vi "Position_TOTAL_R22.vi"(5 "Distance Between \nCameras  (*unit)":sgl=2.5) -> (12 "dX, dY\nLeft Cam":cluster{"X":sgl[], "Y":sgl[]}={"X"=[-5.750775, -4.1849813, -3.081379, -2.0098581, 0.0], "Y"=[7.9585915, 7.9595685, 7.960258, 7.960927, 0.0]}, 13 "Position Valid":bool=TRUE, 14 "Left Camera Real Coordinates":cluster{"X":sgl, "Y":sgl}={"X"=7.9602513, "Y"=5.592073}, 16 "dX, dY\nRight Cam":cluster{"X":sgl[], "Y":sgl[]}={"X"=[-7.3032045, -5.737411, -4.6338086, -3.5622878, -1.5524296], "Y"=[7.2714148, 7.2723923, 7.2730813, 7.273751, -0.68717635]}, 18 "Robot Coordinates":cluster{"X":sgl, "Y":sgl}={"X"=7.616663, "Y"=6.3682876}, 19 "Orietnation\n(current)":sgl=-23.843685 format="%#_13g")   [LabVIEW 2015]
uses:
  <vilib>/Analysis/coordinate.llb/2D Cartesian Coordinate Rotation (Array).vi
  <vilib>/myRIO/Common/Instrument Driver Framework/myRIO v1.0/DIO/vis/myRIO v1.0 Close DIO.vi
  <vilib>/myRIO/Common/Instrument Driver Framework/myRIO v1.0/DIO/vis/myRIO v1.0 Unreserve DIO.vi
  <vilib>/myRIO/Common/Instrument Driver Framework/myRIO v1.0/DIO/vis/myRIO v1.0 Build MUX Configuration DIO.vi
  <vilib>/myRIO/Common/Instrument Driver Framework/myRIO v1.0/Resource Manager/vis/myRIO v1.0 Unreserve Channel List.vi
  <vilib>/myRIO/Common/Instrument Driver Framework/myRIO v1.0/Resource Manager/vis/myRIO v1.0 Create Configuration List.vi
  <vilib>/myRIO/Common/Instrument Driver Framework/myRIO v1.0/Resource Manager/vis/myRIO v1.0 Unreserve Channel.vi
  <vilib>/myRIO/Common/Instrument Driver Framework/myRIO v1.0/Resource Manager/vis/myRIO v1.0 Build Mutex Name.vi
  <vilib>/Instr/_visa.llb/VISA Configure Serial Port (Instr).vi
  <vilib>/myRIO/Common/Instrument Driver Framework/myRIO v1.0/DIO/vis/myRIO v1.0 Shutdown DIO.vi
  <vilib>/Utility/error.llb/Error Cluster From Error Code.vi
  <vilib>/myRIO/Common/Instrument Driver Framework/myRIO v1.0/Resource Manager/vis/myRIO v1.0 Configure IO.vi
  <vilib>/myRIO/Common/Instrument Driver Framework/Utilities/vis/Configuration Manager.vi
  <vilib>/myRIO/Common/Instrument Driver Framework/Utilities/vis/IO Manager.vi
  <vilib>/myRIO/Common/Instrument Driver Framework/myRIO v1.0/myRIO v1.0 Close.vi
  <vilib>/Analysis/NI_AALPro.lvlib
  <vilib>/myRIO/Instrument Drivers/Onboard IO/DIO/DIO.lvlib
panel:
  out "Scale Based\nWeight":sgl format="%#_13g"
  in  "Triangle Based\nWeight":sgl=0.4 format="%#_13g"
  out "Current Cam State - R":T1(ring)=enum."Normal - 5"
  out "Current Cam State - L":T1(ring)=enum."Normal - 5"
  out "Valid Beacon Sets_":bool[](array[boolean])=[TRUE, TRUE, TRUE, TRUE, FALSE]
  in  "Distance Threshold\nRef Triangles (*unit)":sgl=30.0
  out "dA2 4":sgl=9.6935425 format="%#_13g"
  out "dA2 2":sgl=9.6935425 format="%#_13g"
  out "dA2 3":sgl=9.6935425 format="%#_13g"
  out "Beacon Scales - Left":sgl[](array[numeric])=[76.306, 116.841255, 157.35043, 195.67218, 0.0]
  out "Beacon Scales - Right":sgl[](array[numeric])=[76.306, 116.841255, 157.35043, 195.67218, 0.0]
  in  "New Orientation \nThreshold":sgl=10.0
  in  "Moving Average\nWindow Length":u8=2
  out "Current Recovery State -L":enum16{"Generic Sweep", "Recovery Search"}(ring)=enum."Recovery Search"
  out "Current Move Delta - L 2":u16
  out "Next Recovery State - Left":enum16{"Generic Sweep", "Recovery Search"}(ring)=enum."Recovery Search"
  out "Next Recovery State - Right":enum16{"Generic Sweep", "Recovery Search"}(ring)=enum."Recovery Search"
  out "Current Recovery State - Right":enum16{"Generic Sweep", "Recovery Search"}(ring)=enum."Recovery Search"
  in  "Initial Recovery State  - Right":enum16{"Generic Sweep", "Recovery Search"}(ring)=enum."Recovery Search"
  in  "Initial Recovery State - L":enum16{"Generic Sweep", "Recovery Search"}(ring)=enum."Recovery Search"
  out "Next Tracking State - Right":enum16{"Track", "Reactive Predict", ""}(ring)
  out "Current Tracking State - Right 2":enum16{"Track", "Reactive Predict", ""}(ring)
  in  "Initial Tracking State - Right":enum16{"Track", "Reactive Predict", ""}(ring)
  out "Last Track Angle - R":sgl=98.61328
  out "Next Tracking State - Left":enum16{"Track", "Reactive Predict", ""}(ring)
  in  "Initial Tracking State - Left":enum16{"Track", "Reactive Predict", ""}(ring)
  out "Current Tracking State - Left":enum16{"Track", "Reactive Predict", ""}(ring)
  in  "Timeout to \nEnable Reactive Predict":u16=5
  out "Tracking Timeout\nCount - R":i32
  in  "Tracking Timeout\nThreshold":i32=10
  out "Tracking Timeout\nCount - L":i32
  in  "Search Direction - in - Right":bool=TRUE
  out "Next Main State - Right":T2(ring)=enum."Tracking"
  in  "Recovery Search\nDirection - R":bool
  out "Recovery Mode Count in Right":i32
  out "Frames Processed\nCount - in Right":i32
  out "Recovery Search\nmove Count - Right":u16
  out "Recovery Search\nAttempt Count - Right":u16
  in  "Mounting Offset - Right":sgl=45.0
  in  "Tracking Angle - Right":sgl=98.60307
  in  "Current Servo Position\n- Right":u16
  out "New Data  Flag\nRight Servo":bool
  in  "Track Angle Valid  - Right":bool=TRUE
  out "Current Main State - Right":T2(ring)=enum."Tracking"
  in  "Initial Main State- Right":T2(ring)
  in  "Recovery Search\nDirection - L 2":bool
  in  "Max Recovery Count\n(Recovery Search) 2":u16
  in  "Max Recovery\nSearch Attempts 2":u16
  in  "Image Lock - Right 2":bool
  out "Last Track Angle - L":sgl=87.24609
  in  "Recovery Search\nDirection - L":bool=TRUE
  out "Next Main State - Left":T2(ring)=enum."Tracking"
  out "Current Move Delta - L":u16
  in  "Max Recovery Count\n(Recovery Search)":u16=10
  in  "Max Recovery\nSearch Attempts":u16=3
  out "Recovery Search\nAttempt Count - in - L":u16
  out "Recovery Search\nmove Count - in - L":u16
  in  "Image Lock - Right":bool=TRUE
  out "Recovery Mode Count - in Left":u16
  in  "Middle Beacon\nCoordinates":cluster{"X":sgl, "Y":sgl}={"X"=0.0, "Y"=2.5}
  in  "Min Num Frames\nper Search":i32=2
  in  "Wait Tick Threshold":i32=10
  out "Frames Processed\nCount - in -L":i32
  in  "Maximum Move \nServo Threshold":i16=300
  in  "Minimum Delta \nServo Threshold":i16=3
  in  "Mounting Offset - Left":sgl=-45.0
  in  "Search Step Size":u16=50
  in  "Search Direction - in - L":bool
  in  "Current Servo Position\n- Left":u16
  in  "Tracking Angle - Left":sgl=87.25689
  out "New Data  Flag\nLeft Servo":bool
  in  "Track Angle Valid - Left":bool=TRUE
  in  "Image Lock - Left":bool=TRUE
  in  "Initial Main State - Left":T2(ring)
  out "Current Main State - Left":T2(ring)=enum."Tracking"
  in  "Position Calc\nTimer":u32=100 caption="Position Calc Timer"
  in  "Fetch Input\n(mSec)":u32=20 caption="Update Camera Input\n(mSec)"
  out "Right Data\nInput Flag\n- Internal":bool=TRUE
  in  "Position Calc\nReady":bool
  out "This Servo \nAngle - Right":sgl=98.90625
  in  "Beacon Angles -R":sgl[](array[numeric])=[111.28093, 105.355774, 98.60307, 92.04714, 103.90625]
  in  "Beacon Angles - L":sgl[](array[numeric])=[101.98467, 94.59042, 87.25689, 80.30646, 91.66016]
  in  "Valid Angles -R":bool[](array[boolean])=[TRUE, TRUE, TRUE, TRUE, FALSE]
  in  "Valid Angles - L":bool[](array[boolean])=[TRUE, TRUE, TRUE, TRUE, FALSE]
  out "Left Data\nInput Flag\n- Internal":bool
  in  "Check Shared Var Timer":u32=50 caption="Main Loop\n Timer (ms)"
  out "Left_Flag 2":bool
  out "Right_Flag 2":bool
  out "Beacons Found\n- Left (Bool Array) 2":bool[](array[boolean])=[TRUE, TRUE, TRUE, TRUE, FALSE]
  out "LEFT Beacon Coord - X px (IN) 2":sgl[](array[numeric])=[76.306, 116.841255, 157.35043, 195.67218, 0.0]
  out "LEFT Beacon Position - Y px (IN) 2":sgl[](array[numeric])=[154.30304, 148.59094, 148.39949, 146.94655, 0.0]
  out "This Servo \nAngle - Left":sgl=86.66016
  in  "Compliance Slope":u8=128
  out "deltaMoveServo\n- R":i16
  out "Move Respond - R":bool
  out "Move Respond - L":bool
  out "Last Position":cluster{"X":sgl, "Y":sgl}={"X"=7.6261, "Y"=6.350474}
  out "Last Orientation":sgl=-23.876373
  in  "Distance\nBetween Beacons \n- Tolerance":sgl=0.35 format="%#_13g"
  in  "Distance\nBetween Beacons":sgl=1.0 format="%#_13g"
  out "dT":dbl=143.499
  out "Position Valid\nHistory":bool[](array[boolean])=[TRUE, FALSE, FALSE, TRUE, TRUE, FALSE, TRUE, TRUE, TRUE, TRUE, TRUE, TRUE, FALSE, TRUE, FALSE]
  out "Orientation\nHistory":sgl[](array[numeric])=[-23.876373, 0.0, 0.0, -23.938759, -24.0458, 0.0, -23.14014, -22.504314, -22.596928, -22.90728, -23.237453, -23.75214, 0.0, -23.808718, 0.0]
  out "Robot Coordinates\nHistory":cluster{sgl, sgl}[](array[cluster])=[{7.6261, 6.350474}, {0.0, 0.0}, {0.0, 0.0}, {7.63815, 6.33973}, {7.6316156, 6.322055}, {0.0, 0.0}, {7.6863523, 6.2558875}, {7.688662, 6.2228284}, {7.6736236, 6.2455945}, {7.6880507, 6.2819676}, {7.6893277, 6.3140097}, {7.668109, 6.3330927}, {0.0, 0.0}, {7.6506357, 6.3142757}, {0.0, 0.0}]
  in  "New Position \nThreshold":sgl=1.5
  out "Orientation Avgd":sgl=-23.876373
  in  "History Size":u8=15
  in  "Max Y (arena)":sgl=15.0
  in  "Max X (arena)":sgl=35.0
  in  "New Position\nWeight":sgl=0.7 format="%#_13g"
  in  "Max Std Dev (3)":sgl=0.2 format="%#_13g"
  in  "Max Std Dev (4)":sgl=0.2 format="%#_13g"
  out "Post Filtering\n- Valid Beacons":bool[](array[boolean])=[FALSE, TRUE, TRUE, TRUE, FALSE]
  out "Robot Coordinates - Avgd":cluster{"X":sgl, "Y":sgl}={"X"=7.6261, "Y"=6.350474}
  out "Real Position in Course 2":cluster{"X":dbl[], "Y":dbl[]}(graph)={"X"=[7.626100046018056], "Y"=[6.35047366782369]}
  out "Position \nLock Status":bool=TRUE
  out "Right Camera Real Coordinate":cluster{"X":sgl, "Y":sgl}={"X"=7.2730746, "Y"=7.1445026}
  out "deltaMoveServo\n- L":i16
  in  "Search Step Size\n(deg)":sgl=15.0 format="%#_13g"
  out "Beacons Found\n- Right (Bool Array)":bool[](array[boolean])=[TRUE, TRUE, TRUE, TRUE, FALSE]
  out "RIGHT Beacon Position - Y px (IN)":sgl[](array[numeric])=[153.02994, 149.48933, 150.4864, 150.33003, 0.0]
  out "RIGHT Beacon Coord - X px (IN)":sgl[](array[numeric])=[91.3685, 123.99656, 161.27843, 197.4523, 0.0]
  in  "Right Servo\nID":string="\u0001"
  in  "Servo Comm\nWait Time - (ms)":i32
  in  "Left Servo\nID":string="\u0000"
  out "dT - Comm Loop":u32=19
  in  "Servo Comm\nLoop Time (ms)":i32=20
  in  "close comms":bool
  in  "Max Read\nTx Attempts":u8=3
  in  "Max Write\nTx Attempts":u8=3
  out "Current R (10bit)":u16=696
  out "Servo Moving - R":bool
  out "Servo Moving - L":bool
  out "Current L (10bit)":u16=347
  in  "SERVO ENABLE":bool=TRUE
  out "Move Servo - L":bool
  out "Move Servo - R":bool
  in  "Servo Goal Position\n - Right":u16=695
  in  "Move Servo\nThreshold (deg)":sgl=2.0 format="%#_13g"
  in  "Servo Algorithm\nCycle Time(ms)":i32=25
  in  "Servo Goal Position\n - Left":u16=349
  in  "Current Angle\n - Left (internal)":sgl=86.66016
  in  "Current Angle\n - Right (internal)":sgl=98.90625
  in  "stop":bool
  in  "Num of Beacons (Total)":i8=5
  out "Angle to Pixel Ratios":T3={"Angle to Pixel\nRatio - Horizontal"=0.18125, "Angle to Pixel\nRatio - Vertical"=0.1875} {"Angle to Pixel\nRatio - Vertical" format="%#_13g"; "Angle to Pixel\nRatio - Horizontal" format="%#_13g"}
  in  "Cam AOV Vertical (deg)":sgl=45.0
  in  "Cam AOV Horizontal (deg)":sgl=58.0
  in  "Image Height (px)":sgl=240.0
  in  "Image Width (px)":sgl=320.0
  out "Beacon Coordinates - Left Image":T4={"Beacon Position - X px"=[76.306, 116.841255, 157.35043, 195.67218, 0.0], "Beacon Position - Y px"=[154.30304, 148.59094, 148.39949, 146.94655, 0.0]}
  out "Beacon Coordinates - Right Image":T4={"Beacon Position - X px"=[91.3685, 123.99656, 161.27843, 197.4523, 0.0], "Beacon Position - Y px"=[153.02994, 149.48933, 150.4864, 150.33003, 0.0]}
  out "Distance to LBF":sgl[](array[numeric])=[0.024284193, 0.015691843, 0.008273765, 0.028971607, 0.03291407]
  out "Local Coordinates - Calculated":cluster{sgl[], sgl[]}(graph)={[-2.0384164, -0.70265853, 0.4090246, 1.3811935, 0.0], [9.602626, 8.751521, 8.536832, 8.085801, 0.0]}
  out "Local Coordinates - Rotated":cluster{dbl[], dbl[]}(graph)={[1.5524295802029098, -5.750774735805926, -4.1849814062260675, -3.0813788557258652, -2.009858210562305, 0.0], [0.6871763361707266, 7.9585912385832795, 7.959568450875426, 7.960257859242679, 7.960927027680405, 0.0]}
  out "All Object Coordinates \n- Local - Rotated":cluster{"X":sgl[], "Y":sgl[]}={"X"=[1.5524296, -5.750775, -4.1849813, -3.081379, -2.0098581, 0.0], "Y"=[0.68717635, 7.9585915, 7.9595685, 7.960258, 7.960927, 0.0]}
  out "Local Coordinates - Normalized":cluster{sgl[], dbl[]}(graph)={[1.6977187, -2.0372734, -0.60508364, 0.4043527, 1.3844445, 0.0], [0.0, 9.605212211608887, 8.972328186035156, 8.526259422302246, 8.093157768249512, 0.0]}
  in  "Max Std Dev (5)":sgl=0.2 format="%#_13g"
  out "All Object Coordinates \n- Local":cluster{"X":sgl[], "Y":sgl[]}={"X"=[1.6977187, -2.0372734, -0.60508364, 0.4043527, 1.3844445, 0.0], "Y"=[0.0, 9.605212, 8.972328, 8.526259, 8.093158, 0.0]}
  out "LOCAL\nBeacon Coordinates\nRelative to Robot":cluster{"dX_beacon":sgl[], "dY_beacon":sgl[]}={"dX_beacon"=[-2.0384164, -0.70265853, 0.4090246, 1.3811935, 0.0], "dY_beacon"=[9.602626, 8.751521, 8.536832, 8.085801, 0.0]}
  in  "Real Beacon\n - Coordinates":cluster{"X":dbl[], "Y":dbl[]}={"X"=[0.0, 0.0, 0.0, 0.0, 0.0, 0.0], "Y"=[0.5, 1.5, 2.5, 3.5, 4.5, 0.0]}
  # "POSITION CALCULATION VARIABLES"
  # "OUTPUT VALUES"
  # "CONFIG VALUES"
  # "FILTER CONFIG VALUES"
  # "FEEDBACK INPUT VALUES"
  # "INPUT VALUES"
  # "INTERMEDIATE VALUES"
  # "IMAGE TO ANGLE VARIABLES"
  # "VISION PROCESSEING INPUTS"
  # "Use moving average for previous orientation thresholds"
  # "INPUTS"
  # "CONFIG"
  # "OUTPUT VALUES"
  # "*********************"
  # "unfiltered"
  # "NEW FILTER VALS"
  # "Inter Beacon Distance Filtering"
  # "MOVING AVERAGE\nVARIABLES"
  # "DISTANCE SOURCE WEIGHT"
  # "SERVO CONTROL VARIABLES"
  # "SERVO CONTROL VARIABLES"
  # "CONFIG"
  # "SHARED VARIABLE INPUTS"
  # "LOCAL VARIABLE INPUTS"
  # "INTERNRAL VARIABLES"
  # "SEARCH ROUTINE VARIABLES"
  # "MISC"
  # "SERVO IDs"
  # "CONTROL DELAYS"
  # "COMM LOOP DELAY"
  # "COMM PROTOCOL"
  # "SETTINGS"
  # "Make function of distance^^"
  # "**** only left side starts search\nat previously known good angle"
  # "LEFT SERVO"
  # "RIGHT SERVO"
  # "Main State Machine"
  # "Recovery State Machine"
  # "Current Track Angle Inputs"
  # "Servo Status Inputs"
  # "Main State Machine Inputs"
  # "Recovery State Machine Inputs"
  # "Current Track Angle Inputs"
  # "Servo Status Inputs"
  # "Recovery State Machine Feedback"
  # "Tracking State Machine Inputs"
  # "Tracking State Machine Inputs"
  # "NOTE: Must be 1 bigger than amount of beacons"
  # "NOTE: Must be 1 bigger than amount of beacons"
types:
  T1 = enum16{"Sub - 2", "Sub - 3", "Sub - 4", "Normal - 5"}
  T2 = enum16{"Start Up Search", "Tracking", "Recovery Mode", ""}
  T3 = cluster{"Angle to Pixel\nRatio - Horizontal":sgl, "Angle to Pixel\nRatio - Vertical":sgl}
  T4 = cluster{"Beacon Position - X px":sgl[], "Beacon Position - Y px":sgl[]}
  T5 = cluster{"Tracking Coordinates":cluster{"X":dbl, "Y":dbl}, "Current Valid":bool, "Current State - Out":enum16{"Sub - 2", "Sub - 3", "Sub - 4", "Normal - 5"}}
  T6 = cluster{"Array of Double":dbl[], "Array of Double":dbl[]}
  T7 = typedef "DIO.lvlib/DIO Reference.ctl" = cluster{"myRIO Reference":T8, "DIO Channels List":T12}
  T8 = typedef "myRIO Generic Hardware Reference.ctl" = cluster{"myRIO Model":T9, "myRIO Hardware Reference":T10}
  T9 = typedef "Hardware Version Enum.ctl" = enum16{"Unknown", "myRIO-1900", "myRIO-1950", "roboRIO"}
  T10 = typedef "myRIO v1.0 Reference.ctl" = cluster{"Generic FPGA Reference":T11, "Allow multiple opens":bool}
  T11 = typedef "Generic FPGA Reference.ctl" = refnum<k20>
  T12 = typedef "DIO Channels List.ctl" = T13[]
  T13 = typedef "DIO Channels Enum.ctl" = enum16{"Not Connected", "C/DIO0", "C/DIO1", "C/DIO2", "C/DIO3", "C/DIO4", "C/DIO5", "C/DIO6", "C/DIO7", "A/DIO0", "A/DIO1", "A/DIO2", "A/DIO3", "A/DIO4", "A/DIO5", "A/DIO6", "A/DIO7", "A/DIO8", "A/DIO9", "A/DIO10", "A/DIO11", "A/DIO12", "A/DIO13", "A/DIO14", "A/DIO15", "B/DIO0", "B/DIO1", "B/DIO2", "B/DIO3", "B/DIO4", "B/DIO5", "B/DIO6", "B/DIO7", "B/DIO8", "B/DIO9", "B/DIO10", "B/DIO11", "B/DIO12", "B/DIO13", "B/DIO14", "B/DIO15", "LED0", "LED1", "LED2", "LED3", "Button0", "DIO/DIO0", "DIO/DIO1", "DIO/DIO2", "DIO/DIO3", "DIO/DIO4", "DIO/DIO5", "DIO/DIO6", "DIO/DIO7", "DIO/DIO8", "DIO/DIO9", "SPI/CS0", "SPI/CS1", "SPI/CS2", "SPI/CS3", "LED RADIO (Green)", "LED RADIO (Red)", "LED COMM (Green)", "LED COMM (Red)", "LED MODE (Green)", "LED MODE (Red)"}
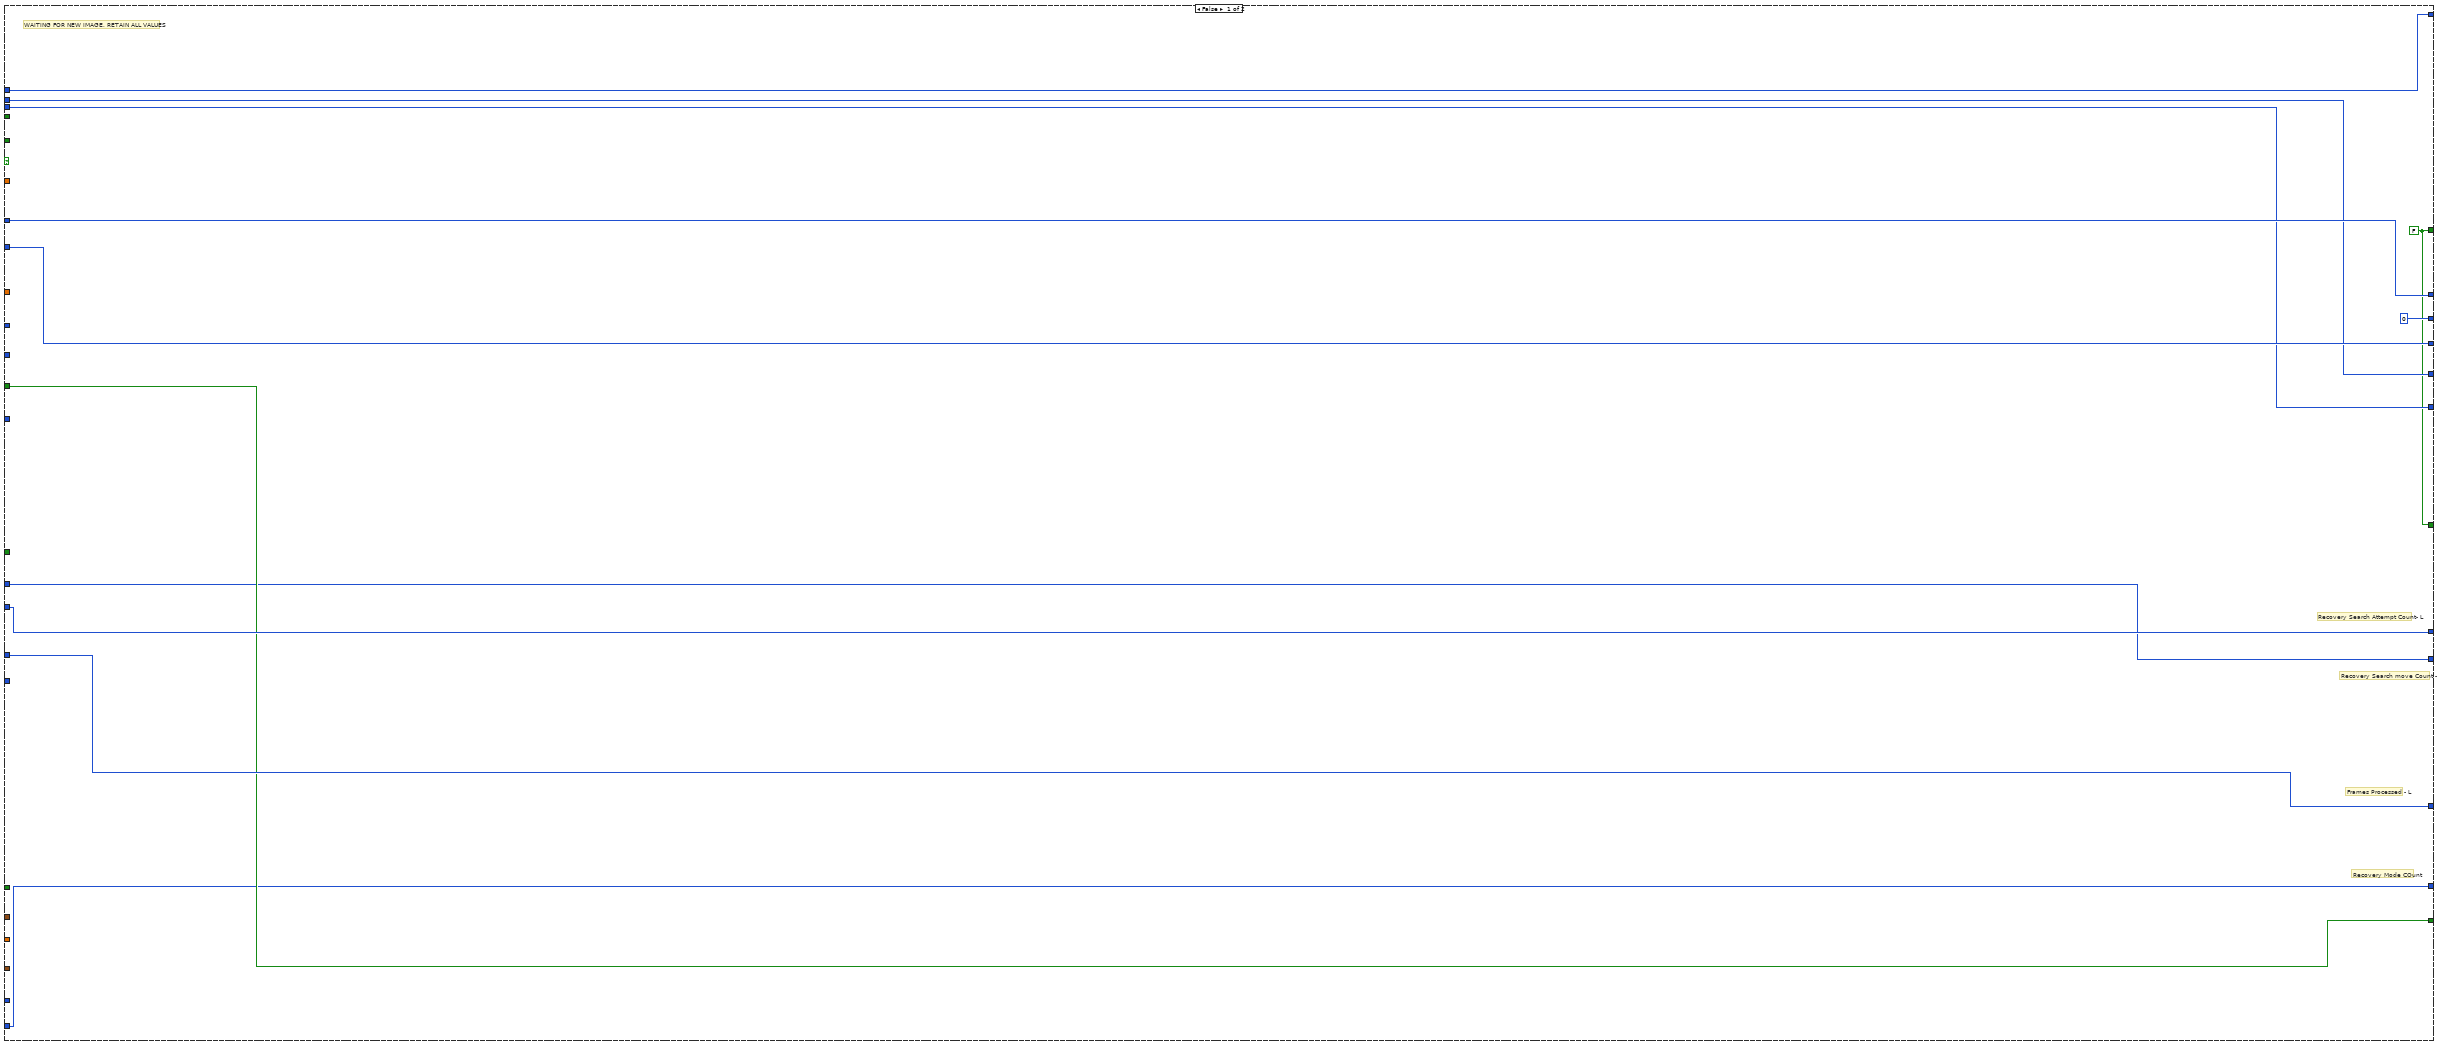
[diagram p2: hidden frame]
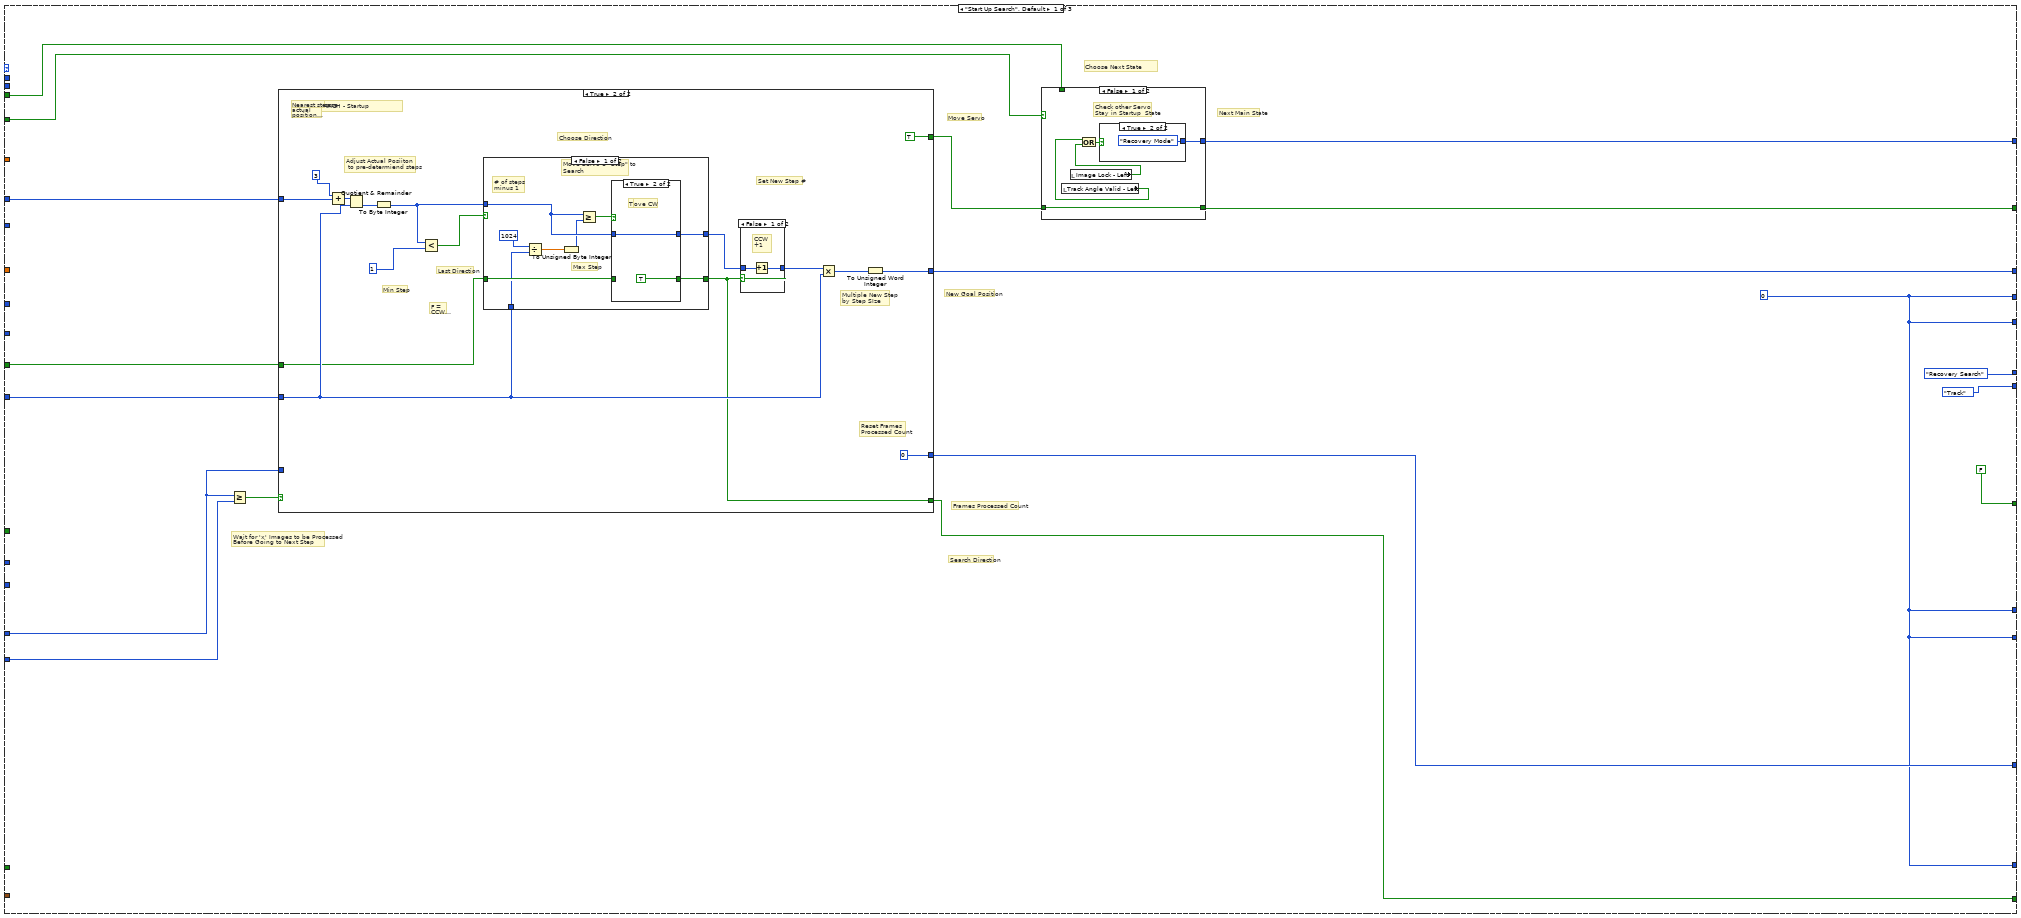
[diagram p3: hidden frame]
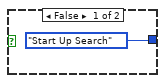
[diagram p4: hidden frame]
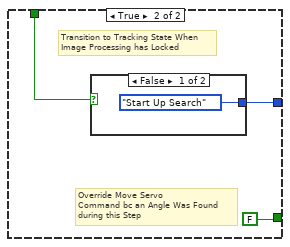
[diagram p5: hidden frame]
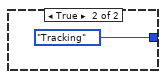
[diagram p6: hidden frame]
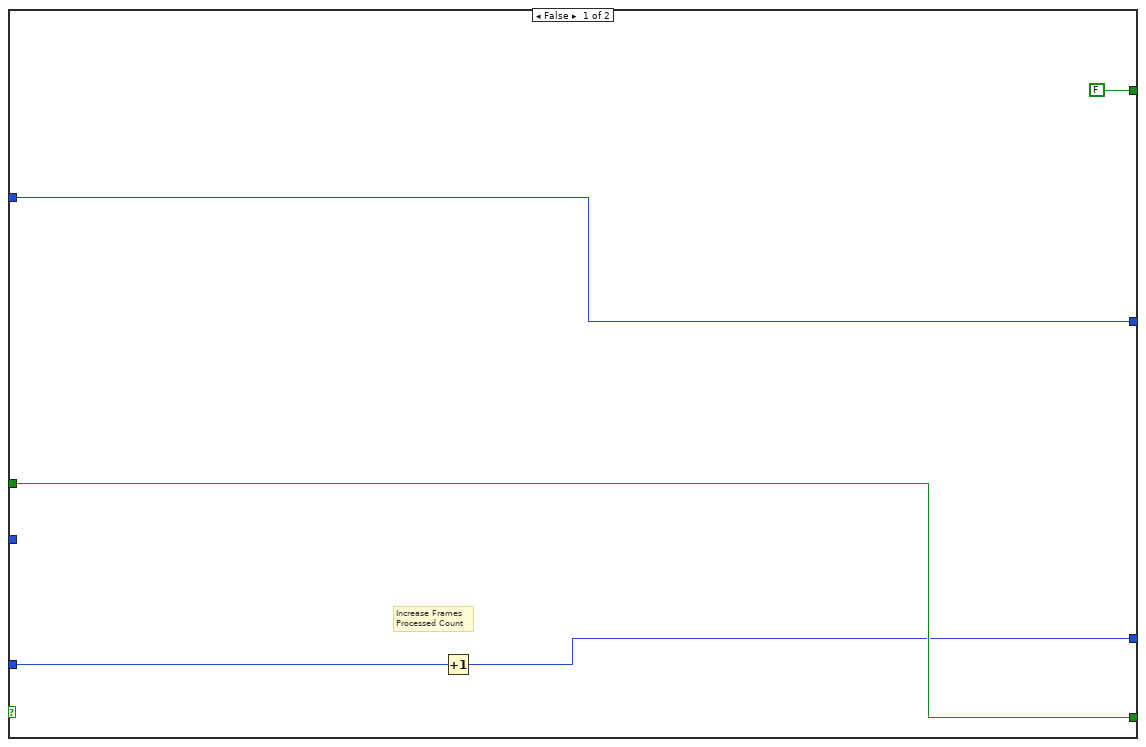
[diagram p7: hidden frame]
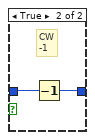
[diagram p8: hidden frame]
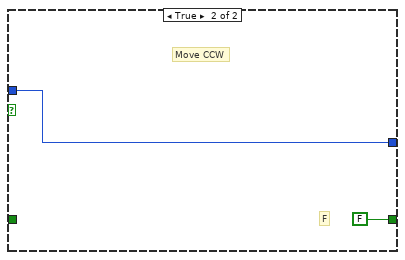
[diagram p10: hidden frame]
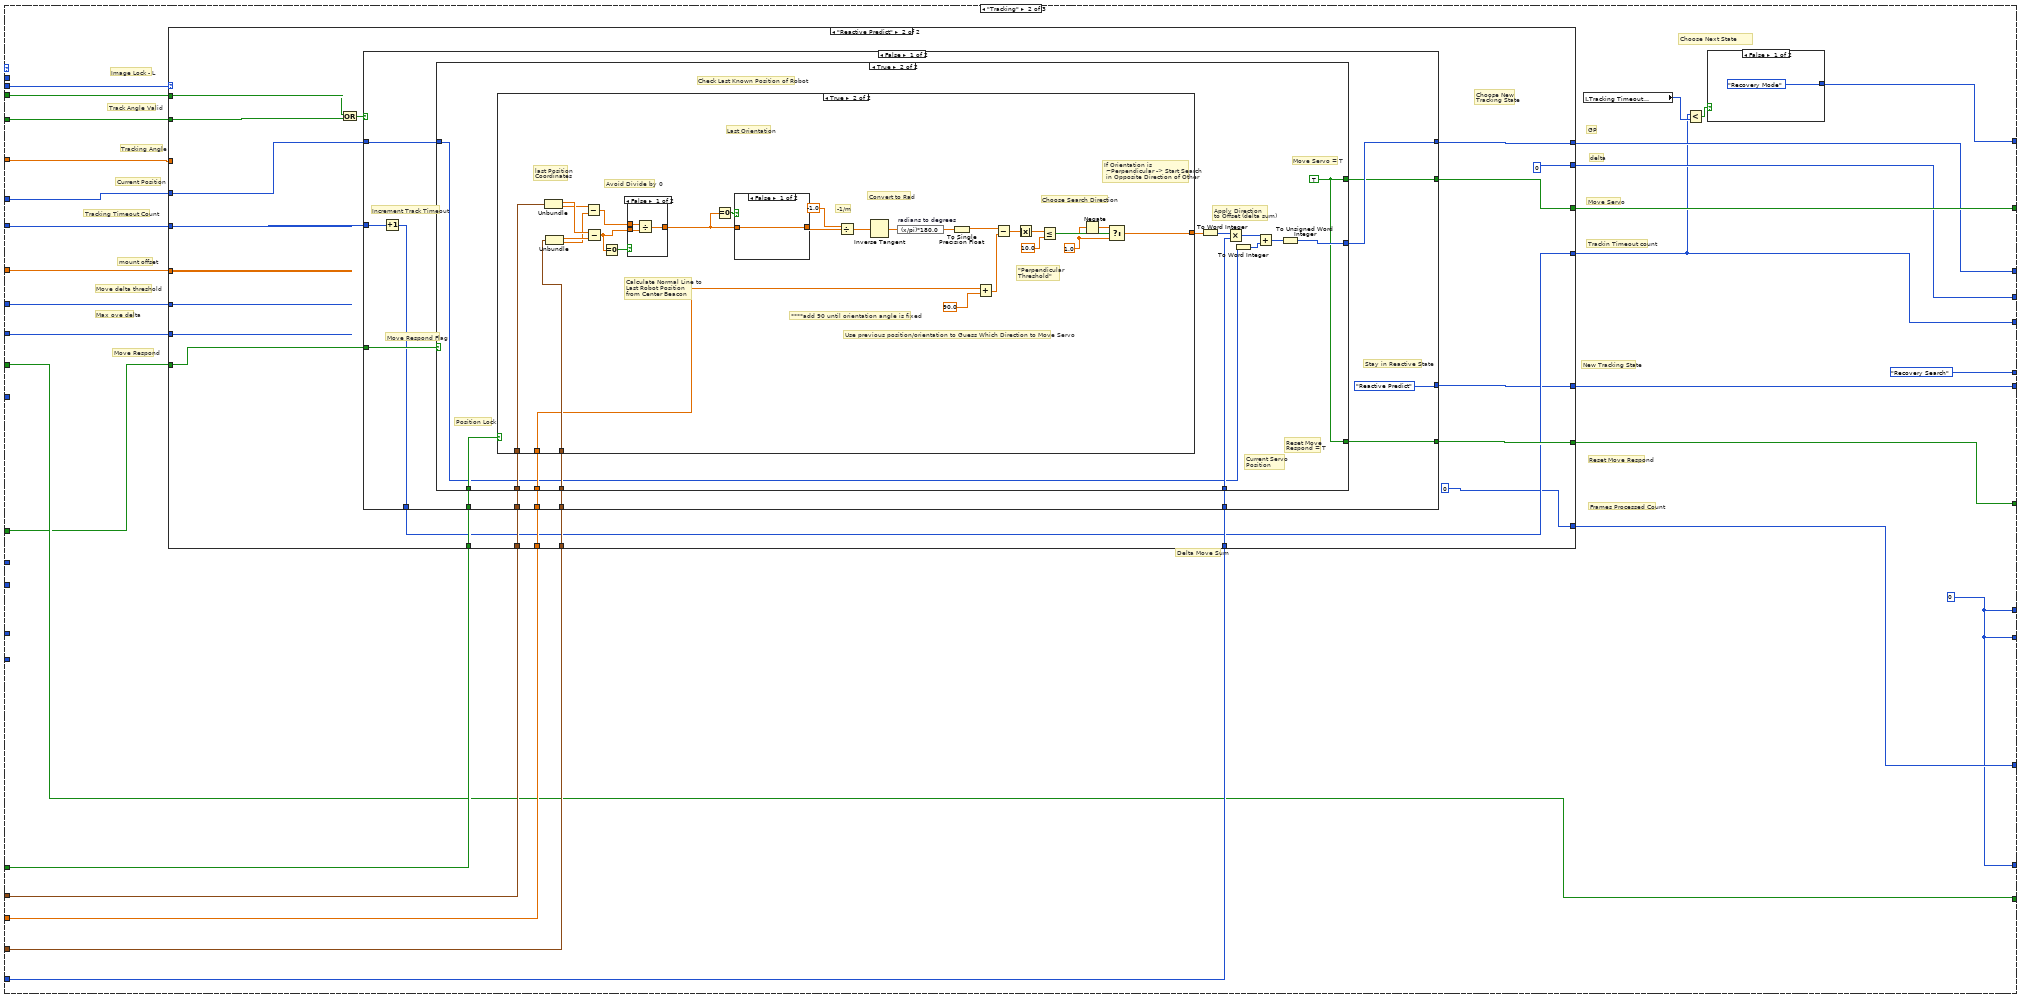
[diagram p11: hidden frame]
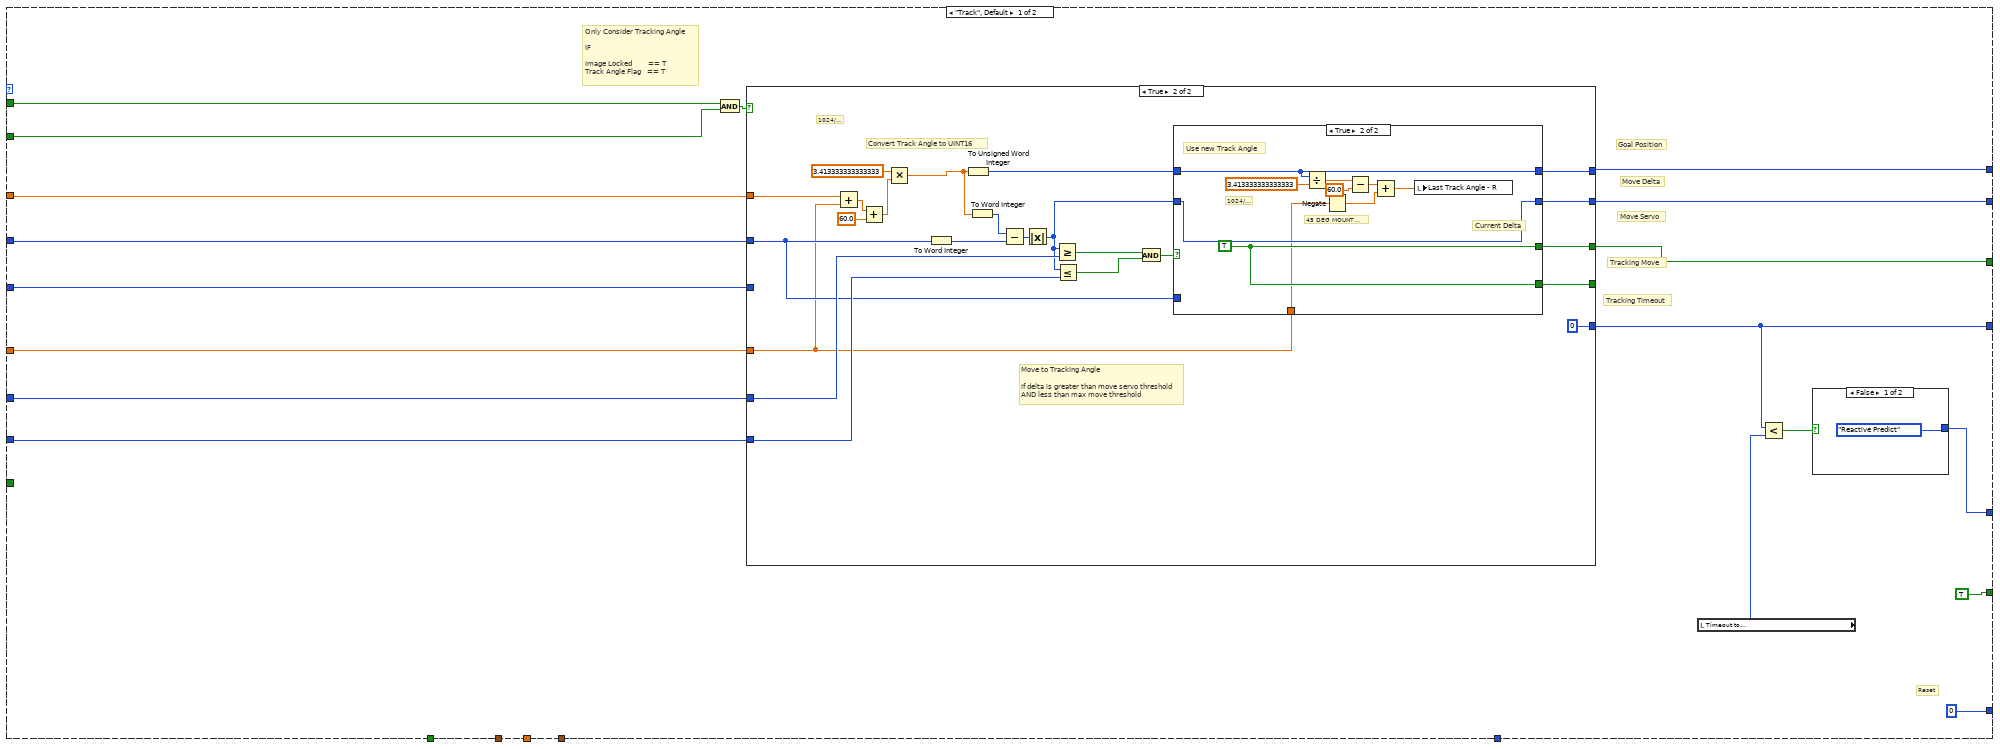
[diagram p12: hidden frame]
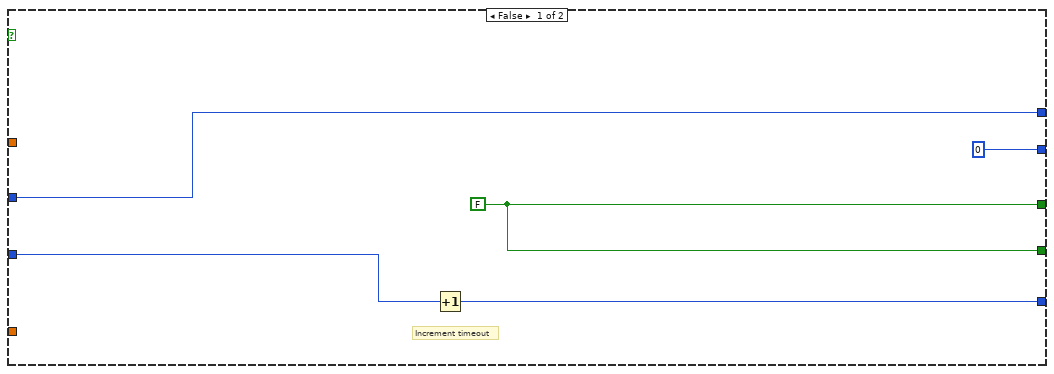
[diagram p13: hidden frame]
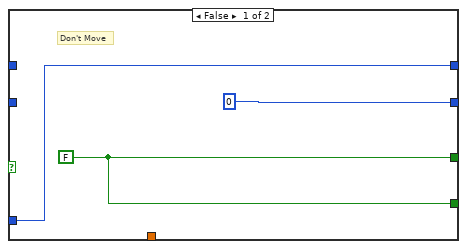
[diagram p14: hidden frame]
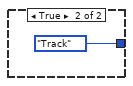
[diagram p15: hidden frame]
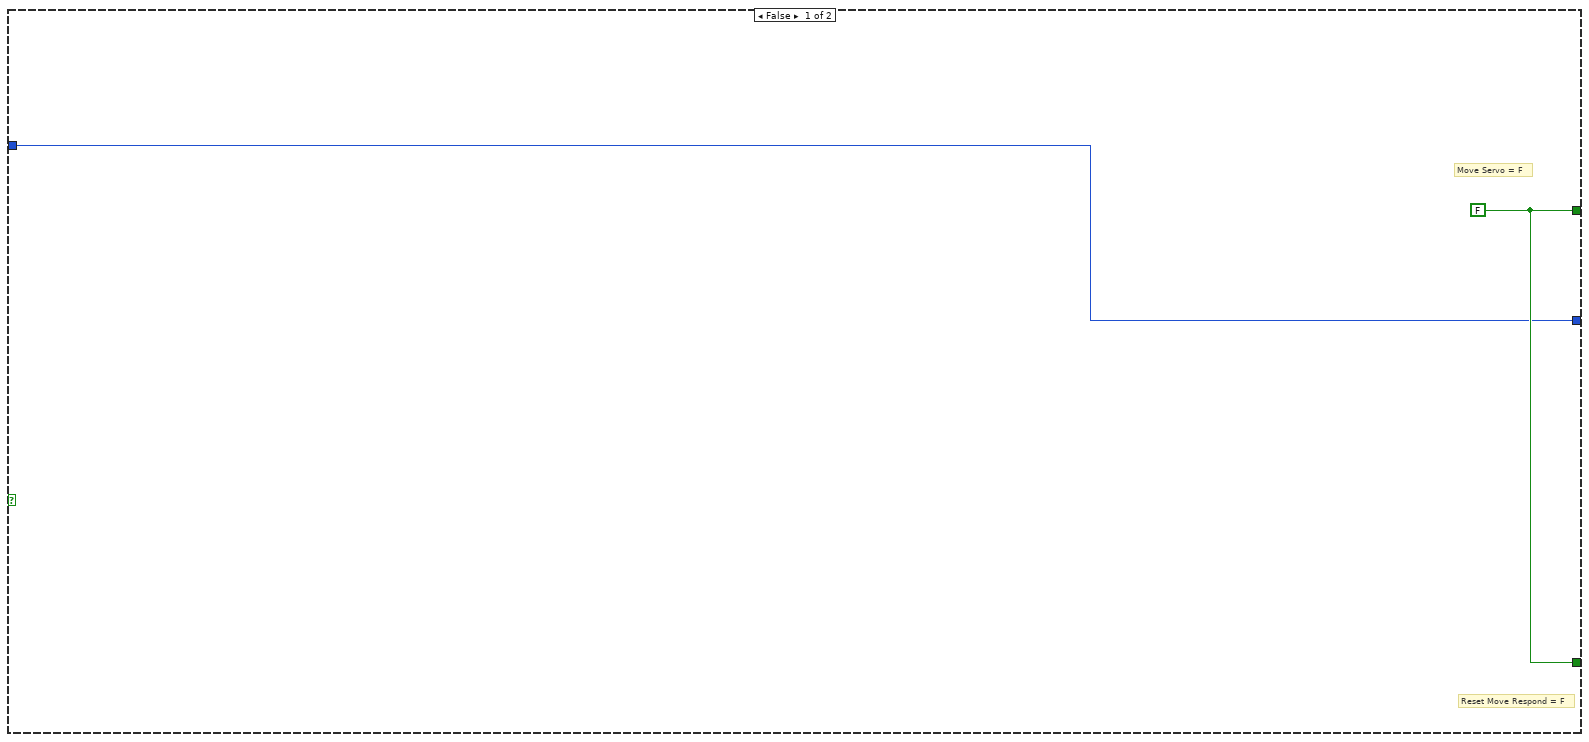
[diagram p16: hidden frame]
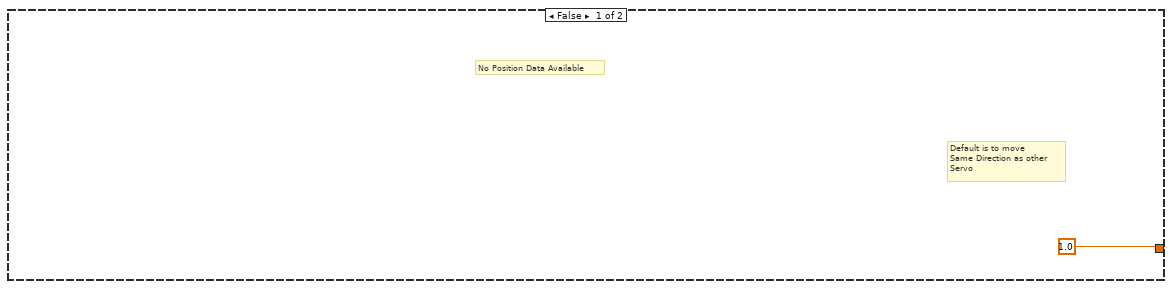
[diagram p17: hidden frame]
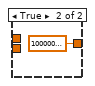
[diagram p18: hidden frame]
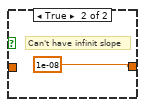
[diagram p19: hidden frame]
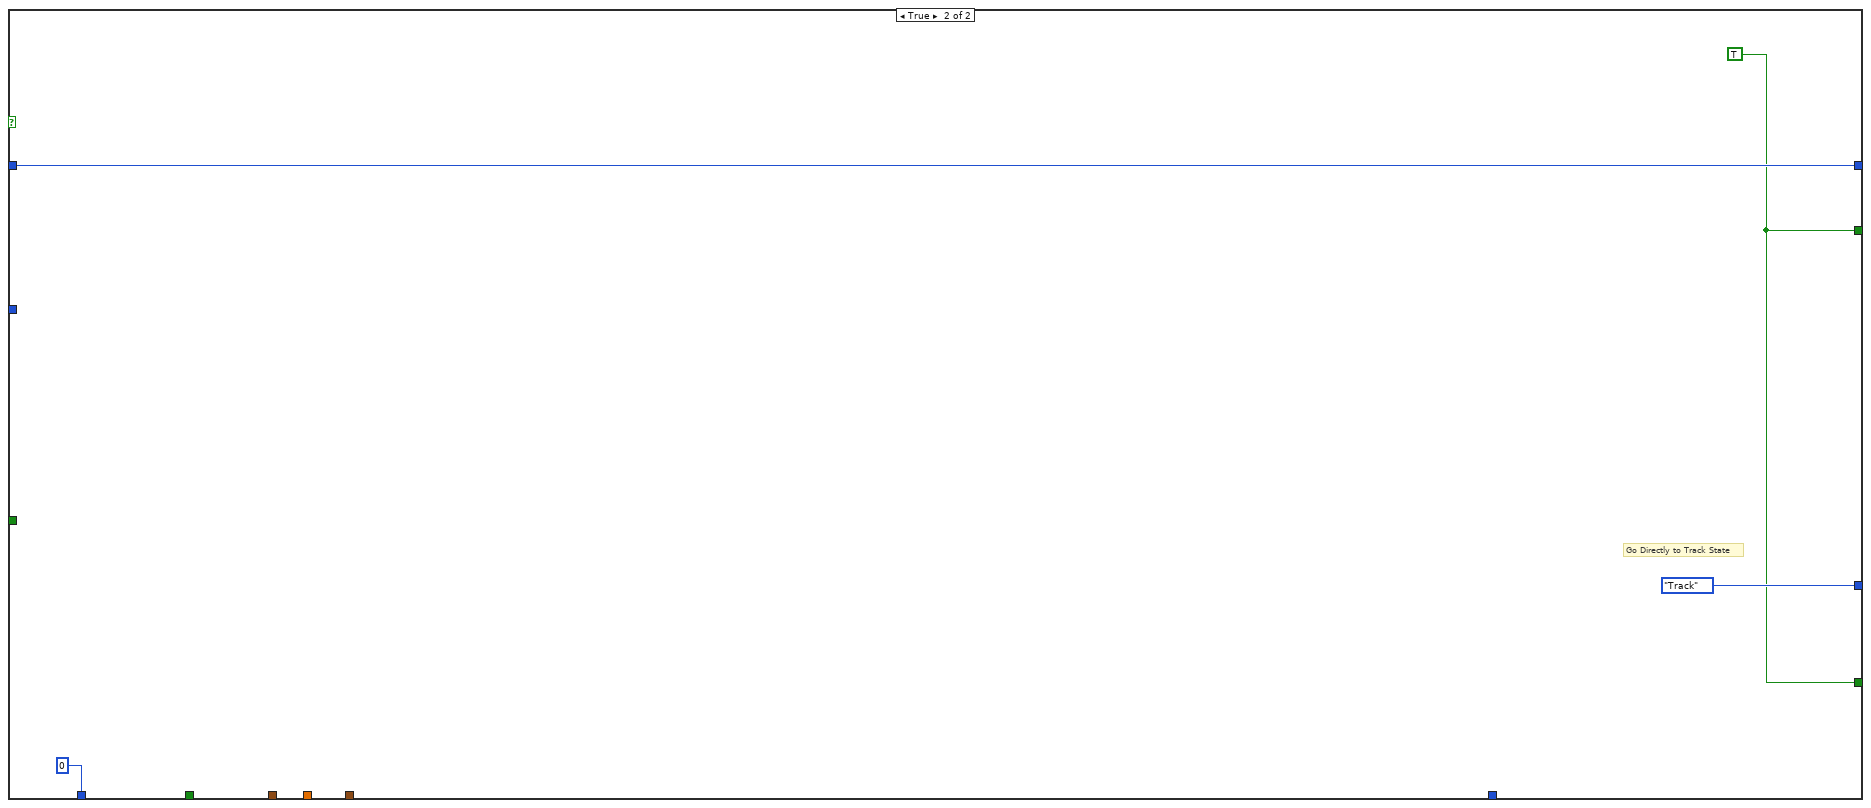
[diagram p20: hidden frame]
diagram:
  (unwired) enum16{"Generic Sweep", "Recovery Search"}."Recovery Search"
  w12 = 0 ("Frames Processed\nCount - in")
  w13 = 0 ("Frames Processed\nCount - in")
  w2 = FALSE
  w34 = sgl 0.0
  # "SERVO CONTROL FLAGS"
  # "***"
  # "Next Tracking State"
  # "Tracking Timeout Count"
  # "Search Direction - L"
  # "Next Recovery State"
  # "Move Respond"
  # "Recovery Mode Count - L"
  # "Delta Move Sum - L"
  # "Wait Tick Count - L"
  # "Frames Processed - L"
  # "Recovery Search move Count - L"
  # "Recovery Search Attempt Count- L"
  # "Next Main State"
  # "Search Direction - L"
  # "Next Recovery State"
  # "INPUTS - Local vars"
  # "Recovery Mode Count - L"
  # "Delta Move Sum - L"
  # "Frames Processed\nLeft"
  # "Move Respond - R"
  # "Initial Search Direction\n- Right"
  # "Move Respond"
  # "Recovery Mode Count - L"
  # "Delta Move Sum - L"
  # "Wait Tick Count - L"
  # "Frames Processed - L"
  # "Recovery Search move Count - L"
  # "Recovery Search Attempt Count- L"
  # "Next Main State"
  # "Settings -- Update in a slow loop"
  # "Recovery Mode Count - L"
  # "Delta Move Sum - L"
  # "Frames Processed\nLeft"
  # "Move Respond - L"
  # "Replace these with\nconstants"
  # "Initial Search Direction\n- Left"
  # "Read Inputs when Available"
  # "# of Physical Beacons"
  # "Right Data Internal Falg"
  # "Left Data Internal Falg"
  # "Initialize Shift Arrays"
  # "Robot Position (cluster)\nShift Array"
  # "Robot Position (cluster)\nShift Array"
  # "Position Valid Shift Array"
  # "Orientation Shift Array"
  # "Position Valid Shift Array"
  # "Orientation Shift Array"
  # "Servo Communication (to Servo- UART))"
  # "Internal Local Variables"
  # "Servo Control Logic"
  # "Local Variables"
  # "Images to Robot Position Calculation Process"
  # "SERVO MOTOR CONTROL"
  # "SERVO MOTOR CONTROL"
  n1 = Divide(x="Cam AOV Horizontal (deg)", y="Image Width (px)") -> (x/y=w25:sgl)
  n2 = Divide(x="Cam AOV Vertical (deg)", y="Image Height (px)") -> (x/y=w26:sgl)
  n3 = Bundle(w25, w26) -> (w20:cluster{sgl, sgl})  [unwired: 1 in]
  "Angle to Pixel Ratios" <- w20
  n4 = disable-structure shown="Disabled" {
    frame Disabled {
      # "Always Read Incoming Flags & Store"
      n5 = while {
        tunnel: "Check Shared Var Timer" -> [w46]
        stop <- FALSE stop-if-true
        n6 = shared-variable "myRIO-1900\\Lib1.lvlib\\RIGHT_FLAG"() -> (→"Right_Flag 2":bool)  [unwired: 1 in, 1 out]
        n7 = shared-variable "myRIO-1900\\Lib1.lvlib\\Left_Flag"() -> (→"Left_Flag 2":bool)  [unwired: 1 in, 1 out]
        n8 = call "Wait8"("Count(mSec)"=w46) -> ()  [unwired: 1 out]
      }
    }
    frame Enabled {
    }
  }
  n9 = while {
    shift-right: [w55] -> _
    shift-left: w2 -> [w60]
    shift-right: [w54] -> _
    shift-left: w2 -> [w58]
    tunnel: w20 -> [w56]
    tunnel: "Num of Beacons (Total)" -> [w57]
    stop <- FALSE stop-if-true
    # "Wait for Both Internal Flags"
    n10 = call "Wait6"("Count(mSec)"="Fetch Input\n(mSec)") -> ()  [unwired: 1 out]
    n11 = shared-variable "RT myRIO Target - Overlord\\Localization_Variables_r0.lvlib\\RIGHT_FLAG"() -> (w51:bool)  [unwired: 1 in, 1 out]
    n12 = shared-variable "RT myRIO Target - Overlord\\Localization_Variables_r0.lvlib\\Left_Flag"() -> (w52:bool)  [unwired: 1 in, 1 out]
    n13 = case shown="True" w51 {
      tunnel: w57 -> [_ w79]
      tunnel: w56 -> [_ w77]
      tunnel: [w61 w67] -> w49
      tunnel: w58 -> [w61 _]
      frame False {
        # "Don't Update Servo Position\nbc we're waiting on new Data to\ncome in and the servo position\nwas set at the previous set of data"
      }
      frame True {
        w67 = TRUE
        # "Store Values"
        # "Raise Internal Flag"
        # "If New Data Available"
        # "From Shift Reg"
        # "Perforrm Indivudual Angle Calculation"
        # "Pull Down Individual Flag"
        n14 = shared-variable "RT myRIO Target - Overlord\\Localization_Variables_r0.lvlib\\RIGHT_BEACON_X_array"() -> (w73:dbl[])  [unwired: 1 in, 1 out]
        "RIGHT Beacon Coord - X px (IN)" <- w73
        n15 = shared-variable "RT myRIO Target - Overlord\\Localization_Variables_r0.lvlib\\Image Lock - R"() -> (w68:bool)  [unwired: 1 in, 1 out]
        n16 = shared-variable "RT myRIO Target - Overlord\\Localization_Variables_r0.lvlib\\RIGHT_BEACON_Scales"() -> (→"Beacon Scales - Right":sgl[])  [unwired: 1 in, 1 out]
        n17 = shared-variable "RT myRIO Target - Overlord\\Localization_Variables_r0.lvlib\\Info - Right"() -> (w65:T5)  [unwired: 1 in, 1 out]
        n18 = shared-variable "RT myRIO Target - Overlord\\Localization_Variables_r0.lvlib\\RIGHT_BEACON_Y_array"() -> (w72:dbl[])  [unwired: 1 in, 1 out]
        "RIGHT Beacon Position - Y px (IN)" <- w72
        n19 = shared-variable "RT myRIO Target - Overlord\\Localization_Variables_r0.lvlib\\RIGHT_BEACON_BOOL_array"() -> (w71:bool[])  [unwired: 1 in, 1 out]
        "Beacons Found\n- Right (Bool Array)" <- w71
        n20 = Unbundle By Name(w65) -> ("Tracking Coordinates"=w64:cluster{"X":dbl, "Y":dbl}, "Current Valid"=w63:bool, "Current State - Out"=→"Current Cam State - R":T1)
        n21 = local write "Image Lock - Right"(w68) -> ()
        n22 = Bundle("Array of Double"=w73, "Array of Double"=w72) -> (w70:T6)  [unwired: 1 in]
        "Beacon Coordinates - Right Image" <- w70
        n23 = shared-variable "RT myRIO Target - Overlord\\Localization_Variables_r0.lvlib\\Right Servo Angle_Image"() -> (w69:dbl)  [unwired: 1 in, 1 out]
        "This Servo \nAngle - Right" <- w69
        n24 = shared-variable "RT myRIO Target - Overlord\\Localization_Variables_r0.lvlib\\RIGHT_FLAG"(FALSE) -> ()  [unwired: 1 in, 1 out]
        n25 = feedback #1() -> (w81:sgl[])  [unwired: 1 in]
        n26 = feedback #2() -> (w80:bool[])  [unwired: 1 in]
        n27 = call "Angle Calc_Individual Process R4.vi"("Angle to Pixel Ratios"=w77, "Previous Angles"=w81, "Num of Beacons"=w79, "Beacon Coordinates - Image"=w70, "Current Servo Angle"=w69, "Beacons Found (Bool Array)"=w71, "Previous Valid Angles"=w80, "Tracking Coordinates"=w64) -> ("Servo Goal Angle"=w76:sgl, "Valid Beacons (Bool Array)\nPosition Calc"=w75:bool[], "Angle Of Beacons \nRelative to Robot"=w74:sgl[])  [unwired: 4 in, 1 out]
        n28 = feedback-in #1(w74) -> ()
        n29 = feedback-in #2(w75) -> ()
        n30 = local write "Beacon Angles -R"(w74) -> ()
        n31 = local write "Tracking Angle - Right"(w76) -> ()
        n32 = local write "Valid Angles -R"(w75) -> ()
        n33 = local write "Track Angle Valid  - Right"(w63) -> ()
        n34 = local write "New Data  Flag\nRight Servo"(w67) -> ()
      }
    }
    "Right Data\nInput Flag\n- Internal" <- w49
    n35 = case shown="True" w52 {
      tunnel: [w82 w88] -> w48
      tunnel: w60 -> [w82 _]
      tunnel: w56 -> [_ w92]
      tunnel: w57 -> [_ w91]
      frame False {
        # "Don't Update Servo Position\nbc we're waiting on new Data to\ncome in and the servo position\nwas set at the previous set of data"
      }
      frame True {
        w88 = TRUE
        # "Store Values"
        # "Raise Internal Flag"
        # "If New Data Available"
        # "Perforrm Indivudual Angle Calculation"
        # "Pull Down Individual Flag"
        n36 = shared-variable ".\\Localization_Variables_r0.lvlib\\LEFT_BEACON_X_array"() -> (w98:dbl[])  [unwired: 1 in, 1 out]
        "LEFT Beacon Coord - X px (IN) 2" <- w98
        n37 = shared-variable "RT myRIO Target - Overlord\\Localization_Variables_r0.lvlib\\LEFT_BEACON_Scales"() -> (→"Beacon Scales - Left":sgl[])  [unwired: 1 in, 1 out]
        n38 = shared-variable "RT myRIO Target - Overlord\\Localization_Variables_r0.lvlib\\LEFT_BEACON_Y_array"() -> (w99:dbl[])  [unwired: 1 in, 1 out]
        "LEFT Beacon Position - Y px (IN) 2" <- w99
        n39 = shared-variable "RT myRIO Target - Overlord\\Localization_Variables_r0.lvlib\\LEFT_BEACON_BOOL_array"() -> (w100:bool[])  [unwired: 1 in, 1 out]
        "Beacons Found\n- Left (Bool Array) 2" <- w100
        n40 = shared-variable "RT myRIO Target - Overlord\\Localization_Variables_r0.lvlib\\Image Lock - L"() -> (w89:bool)  [unwired: 1 in, 1 out]
        n41 = shared-variable "RT myRIO Target - Overlord\\Localization_Variables_r0.lvlib\\Info - Left"() -> (w86:T5)  [unwired: 1 in, 1 out]
        n42 = Unbundle By Name(w86) -> ("Tracking Coordinates"=w85:cluster{"X":dbl, "Y":dbl}, "Current Valid"=w84:bool, "Current State - Out"=→"Current Cam State - L":T1)
        n43 = local write "Image Lock - Left"(w89) -> ()
        n44 = Bundle("Array of Double"=w98, "Array of Double"=w99) -> (w96:T6)  [unwired: 1 in]
        "Beacon Coordinates - Left Image" <- w96
        n45 = shared-variable "RT myRIO Target - Overlord\\Localization_Variables_r0.lvlib\\Left Servo Angle_Image"() -> (w90:dbl)  [unwired: 1 in, 1 out]
        "This Servo \nAngle - Left" <- w90
        n46 = shared-variable "RT myRIO Target - Overlord\\Localization_Variables_r0.lvlib\\Left_Flag"(FALSE) -> ()  [unwired: 1 in, 1 out]
        n47 = feedback #3() -> (w102:sgl[])  [unwired: 1 in]
        n48 = feedback #4() -> (w101:bool[])  [unwired: 1 in]
        n49 = call "Angle Calc_Individual Process R4.vi"("Angle to Pixel Ratios"=w92, "Previous Angles"=w102, "Num of Beacons"=w91, "Beacon Coordinates - Image"=w96, "Current Servo Angle"=w90, "Beacons Found (Bool Array)"=w100, "Previous Valid Angles"=w101, "Tracking Coordinates"=w85) -> ("Servo Goal Angle"=w95:sgl, "Valid Beacons (Bool Array)\nPosition Calc"=w94:bool[], "Angle Of Beacons \nRelative to Robot"=w93:sgl[])  [unwired: 4 in, 1 out]
        n50 = feedback-in #3(w93) -> ()
        n51 = feedback-in #4(w94) -> ()
        n52 = local write "Beacon Angles - L"(w93) -> ()
        n53 = local write "Valid Angles - L"(w94) -> ()
        n54 = local write "Tracking Angle - Left"(w95) -> ()
        n55 = local write "Track Angle Valid - Left"(w84) -> ()
        n56 = local write "New Data  Flag\nLeft Servo"(w88) -> ()
      }
    }
    "Left Data\nInput Flag\n- Internal" <- w48
    n57 = And(x=w48, y=w49) -> (x .and. y?=w59:bool)
    n58 = case shown="True" w59 {
      selector: w59 -> [_ w105]
      tunnel: w48 -> [w104 _]
      tunnel: [w104 w106] -> w55
      tunnel: [w103 w106] -> w54
      tunnel: w49 -> [w103 _]
      frame False {
      }
      frame True {
        w106 = FALSE
        # "Reset Internal Data Flags"
        # "Position Data\nReady Enabled"
        n59 = local write "Position Calc\nReady"(w105) -> ()
      }
    }
  }
  n60 = Bundle(w34, w34) -> (w37:cluster{sgl, sgl})  [unwired: 1 in]
  n61 = Initialize Array(w34, "History Size") -> (w32:sgl[])
  n62 = Initialize Array(w37, "History Size") -> (w33:cluster{sgl, sgl}[])
  n63 = Initialize Array(FALSE, "History Size") -> (w31:bool[])
  n64 = call "Tick Count4"() -> ("Tick Count(uSec)"=w30:u32)
  n65 = while {
    shift-right: [w117] -> _
    shift-left: w32 -> [w114]
    shift-right: [w116] -> _
    shift-left: w31 -> [w115]
    shift-right: [w118] -> _
    shift-left: w33 -> [w109]
    shift-right: [w110] -> _
    shift-left: w30 -> [w111]
    stop <- "stop" stop-if-true
    n66 = call "Wait5"("Count(mSec)"="Position Calc\nTimer") -> ()  [unwired: 1 out]
    n67 = case shown="True" "Position Calc\nReady" {
      selector: "Position Calc\nReady" -> [_ w184]
      tunnel: w109 -> [_ w206]
      tunnel: w109 -> [w127 w200]
      tunnel: w114 -> [w129 w199]
      tunnel: w115 -> [w128 w198]
      tunnel: [w129 w205] -> w117
      tunnel: [w128 w203] -> w116
      tunnel: [w127 w204] -> w118
      tunnel: w115 -> [_ w197]
      tunnel: w114 -> [_ w196]
      tunnel: [w126 w191] -> w112
      tunnel: w111 -> [_ w191]
      tunnel: [FALSE TRUE] -> w113
      tunnel: w109 -> [_ w186]
      frame False {
        n68 = call "Tick Count5"() -> ("Tick Count(uSec)"=w126:u32)
      }
      frame True {
        # "dY"
        # "dX"
        # "Valid"
        # "Find Local Coordinates"
        # "Valid COunt"
        # "Make sure 2+ Data Sets are Still available"
        # "Check 1st element\nwith rest of elements"
        # "Make Sure all Pointed \nIn Same Direction"
        # "For Each Valid Beacon\nCalculate Distance from Each Camera to Each Beacon"
        # "Find Common Beacons\nAmong Cameras"
        # "Currently will only\ncalculate position if 2+ \nbeacons are available \nfrom both cameras"
        # "System is in Normal (long range) State"
        # "Average Both Data Sets"
        # "Estimate Distance for each Available Beacon Angle\nPER Camera, indivduallly"
        # "At least 2+ Avaialbe"
        # "CALCULATE AVERAGE ORIENTATION"
        # "Update Outputs\nif Current Calc is Invalid\n(shouldn't matter)"
        # "Estimate Orienation Based on Previous Position"
        # "****# of previous in history that must be true\nin order for position to be considered \"locked\""
        # "New Position is Valid if both \nOrientation and Positions\nis within range of previous"
        # "Robot Position\n Shift Array"
        # "Position Valid Shift Array"
        # "Orientation Shift Array"
        # "Orientation Value"
        # "Shift & Insert Current Position Valid"
        # "Position Valid\n(orientation)"
        # "Position Valid\n(position)"
        # "Update Shift Registers"
        # "Shift & Insert Current Calculated Orientation"
        # "Shift & Insert Current Robot Position"
        # "UPDATE FINAL OUTPUT\n VALUES"
        n69 = local read "Num of Beacons (Total)"() -> (w167:i8)
        n70 = Not(x=w184) -> (.not. x?=w185:bool)
        n71 = local write "Position Calc\nReady"(w185) -> ()
        n72 = disable-structure shown="Disabled" {
          frame Disabled {
            w207 = T1."Normal - 5" ("Initial State")
            # "***********do for both"
            # "sTATE"
            n73 = local read "Current Cam State - L"() -> (w211:T1)
            n74 = local read "Current Cam State - R"() -> (w210:T1)
            n75 = Equal?(x=w211, y=w207) -> (x = y?=w209:bool)
            n76 = Equal?(x=w210, y=w207) -> (x = y?=w208:bool)
            n77 = And(x=w209, y=w208) -> ()  [unwired: 1 out]
          }
          frame Enabled {
          }
        }
        n78 = local read "Beacon Scales - Left"() -> (w173:sgl[])
        n79 = local read "Beacon Scales - Right"() -> (w170:sgl[])
        n80 = for {
          N: w167 -> [_]
          tunnel: "Valid Angles - L" -> [w340] mode=indexing
          tunnel: "Beacon Angles - L" -> [w349] mode=indexing
          tunnel: w173 -> [w350] mode=indexing
          tunnel: "Valid Angles -R" -> [w339] mode=indexing
          tunnel: "Beacon Angles -R" -> [w348] mode=indexing
          tunnel: w170 -> [w347] mode=indexing
          tunnel: "Distance Between \nCameras  (*unit)" -> [w346]
          tunnel: [w338] -> w164 mode=indexing
          tunnel: [w337] -> w163 mode=indexing
          tunnel: [w336] -> w165 mode=indexing
          # "dY"
          # "dX"
          # "Valid"
          # "If Both Cameras are using Same Beacon Data,\nAverage the 2 independently esitmated positions"
          # "dY"
          # "dX"
          # "dY"
          # "dX"
          n81 = case shown="True" w340 {
            tunnel: w349 -> [_ w427]
            tunnel: [w414 w418] -> w344
            tunnel: [w414 w419] -> w343
            tunnel: w350 -> [_ w415]
            frame False {
              w414 = sgl 0.0
              # "Current Data Set Was Not Valid\nFill with 0\nWill not be used later"
            }
            frame True {
              # "Estimate Distance"
              # "Negate dX if A2>90"
              # "Find LOCAL Coordinate of Each Beacon"
              # "Current - Valid Data Set"
              n82 = call "Scaling and Mapping"("Signals"=w415) -> ("Scaled Signals"=w416:dynamicdata)  [unwired: 9 in, 1 out]
              n83 = To Single Precision Float(number=w416) -> (single precision float=w417:sgl)
              n84 = Less?(x=w427, y=sgl 90.0) -> (x < y?=w429:bool)
              n85 = case shown="False" w429 {
                tunnel: w427 -> [w436 w438]
                tunnel: [w434 w439] -> w426
                tunnel: [FALSE TRUE] -> w421
                frame False {
                  # "Negative Y"
                  # "A2 is > 90"
                  n86 = Subtract(x=w436, y=sgl 90.0) -> (x-y=w434:sgl)
                }
                frame True {
                  # "Positive Y"
                  # "A2 is < 90"
                  n87 = Subtract(x=sgl 90.0, y=w438) -> (x-y=w439:sgl)
                }
              }
              "dA2 2" <- w426
              n88 = expression code="(x/180.0)*pi" "degrees to radians"(w426) -> (w424:sgl)
              n89 = expression code="(x/180.0)*pi" "degrees to radians"(w426) -> (w425:sgl)
              n90 = Cosine(x=w424) -> (cos(x)=w422:sgl)
              n91 = Sine(x=w425) -> (sin(x)=w423:sgl)
              n92 = Multiply(x=w417, y=w422) -> (x*y=w419:sgl)
              n93 = Multiply(x=w417, y=w423) -> (x*y=w420:sgl)
              n94 = case shown="True" w421 {
                tunnel: w420 -> [w431 w432]
                tunnel: [w430 w432] -> w418
                frame False {
                  n95 = Negate(x=w431) -> (-x=w430:sgl)
                }
                frame True {
                }
              }
            }
          }
          n96 = case shown="True" w339 {
            tunnel: w348 -> [_ w400]
            tunnel: [w385 w387] -> w342
            tunnel: [w385 w386] -> w341
            tunnel: w347 -> [_ w392]
            tunnel: w346 -> [_ w389]
            frame False {
              w385 = sgl 0.0
              # "Current Data Set Was Not Valid\nFill with 0\nWill not be used later"
            }
            frame True {
              # "Add delta for\nRIGHT camera ONLY"
              # "Estimate Distance"
              # "Negate dX if A2>90"
              # "Find LOCAL Coordinate of Each Beacon"
              # "Current - Valid Data Set"
              n97 = call "Scaling and Mapping2"("Signals"=w392) -> ("Scaled Signals"=w391:dynamicdata)  [unwired: 9 in, 1 out]
              n98 = To Single Precision Float(number=w391) -> (single precision float=w390:sgl)
              n99 = Less?(x=w400, y=sgl 90.0) -> (x < y?=w402:bool)
              n100 = case shown="False" w402 {
                tunnel: w400 -> [w409 w411]
                tunnel: [w407 w412] -> w399
                tunnel: [FALSE TRUE] -> w394
                frame False {
                  # "Negative Y"
                  # "A2 is > 90"
                  n101 = Subtract(x=w409, y=sgl 90.0) -> (x-y=w407:sgl)
                }
                frame True {
                  # "Positive Y"
                  # "A2 is < 90"
                  n102 = Subtract(x=sgl 90.0, y=w411) -> (x-y=w412:sgl)
                }
              }
              "dA2 3" <- w399
              n103 = expression code="(x/180.0)*pi" "degrees to radians"(w399) -> (w397:sgl)
              n104 = expression code="(x/180.0)*pi" "degrees to radians"(w399) -> (w398:sgl)
              n105 = Cosine(x=w397) -> (cos(x)=w395:sgl)
              n106 = Sine(x=w398) -> (sin(x)=w396:sgl)
              n107 = Multiply(x=w390, y=w395) -> (x*y=w386:sgl)
              n108 = Multiply(x=w390, y=w396) -> (x*y=w393:sgl)
              n109 = case shown="True" w394 {
                tunnel: w393 -> [w404 w405]
                tunnel: [w403 w405] -> w388
                frame False {
                  n110 = Negate(x=w404) -> (-x=w403:sgl)
                }
                frame True {
                }
              }
              n111 = Add(x=w389, y=w388) -> (x+y=w387:sgl)
            }
          }
          n112 = And(x=w340, y=w339) -> (x .and. y?=w345:bool)
          n113 = case shown="False" w345 {
            tunnel: w344 -> [w358 w384]
            tunnel: w343 -> [w355 w383]
            tunnel: w342 -> [w357 w382]
            tunnel: w341 -> [w356 w381]
            tunnel: [w353 w377] -> w338
            tunnel: [w352 w376] -> w337
            tunnel: w340 -> [w354 _]
            tunnel: w339 -> [w359 _]
            tunnel: [w351 TRUE] -> w336
            frame False {
              n114 = Exclusive Or(1:w359, 2:w354) -> (0:w360:bool)
              n115 = case shown="True" w360 {
                tunnel: w358 -> [_ w368]
                tunnel: w357 -> [_ w365]
                tunnel: w356 -> [_ w364]
                tunnel: w355 -> [_ w366]
                tunnel: w354 -> [_ w370]
                tunnel: [w361 w369] -> w353
                tunnel: [w361 w367] -> w352
                tunnel: [FALSE TRUE] -> w351
                frame False {
                  w361 = sgl 0.0
                  # "None are valid,"
                }
                frame True {
                  # "Only 1 beacon is valid,\nUse the valid beacon"
                  n116 = case shown="False" w370 {
                    tunnel: [w372 w374] -> w369
                    tunnel: w368 -> [_ w374]
                    tunnel: [w371 w373] -> w367
                    tunnel: w366 -> [_ w373]
                    tunnel: w365 -> [w372 _]
                    tunnel: w364 -> [w371 _]
                    frame False {
                      # "Left is invalid,\nRight MUST be valid"
                    }
                    frame True {
                      # "Left is Valid"
                    }
                  }
                }
              }
            }
            frame True {
              w378 = sgl 2.0 ("y")
              # "Both are Valid"
              n117 = Add(x=w384, y=w382) -> (x+y=w379:sgl)
              n118 = Add(x=w383, y=w381) -> (x+y=w380:sgl)
              n119 = Divide(x=w380, y=w378) -> (x/y=w376:sgl)
              n120 = Divide(x=w379, y=w378) -> (x/y=w377:sgl)
            }
          }
        }
        n121 = And(x="Valid Angles - L", y="Valid Angles -R") -> (x .and. y?=w155:bool[])
        n122 = Boolean To (0,1)(Boolean=w155) -> (0, 1=w152:i16[])
        n123 = Add Array Elements(numeric array=w152) -> (sum=w153:i16)
        n124 = Greater?(x=w153, y=1) -> (0:w151:bool)
        n125 = for {
          N: w167 -> [_]
          tunnel: w151 -> [w272]
          tunnel: "Beacon Angles - L" -> [w271] mode=indexing
          tunnel: "Beacon Angles -R" -> [w270] mode=indexing
          tunnel: "Distance Between \nCameras  (*unit)" -> [w269]
          tunnel: "Distance Threshold\nRef Triangles (*unit)" -> [w268]
          tunnel: [w267] -> w138 mode=indexing
          tunnel: [w266] -> _ mode=indexing
          tunnel: [w265] -> w137 mode=indexing
          tunnel: [w264] -> _ mode=indexing
          tunnel: [w263] -> w139 mode=indexing
          tunnel: [w262] -> w145 mode=indexing
          n126 = case shown="True" w272 {
            tunnel: w271 -> [w277 w287]
            tunnel: w270 -> [w276 w286]
            tunnel: w269 -> [_ w278]
            tunnel: w268 -> [_ w279]
            tunnel: [w277 w285] -> w267
            tunnel: [w276 w284] -> w266
            tunnel: [FALSE w283] -> w265
            tunnel: [w274 w282] -> w264
            tunnel: [w274 w281] -> w263
            tunnel: [0 w280] -> w262
            frame False {
              w274 = sgl 1.0
            }
            frame True {
              # "Build Reference Triangle"
              n127 = call "Position Calc_Build Reference Triangle_R1.vi"("A2_in"=w287, "A3_in"=w286, "S1 (Length Between\n Cameras - inches)"=w278, "Distance\nThreshold"=w279) -> ("S2"=w282:sgl, "S3"=w281:sgl, "Direction"=w280:i8, "A2"=w285:sgl, "A3"=w284:sgl, "Accept"=w283:bool)  [unwired: 6 in]
            }
          }
        }
        n128 = for {
          N: w167 -> [_]
          tunnel: w137 -> [w257] mode=indexing
          tunnel: w145 -> [w261] mode=indexing
          tunnel: [w261] -> w147 mode=indexing if=w257
          shift-right: [w260] -> w141
          shift-left: 0 -> [w258]
          # "Only add to array\nif valid distance"
          n129 = Increment(x=w258) -> (x+1=w259:i32)
          n130 = Select(t=w259, s=w257, f=w258) -> (s? t:f=w260:i32)
        }
        n131 = Index Array(array=w147, index=0) -> (element=w148:i32)
        n132 = Equal?(x=w147, y=w148) -> (x = y?=w149:bool[])
        n133 = And Array Elements(Boolean array=w149) -> (logical AND=w143:bool)
        n134 = Greater?(x=w141, y=1) -> (0:w142:bool)
        n135 = And(x=w143, y=w142) -> (x .and. y?=w136:bool)
        n136 = case shown="True" w136 {
          tunnel: w167 -> [w214 w223]
          tunnel: w139 -> [_ w222]
          tunnel: w138 -> [_ w221]
          tunnel: w137 -> [_ w220]
          tunnel: [w213 w219] -> w166
          tunnel: [w212 w218] -> w162
          tunnel: [w212 w217] -> w161
          frame False {
            # "Build Array for False"
            n137 = for {
              N: w214 -> [_]
              tunnel: [sgl 0.0] -> w212 mode=indexing
              tunnel: [FALSE] -> w213 mode=indexing
            }
          }
          frame True {
            n138 = for {
              N: w223 -> [_]
              tunnel: w221 -> [w229] mode=indexing
              tunnel: w222 -> [w228] mode=indexing
              tunnel: [w227] -> w218 mode=indexing
              tunnel: [w226] -> w217 mode=indexing
              tunnel: [w225] -> w219 mode=indexing
              tunnel: w220 -> [w224] mode=indexing
              n139 = case shown="True" w224 {
                selector: w224 -> [w231 w235]
                tunnel: w229 -> [_ w243]
                tunnel: [w230 w233] -> w227
                tunnel: [w230 w234] -> w226
                tunnel: w228 -> [_ w232]
                tunnel: [w231 w235] -> w225
                frame False {
                  w230 = sgl 0.0
                  # "Current Data Set Was Not Valid\nFill with 0\nWill not be used later"
                }
                frame True {
                  # "dY"
                  # "dX"
                  # "Negate dX if A2>90"
                  # "Find LOCAL Coordinate of Each Beacon"
                  # "Current - Valid Data Set"
                  n140 = Less?(x=w243, y=sgl 90.0) -> (x < y?=w245:bool)
                  n141 = case shown="False" w245 {
                    tunnel: w243 -> [w252 w254]
                    tunnel: [w250 w255] -> w242
                    tunnel: [FALSE TRUE] -> w237
                    frame False {
                      # "Negative Y"
                      # "A2 is > 90"
                      n142 = Subtract(x=w252, y=sgl 90.0) -> (x-y=w250:sgl)
                    }
                    frame True {
                      # "Positive Y"
                      # "A2 is < 90"
                      n143 = Subtract(x=sgl 90.0, y=w254) -> (x-y=w255:sgl)
                    }
                  }
                  "dA2 4" <- w242
                  n144 = expression code="(x/180.0)*pi" "degrees to radians"(w242) -> (w240:sgl)
                  n145 = expression code="(x/180.0)*pi" "degrees to radians"(w242) -> (w241:sgl)
                  n146 = Cosine(x=w240) -> (cos(x)=w238:sgl)
                  n147 = Sine(x=w241) -> (sin(x)=w239:sgl)
                  n148 = Multiply(x=w232, y=w238) -> (x*y=w234:sgl)
                  n149 = Multiply(x=w232, y=w239) -> (x*y=w236:sgl)
                  n150 = case shown="True" w237 {
                    tunnel: w236 -> [w247 w248]
                    tunnel: [w246 w248] -> w233
                    frame False {
                      n151 = Negate(x=w247) -> (-x=w246:sgl)
                    }
                    frame True {
                    }
                  }
                }
              }
            }
          }
        }
        n152 = Subtract(x=sgl 1.0, y="Triangle Based\nWeight") -> (x-y=w158:sgl)
        "Scale Based\nWeight" <- w158
        n153 = for {
          N: w167 -> [_]
          tunnel: w166 -> [w292] mode=indexing
          tunnel: w165 -> [w291] mode=indexing
          tunnel: w164 -> [w296] mode=indexing
          tunnel: w163 -> [w295] mode=indexing
          tunnel: w162 -> [w298] mode=indexing
          tunnel: w161 -> [w297] mode=indexing
          tunnel: "Triangle Based\nWeight" -> [w294]
          tunnel: w158 -> [w293]
          tunnel: [w290] -> w135 mode=indexing
          tunnel: [w289] -> w157 mode=indexing
          tunnel: [w288] -> w156 mode=indexing
          # "If Beacon info \nis available from\nboth"
          n154 = And(x=w292, y=w291) -> (x .and. y?=w299:bool)
          n155 = case shown="True" w299 {
            selector: w299 -> [_ w325]
            tunnel: w298 -> [w306 w333]
            tunnel: w297 -> [w304 w334]
            tunnel: w296 -> [w302 w332]
            tunnel: w295 -> [w301 w331]
            tunnel: w294 -> [_ w335]
            tunnel: w293 -> [_ w330]
            tunnel: [w305 w323] -> w288
            tunnel: [w307 w324] -> w289
            tunnel: w292 -> [w308 _]
            tunnel: w291 -> [w303 _]
            tunnel: [w300 w325] -> w290
            frame False {
              n156 = case shown="False" w308 {
                selector: w308 -> [_ w320]
                tunnel: [w313 w322] -> w307
                tunnel: w306 -> [_ w322]
                tunnel: [w311 w321] -> w305
                tunnel: w304 -> [_ w321]
                tunnel: w303 -> [w314 _]
                tunnel: w302 -> [w312 _]
                tunnel: w301 -> [w310 _]
                tunnel: [w309 w320] -> w300
                frame False {
                  n157 = case shown="False" w314 {
                    selector: w314 -> [w315 w317]
                    tunnel: [w316 w319] -> w313
                    tunnel: w312 -> [_ w319]
                    tunnel: [w316 w318] -> w311
                    tunnel: w310 -> [_ w318]
                    tunnel: [w315 w317] -> w309
                    frame False {
                      w316 = sgl 0.0
                      # "None avail"
                    }
                    frame True {
                    }
                  }
                }
                frame True {
                }
              }
            }
            frame True {
              n158 = Multiply(x=w333, y=w335) -> (x*y=w329:sgl)
              n159 = Multiply(x=w334, y=w335) -> (x*y=w327:sgl)
              n160 = Multiply(x=w332, y=w330) -> (x*y=w328:sgl)
              n161 = Multiply(x=w331, y=w330) -> (x*y=w326:sgl)
              n162 = Add(x=w329, y=w328) -> (x+y=w324:sgl)
              n163 = Add(x=w327, y=w326) -> (x+y=w323:sgl)
            }
          }
        }
        "Valid Beacon Sets_" <- w135
        n164 = Boolean To (0,1)(Boolean=w135) -> (0, 1=w178:i16[])
        n165 = Add Array Elements(numeric array=w178) -> (sum=w177:i16)
        n166 = Greater?(x=w177, y=i16 1) -> (0:w175:bool)
        n167 = case shown="True" w175 {
          tunnel: w206 -> [_ w531]
          tunnel: [0.0 ("f") w530] -> w202
          tunnel: [w443 w529] -> w201
          tunnel: w197 -> [_ w447]
          tunnel: w196 -> [_ w528]
          tunnel: [FALSE w527] -> w189
          tunnel: [FALSE w526] -> w188
          tunnel: w186 -> [_ w525]
          tunnel: [sgl 0.0 w523] -> w179
          tunnel: "Distance Between \nCameras  (*unit)" -> [_ w459]
          tunnel: w157 -> [_ w458]
          tunnel: w156 -> [_ w457]
          tunnel: w135 -> [_ w456]
          tunnel: w167 -> [_ w455]
          frame False {
            w442 = 0.0 ("f")
            n168 = Bundle("f"=w442, "f"=w442) -> (w443:cluster{"f":dbl, "f":dbl})  [unwired: 1 in]
          }
          frame True {
            w495 = sgl 2.0
            w512 = 0
            # "Valid Position Ccount"
            # "Only Apply This Filtering \nif 3 or More Beacons Still Valid"
            # "Orientation Value"
            # "Orientation Valid"
            # "Y (current)"
            # "X (current)"
            # "Number of Valid\nPrevious Orientations"
            # "More than 1 Previous\nValid Positions"
            # "More than\n2previous position\navailable"
            # "Choose Beacon Set\nwith Lowest Std Dev"
            # "Y value cannot be negative"
            # "Find New # Of Valid Beacons"
            # "Adjust/Normalize\nLocal Beacon Positions\nusing Line of Best fit"
            # "# Valid\nData Sets"
            # "cam, y"
            # "cam, x"
            # "Calculate dX and dY\nfor right cam"
            # "Average dX and dY from each (valid) beacon to find position of each camera\n\nthen average all  positions for each camera find center between"
            # "Convert Slope\nto Radians"
            # "*rotate CCW in rad"
            # "Rotate Coordinate\n System by Slope"
            n169 = Boolean To (0,1)(Boolean=w447) -> (0, 1=w479:i16[])
            n170 = Initialize Array(u8 0, "Moving Average\nWindow Length") -> (w452:u8[])
            n171 = Add Array Elements(numeric array=w479) -> (sum=w473:i16)
            n172 = Greater?(x=w473, y=0) -> (0:w449:bool)
            n173 = while {
              shift-right: [w533] -> w450
              shift-left: w452 -> [w535]
              tunnel: w447 -> [w540] mode=indexing
              shift-right: [w539] -> w448
              shift-left: u8 0 -> [w541]
              tunnel: "Moving Average\nWindow Length" -> [w532]
              i -> [w534]
              stop <- w536 stop-if-true
              # "Grab Last 2 Valid Position Indexes"
              n174 = case shown="True" w540 {
                tunnel: w541 -> [w543 w545]
                tunnel: [w543 w548] -> w539
                tunnel: w535 -> [w542 w547]
                tunnel: w534 -> [_ w546]
                tunnel: [w542 w544] -> w533
                frame False {
                }
                frame True {
                  # "Update Index\nto use"
                  # "Increment\nValid Count"
                  n175 = Replace Array Subset(array=w547, new element=w546, index=w545) -> (w544:u8[])
                  n176 = Increment(x=w545) -> (x+1=w548:u8)
                }
              }
              n177 = Greater Or Equal?(x=w539, y=w532) -> (x >= y?=w538:bool)
              n178 = Greater Or Equal?(x=w534, y=w532) -> (x >= y?=w537:bool)
              n179 = Or(x=w538, y=w537) -> (x .or. y?=w536:bool)
            }
            n180 = Bundle(w458, w457) -> (→"LOCAL\nBeacon Coordinates\nRelative to Robot" →"Local Coordinates - Calculated":cluster{sgl[], sgl[]})  [unwired: 1 in]
            n181 = call "Coordinate_Outlier_Filtering_R1.vi"("Num of Beacons"=w455, "Max Std Dev(all 5)"="Max Std Dev (5)", "X in"=w458, "Valid Data\nSets in"=w456, "Y in"=w457, "Max Std Dev( 4 )"="Max Std Dev (4)", "Max Std Dev (3)"="Max Std Dev (3)") -> ("Y out"=w469:sgl[], "X out"=w470:sgl[], "Valid Beacons\nout"=w467:bool[], "Slope out"=w476:dbl)  [unwired: 3 in, 2 out]
            n182 = Inverse Tangent(1:w476) -> (0:w491:dbl)
            n183 = expression code="(x/pi)*180.0" "radians to degrees"(w491) -> (w475:dbl)
            n184 = Boolean To (0,1)(Boolean=w467) -> (0, 1=w466:i16[])
            n185 = To Single Precision Float(number=w475) -> (single precision float=w523:sgl)
            n186 = case shown="True" w449 {
              tunnel: [w558 w569] -> w526
              tunnel: w528 -> [_ w572]
              tunnel: w523 -> [w559 w566]
              tunnel: [w557 w570] -> w530
              tunnel: w525 -> [_ _]
              tunnel: w450 -> [_ w564]
              tunnel: w448 -> [_ w563]
              frame False {
                # "Since no history available,\ncheck that current is with 0-360"
                # "Use Current Orientation bc \nPrevious are not available"
                # "New Position\nValid"
                n187 = In Range and Coerce(upper limit=sgl 360.0, x=w559, lower limit=sgl -360.0 ("upper limit")) -> (In Range?=w558:bool)  [unwired: 1 out]
                n188 = Select(t=w559, s=w558, f=sgl 0.0) -> (s? t:f=w557:sgl)
              }
              frame True {
                # "Moving Average Out"
                n189 = for {
                  N: w563 -> [_]
                  shift-right: [w598] -> w574
                  shift-left: 0.0 -> [w597]
                  tunnel: w564 -> [w596] mode=indexing
                  tunnel: w572 -> [w594]
                  # "Fetch Last Valid Values\nand Sum"
                  n190 = Index Array(array=w594, index=w596) -> (element=w595:sgl)
                  n191 = Add(x=w595, y=w597) -> (x+y=w598:dbl)
                }
                n192 = Increment(x=w563) -> (x+1=w565:u8)
                n193 = Add(x=w566, y=w574) -> (x+y=w567:dbl)
                n194 = To Double Precision Float(number=w565) -> (double precision float=w573:dbl)
                n195 = Divide(x=w567, y=w573) -> (x/y=w571:dbl)
                n196 = Greater Than 0?(x=w565) -> (x > 0?=w568:bool)
                n197 = case shown="True" w568 {
                  tunnel: w571 -> [w578 w584]
                  tunnel: w564 -> [_ w591]
                  tunnel: w572 -> [_ w590]
                  tunnel: [w577 w583] -> w570
                  tunnel: [w576 w586] -> w569
                  frame False {
                    # "No Pevious is Available to Compare\ncheck that current is real angle"
                    n198 = In Range and Coerce(upper limit=sgl 360.0, x=w578, lower limit=sgl -360.0 ("upper limit")) -> (In Range?=w576:bool)  [unwired: 1 out]
                    n199 = Select(t=w578, s=w576, f=sgl 0.0) -> (s? t:f=w577:dbl)
                  }
                  frame True {
                    # "Calculate New, Weighted\nOrientation"
                    # "Check That New Value\nis within Range of Old\n(avg)"
                    # "(X1 - X2)^2"
                    # "Previous"
                    # "Pevious is Available to Compare"
                    n200 = Index Array(array=w591, index=u8 0) -> (element=w592:u8)
                    n201 = Index Array(array=w590, index=w592) -> (element=w589:sgl)
                    n202 = Subtract(x=w589, y=w584) -> (x-y=w588:dbl)
                    n203 = Absolute Value(x=w588) -> (abs(x)=w587:dbl)
                    n204 = Less Or Equal?(x=w587, y="New Orientation \nThreshold") -> (x <= y?=w586:bool)
                    n205 = Select(t=w584, s=w586, f=sgl 0.0) -> (s? t:f=w583:dbl)
                  }
                }
              }
            }
            n206 = Add Array Elements(numeric array=w466) -> (sum=w465:i16)
            n207 = Greater?(x=w465, y=i16 2) -> (0:w463:bool)
            n208 = case shown="True" w463 {
              tunnel: w455 -> [_ w556]
              tunnel: w467 -> [w549 w555]
              tunnel: w470 -> [_ w554]
              tunnel: w469 -> [_ w553]
              tunnel: [w549 w552] -> w468
              tunnel: "Distance\nBetween Beacons" -> [_ w551]
              tunnel: "Distance\nBetween Beacons \n- Tolerance" -> [_ w550]
              frame False {
                # "Don't apply filtering,\nnot enough data points"
              }
              frame True {
                # "This will filter beacons if they are calculate to be \ntoo close to each other. The beacon(s) that is\n discarded is chosen based distance between each/every\nbeacon,. Capable of filtering as long as 1/2 of sample\nset has uniform distances (between beacons)."
                # "Validate Distance Between\nEach Beacon"
                n209 = call "Beacon_Filtering_Inter_Beacon_Distance_R1.vi"("Num of Beacons"=w556, "Inter Beacon\nReal Distance"=w551, "X in"=w554, "Inter Beacon\ndelta Threshold"=w550, "Y in"=w553, "Valid Data\nSets in"=w555) -> ("Beacons Valid - Out"=w552:bool[])  [unwired: 9 in]
              }
            }
            "Post Filtering\n- Valid Beacons" <- w468
            n210 = Increment(x=w455) -> (x+1=w513:i8)
            n211 = for {
              N: w513 -> [_]
              tunnel: [w711] -> w514 mode=indexing
              tunnel: w470 -> [w707]
              tunnel: w469 -> [w710]
              tunnel: [w709] -> w515 mode=indexing
              tunnel: w459 -> [w706]
              i -> [w708]
              # "Build Array's of Coordinates\nFor All Objects"
              n212 = Greater Than 0?(x=w708) -> (x > 0?=w712:bool)
              n213 = case shown="True" w712 {
                tunnel: [w714 w720] -> w711
                tunnel: w707 -> [w717 _]
                tunnel: w710 -> [w716 _]
                tunnel: [w713 0.0] -> w709
                tunnel: w708 -> [w718 _]
                tunnel: w706 -> [_ w720]
                frame True {
                  # "Rest of Array is\nBeacon Coordinates"
                  n214 = Decrement(x=w718) -> (x-1=w715:i32)
                  n215 = Index Array(array=w717, index=w715) -> (element=w714:sgl)
                  n216 = Index Array(array=w716, index=w715) -> (element=w713:sgl)
                }
                frame False {
                  # "First object is the\nother Camera\n\nthis coordinate\nis simply:\nx = 0\ny = distance btween cams"
                }
              }
            }
            n217 = Bundle(w514, w515) -> (→"All Object Coordinates \n- Local" →"Local Coordinates - Normalized":cluster{sgl[], dbl[]})  [unwired: 1 in]
            n218 = expression code="(x/180.0)*pi" "degrees to radians"(w530) -> (w474:dbl)
            n219 = call-poly <vilib>:"2D Cartesian Coordinate Rotation.vi"("theta"=w474, "Y"=w515, "X"=w514) -> ("Y Out"=w492:dbl[], "X Out"=w493:dbl[])  [unwired: 6 in, 1 out]
            n220 = Bundle("X Out"=w493, "Y Out"=w492) -> (→"All Object Coordinates \n- Local - Rotated" →"Local Coordinates - Rotated":cluster{"X Out":dbl[], "Y Out":dbl[]})  [unwired: 1 in]
            n221 = Index Array(array=w492, index=w512) -> (element=w488:dbl)
            n222 = Index Array(array=w493, index=w512) -> (element=w511:dbl)
            n223 = for {
              N: w455 -> [_]
              tunnel: w492 -> [w702]
              tunnel: w493 -> [w703]
              tunnel: w511 -> [w701]
              tunnel: w488 -> [w700]
              tunnel: [w699] -> w485 mode=indexing
              tunnel: [w698] -> w484 mode=indexing
              tunnel: [w697] -> w460 mode=indexing
              tunnel: [w696] -> w486 mode=indexing
              i -> [w705]
              n224 = Increment(x=w705) -> (x+1=w704:i32)
              n225 = Index Array(array=w702, index=w704) -> (element=w696:dbl)
              n226 = Index Array(array=w703, index=w704) -> (element=w697:dbl)
              n227 = Subtract(x=w696, y=w700) -> (x-y=w698:dbl)
              n228 = Subtract(x=w697, y=w701) -> (x-y=w699:dbl)
            }
            n229 = Bundle(w485, w484) -> (→"dX, dY\nRight Cam":cluster{dbl[], dbl[]})  [unwired: 1 in]
            n230 = Bundle(w460, w486) -> (→"dX, dY\nLeft Cam":cluster{dbl[], dbl[]})  [unwired: 1 in]
            n231 = Unbundle("Real Beacon\n - Coordinates") -> ("X"=w509:dbl[], "Y"=w489:dbl[])
            n232 = Boolean To (0,1)(Boolean=w468) -> (0, 1=w487:i16[])
            n233 = for {
              N: w455 -> [_]
              tunnel: w468 -> [w682] mode=indexing
              tunnel: w509 -> [w679] mode=indexing
              tunnel: w489 -> [w678] mode=indexing
              tunnel: w460 -> [w681] mode=indexing
              tunnel: w486 -> [w677] mode=indexing
              tunnel: w485 -> [w680] mode=indexing
              tunnel: w484 -> [w676] mode=indexing
              tunnel: [w675] -> w508 mode=indexing
              tunnel: [w674] -> w507 mode=indexing
              tunnel: [w673] -> w506 mode=indexing
              tunnel: [w672] -> w505 mode=indexing
              n234 = case shown="True" w682 {
                tunnel: w681 -> [_ w695]
                tunnel: w680 -> [_ w694]
                tunnel: w679 -> [_ w685]
                tunnel: w678 -> [_ w684]
                tunnel: w677 -> [_ w693]
                tunnel: w676 -> [_ w686]
                tunnel: [w683 w691] -> w675
                tunnel: [w683 w690] -> w674
                tunnel: [w683 w689] -> w673
                tunnel: [w683 w688] -> w672
                frame False {
                  w683 = sgl 0.0
                  # "Add Nothing"
                }
                frame True {
                  # "realX = beaconX + dY\nrealY = beaconY + (-dx)"
                  # "Right Cam"
                  # "Left Cam"
                  # "dX = -dX\nSwap dX, dY"
                  # "Translate to Real Coordinates\nOnly Apply for Valid Beacons"
                  n235 = Negate(x=w695) -> (-x=w692:dbl)
                  n236 = Negate(x=w694) -> (-x=w687:dbl)
                  n237 = Add(x=w685, y=w693) -> (x+y=w691:dbl)
                  n238 = Add(x=w684, y=w692) -> (x+y=w690:dbl)
                  n239 = Add(x=w685, y=w686) -> (x+y=w689:dbl)
                  n240 = Add(x=w684, y=w687) -> (x+y=w688:dbl)
                }
              }
            }
            n241 = Add Array Elements(numeric array=w487) -> (sum=w490:i16)
            n242 = Add Array Elements(numeric array=w508) -> (sum=w504:dbl)
            n243 = Add Array Elements(numeric array=w507) -> (sum=w503:dbl)
            n244 = Add Array Elements(numeric array=w506) -> (sum=w502:dbl)
            n245 = Add Array Elements(numeric array=w505) -> (sum=w501:dbl)
            n246 = Divide(x=w504, y=w490) -> (x/y=w500:dbl)
            n247 = Divide(x=w503, y=w490) -> (x/y=w498:dbl)
            n248 = Divide(x=w502, y=w490) -> (x/y=w499:dbl)
            n249 = Divide(x=w501, y=w490) -> (x/y=w497:dbl)
            n250 = Bundle(w500, w498) -> (→"Left Camera Real Coordinates":cluster{dbl, dbl})  [unwired: 1 in]
            n251 = Bundle(w499, w497) -> (→"Right Camera Real Coordinate":cluster{dbl, dbl})  [unwired: 1 in]
            n252 = Add(x=w500, y=w499) -> (x+y=w496:dbl)
            n253 = Add(x=w498, y=w497) -> (x+y=w494:dbl)
            n254 = Divide(x=w496, y=w495) -> (x/y=w478:dbl)
            n255 = Divide(x=w494, y=w495) -> (x/y=w477:dbl)
            n256 = Bundle(w478, w477) -> (→"Robot Coordinates":cluster{dbl, dbl})  [unwired: 1 in]
            n257 = Less Than 0?(x=w477) -> ()  [unwired: 1 out]
            n258 = case shown="True" w449 {
              tunnel: w473 -> [_ _]
              tunnel: w478 -> [w603 w620]
              tunnel: [w604 w631] -> w527
              tunnel: w531 -> [_ w625]
              tunnel: w477 -> [w602 w619]
              tunnel: [w601 w635] -> w529
              tunnel: "Max X (arena)" -> [w600 w630]
              tunnel: "Max Y (arena)" -> [w599 w629]
              tunnel: w450 -> [_ w627]
              tunnel: w448 -> [_ w626]
              frame False {
                # "New Position\nValid"
                # "Since no history available,\ncheck that current is within\nthe bounds of the arena size"
                # "Use Current Position bc \nPrevious are not available"
                n259 = In Range and Coerce(upper limit=w600, x=w603, lower limit=sgl 0.0 ("upper limit")) -> (In Range?=w606:bool)  [unwired: 1 out]
                n260 = In Range and Coerce(upper limit=w599, x=w602, lower limit=sgl 0.0 ("upper limit")) -> (In Range?=w605:bool)  [unwired: 1 out]
                n261 = Bundle(w603, w602) -> (w601:cluster{dbl, dbl})  [unwired: 1 in]
                n262 = And(x=w606, y=w605) -> (x .and. y?=w604:bool)
              }
              frame True {
                w628 = 0.0
                # "If needed, make seperate FOR Loop for \nY only... Using more previous values than X"
                # "New Y"
                # "New X"
                # "Only consider if velocity is\ngreater than certain speed"
                # "Weighted Robot \nCoordinates"
                # "Position\nValid\n(current)"
                n263 = for {
                  N: w626 -> [_]
                  shift-right: [w644] -> w624
                  shift-left: w628 -> [w643]
                  shift-right: [w642] -> w623
                  shift-left: w628 -> [w641]
                  tunnel: w627 -> [w639] mode=indexing
                  tunnel: w625 -> [w637]
                  # "Fetch Last Valid Values\nand Sum"
                  n264 = Index Array(array=w637, index=w639) -> (element=w638:cluster{sgl, sgl})
                  n265 = Unbundle(w638) -> (w640:sgl, w636:sgl)
                  n266 = Add(x=w636, y=w641) -> (x+y=w642:dbl)
                  n267 = Add(x=w640, y=w643) -> (x+y=w644:dbl)
                }
                n268 = To Single Precision Float(number=w626) -> (single precision float=w613:sgl)
                n269 = Subtract(x=sgl 1.0, y="New Position\nWeight") -> (x-y=w622:sgl)
                n270 = Multiply(x=w622, y=w624) -> (x*y=w614:dbl)
                n271 = Multiply(x=w622, y=w623) -> (x*y=w615:dbl)
                n272 = Divide(x=w614, y=w613) -> (x/y=w611:dbl)
                n273 = Divide(x=w615, y=w613) -> (x/y=w612:dbl)
                n274 = Multiply(x="New Position\nWeight", y=w620) -> (x*y=w617:dbl)
                n275 = Multiply(x="New Position\nWeight", y=w619) -> (x*y=w616:dbl)
                n276 = Add(x=w617, y=w611) -> (x+y=w610:dbl)
                n277 = Add(x=w616, y=w612) -> (x+y=w609:dbl)
                n278 = Greater Than 0?(x=w626) -> (x > 0?=w634:bool)
                n279 = case shown="True" w634 {
                  tunnel: w610 -> [w649 w656]
                  tunnel: w609 -> [w648 w655]
                  tunnel: w627 -> [_ w668]
                  tunnel: w625 -> [_ w667]
                  tunnel: [w646 w656] -> w633
                  tunnel: [w645 w655] -> w632
                  tunnel: [w650 w657] -> w631
                  tunnel: w630 -> [w652 _]
                  tunnel: w629 -> [w651 _]
                  frame False {
                    w647 = sgl 0.0 ("upper limit")
                    # "Check that within bounds of arena"
                    # "No Pevious is Available to Compare"
                    n280 = In Range and Coerce(upper limit=w652, x=w649, lower limit=w647) -> (In Range?=w654:bool)  [unwired: 1 out]
                    n281 = In Range and Coerce(upper limit=w651, x=w648, lower limit=w647) -> (In Range?=w653:bool)  [unwired: 1 out]
                    n282 = And(x=w654, y=w653) -> (x .and. y?=w650:bool)
                    n283 = Select(t=w649, s=w650, f=w647) -> (s? t:f=w646:dbl)
                    n284 = Select(t=w648, s=w650, f=w647) -> (s? t:f=w645:dbl)
                  }
                  frame True {
                    # "New"
                    # "(Y1 - Y2)^2"
                    # "(X1 - X2)^2"
                    # "Previous"
                    # "Pevious is Available to Compare"
                    n285 = Index Array(array=w668, index=u8 0) -> (element=w670:u8)
                    n286 = Index Array(array=w667, index=w670) -> (element=w669:cluster{sgl, sgl})
                    n287 = Unbundle(w669) -> (w659:sgl, w658:sgl)
                    n288 = Subtract(x=w659, y=w656) -> (x-y=w664:dbl)
                    n289 = Subtract(x=w655, y=w658) -> (x-y=w663:dbl)
                    n290 = Square(x=w664) -> (x^2=w662:dbl)
                    n291 = Square(x=w663) -> (x^2=w661:dbl)
                    n292 = Add(x=w662, y=w661) -> (x+y=w665:dbl)
                    n293 = Square Root(x=w665) -> (sqrt(x)=w660:dbl)
                    n294 = Less Or Equal?(x=w660, y="New Position \nThreshold") -> (x <= y?=w657:bool)
                  }
                }
                n295 = Bundle("upper limit"=w633, "upper limit"=w632) -> (w635:cluster{"upper limit":dbl, "upper limit":dbl})  [unwired: 1 in]
              }
            }
          }
        }
        "Orietnation\n(current)" <- w179
        n296 = And(x=w189, y=w188) -> (x .and. y?=w130:bool)
        "Position Valid" <- w130
        n297 = Exclusive Or(1:w188, 2:w189) -> (0:w187:bool)
        n298 = case shown="True" w130 {
          tunnel: [w727 w730] -> w131
          tunnel: [w728 w729] -> w134
          tunnel: w202 -> [_ w730]
          tunnel: w201 -> [_ w729]
          tunnel: w187 -> [_ _]
          frame False {
            w727 = sgl 0.0 ("f")
            n299 = Bundle("f"=w727, "f"=w727) -> (w728:cluster{"f":sgl, "f":sgl})  [unwired: 1 in]
          }
          frame True {
            # "For Servos"
            "Last Orientation" <- w730
            "Last Position" <- w729
          }
        }
        "Robot Coordinates - Avgd" <- w134
        "Orientation Avgd" <- w131
        n300 = local read "History Size"() -> (w181:u8)
        n301 = Decrement(x=w181) -> (x-1=w182:u8)
        n302 = for {
          N: w181 -> [_]
          shift-right: [w768] -> w204
          shift-left: w200 -> [w767]
          tunnel: w134 -> [w766]
          tunnel: w182 -> [w765]
          i -> [w764]
          n303 = Subtract(x=w765, y=w764) -> (x-y=w763:i32)
          n304 = Equal To 0?(x=w763) -> (x = 0?=w762:bool)
          n305 = case shown="False" w762 {
            tunnel: w763 -> [w770 w775]
            tunnel: w767 -> [w773 w776]
            tunnel: [w771 w777] -> w768
            tunnel: w766 -> [_ w774]
            frame False {
              n306 = Decrement(x=w770) -> (x-1=w769:i32)
              n307 = Index Array(array=w773, index=w769) -> (element=w772:cluster{sgl, sgl})
              n308 = Replace Array Subset(array=w773, new element=w772, index=w770) -> (w771:cluster{sgl, sgl}[])
            }
            frame True {
              n309 = Replace Array Subset(array=w776, new element=w774, index=w775) -> (w777:cluster{sgl, sgl}[])
            }
          }
        }
        n310 = Unbundle(w134) -> ("upper limit"=w133:dbl, "upper limit"=w132:dbl)
        n311 = shared-variable "RT myRIO Target - Overlord\\Localization_Variables_r0.lvlib\\loc_x"(w133) -> ()  [unwired: 1 in, 1 out]
        n312 = shared-variable "RT myRIO Target - Overlord\\Localization_Variables_r0.lvlib\\loc_y"(w132) -> ()  [unwired: 1 in, 1 out]
        n313 = shared-variable "RT myRIO Target - Overlord\\Localization_Variables_r0.lvlib\\loc_theta"(w131) -> ()  [unwired: 1 in, 1 out]
        n314 = shared-variable "RT myRIO Target - Overlord\\Localization_Variables_r0.lvlib\\loc_flag"(w130) -> ()  [unwired: 1 in, 1 out]
        n315 = Decrement(x=w181) -> (x-1=w183:u8)
        n316 = for {
          N: w181 -> [_]
          shift-right: [w752] -> w205
          shift-left: w199 -> [w751]
          tunnel: w131 -> [w750]
          tunnel: w183 -> [w749]
          i -> [w748]
          n317 = Subtract(x=w749, y=w748) -> (x-y=w746:i32)
          n318 = Equal To 0?(x=w746) -> (x = 0?=w747:bool)
          n319 = case shown="False" w747 {
            tunnel: w746 -> [w754 w759]
            tunnel: w751 -> [w757 w760]
            tunnel: [w755 w761] -> w752
            tunnel: w750 -> [_ w758]
            frame False {
              # "Shift"
              n320 = Decrement(x=w754) -> (x-1=w753:i32)
              n321 = Index Array(array=w757, index=w753) -> (element=w756:sgl)
              n322 = Replace Array Subset(array=w757, new element=w756, index=w754) -> (w755:sgl[])
            }
            frame True {
              # "insert new"
              n323 = Replace Array Subset(array=w760, new element=w758, index=w759) -> (w761:sgl[])
            }
          }
        }
        n324 = Decrement(x=w181) -> (x-1=w180:u8)
        n325 = for {
          N: w181 -> [_]
          shift-right: [w737] -> w203
          shift-left: w198 -> [w736]
          tunnel: w130 -> [w735]
          tunnel: w180 -> [w734]
          i -> [w733]
          n326 = Subtract(x=w734, y=w733) -> (x-y=w731:i32)
          n327 = Equal To 0?(x=w731) -> (x = 0?=w732:bool)
          n328 = case shown="False" w732 {
            tunnel: w736 -> [w742 w744]
            tunnel: [w740 w745] -> w737
            tunnel: w735 -> [_ w743]
            tunnel: w731 -> [w738 _]
            frame False {
              n329 = Decrement(x=w738) -> (x-1=w739:i32)
              n330 = Index Array(array=w742, index=w739) -> (element=w741:bool)
              n331 = Replace Array Subset(array=w742, new element=w741, index=w738) -> (w740:bool[])
            }
            frame True {
              n332 = Replace Array Subset(array=w744, new element=w743) -> (w745:bool[])  [unwired: 1 in]
            }
          }
        }
        n333 = Boolean To (0,1)(Boolean=w203) -> (0, 1=w195:i16[])
        n334 = Add Array Elements(numeric array=w195) -> (sum=w193:i16)
        n335 = Greater Or Equal?(x=w193, y=i16 2) -> (x >= y?=→"Position \nLock Status":bool)
        n336 = case shown="True" w130 {
          tunnel: w134 -> [_ w726]
          frame False {
          }
          frame True {
            # "update debug graph\nif current is valid"
            n337 = Unbundle(w726) -> ("upper limit"=w725:dbl, "upper limit"=w724:dbl)
            n338 = Build Array(w724) -> (w722:dbl[])
            n339 = Build Array(w725) -> (w723:dbl[])
            n340 = Bundle(w723, w722) -> (→"Real Position in Course 2":cluster{dbl[], dbl[]})  [unwired: 1 in]
          }
        }
      }
    }
    n341 = case shown="True" w113 {
      tunnel: w112 -> [_ w120]
      frame False {
      }
      frame True {
        n342 = call "Tick Count3"() -> ("Tick Count(uSec)"=w121:u32)
        n343 = Subtract(x=w121, y=w120) -> (x-y=w124:u32)
        n344 = Divide(x=w124, y=u32 1000 ("x")) -> (x/y=→"dT":dbl)
      }
    }
    n345 = call "Tick Count6"() -> ("Tick Count(uSec)"=w110:u32)
    "Robot Coordinates\nHistory" <- w109
    "Orientation\nHistory" <- w114
    "Position Valid\nHistory" <- w115
  }
  n346 = disable-structure shown="Enabled" {
    disable-tunnel: [w780 _] -> _
    disable-tunnel: ["Search Step Size\n(deg)" _] -> _
    frame Enabled {
      n347 = Multiply(x=3.413333333333333, y="Search Step Size\n(deg)") -> (x*y=w778:dbl)
      n348 = To Unsigned Word Integer(number=w778) -> (unsigned 16bit integer=w780:u16)
    }
    frame Disabled {
    }
  }
  n349 = Multiply(x="Move Servo\nThreshold (deg)", y=3.413333333333333) -> (x*y=w18:dbl)
  n350 = To Unsigned Word Integer(number=w18) -> ()  [unwired: 1 out]
  n351 = call "Tick Count8"() -> ()  [unwired: 1 out]
  n352 = flat-sequence {
    tunnel: [w784] -> w42
    tunnel: [w783] -> w41
    tunnel: [w788] -> w40
    tunnel: ["Left Servo\nID"] -> w29
    tunnel: ["Right Servo\nID"] -> w28
    tunnel: ["Compliance Slope"] -> w27
    tunnel: [w828] -> w39
    tunnel: [w827] -> w38
    tunnel: w42 -> [w826]
    tunnel: w41 -> [w825]
    tunnel: w40 -> [w824]
    tunnel: w29 -> [w822]
    tunnel: w28 -> [w821]
    tunnel: w27 -> [w820]
    tunnel: w39 -> [w1101]
    tunnel: w38 -> [w1100]
    frame #0 {
      # "BAUD RATE"
      # "Initialize UART and DIO"
      n353 = call-poly "VISA Configure Serial Port"("VISA resource name"=refnum<visa-resource-name> "ASRL1::INSTR", "Enable Termination\nChar (T)"=FALSE ("Enable Termination\nChar (T)"), "baud rate (9600)"=u32 115200) -> ("VISA resource name out"=w784:refnum<visa-resource-name>)  [unwired: 11 in, 1 out]
      n354 = call <vilib>:"Smart Open.vi"("Channel Names"=tag[] ["A/DIO2"]) -> ("DIO Ref Out"=w783:T7)  [unwired: 9 in, 1 out]
      n355 = flat-sequence {
        tunnel: w784 -> [w796]
        tunnel: w783 -> [w795]
        tunnel: "Left Servo\nID" -> [w797]
        tunnel: [w794] -> w785
        tunnel: "Compliance Slope" -> [w793]
        tunnel: "Right Servo\nID" -> [w810]
        tunnel: w785 -> [w809]
        tunnel: "Compliance Slope" -> [w808]
        tunnel: w784 -> [w807]
        tunnel: w783 -> [w806]
        frame #0 {
          w794 = 3
          n356 = while {
            tunnel: w794 -> [w803]
            tunnel: w796 -> [w801]
            tunnel: w795 -> [w800]
            tunnel: w797 -> [w799]
            tunnel: w793 -> [w798]
            i -> [w804]
            stop <- w802 stop-if-true
            n357 = call "Set_Compliance_Slope_R2.vi"("Compliance Slope"=w798, "DIO Ref Out"=w800, "VISA resource name"=w801, "Servo ID"=w799) -> ()  [unwired: 6 in, 2 out]
            n358 = Increment(x=w804) -> (x+1=w805:i32)
            n359 = Greater Or Equal?(x=w805, y=w803) -> (x >= y?=w802:bool)
          }
        }
        frame #1 {
          n360 = while {
            tunnel: w809 -> [w816]
            tunnel: w810 -> [w814]
            tunnel: w807 -> [w813]
            tunnel: w806 -> [w812]
            tunnel: w808 -> [w811]
            i -> [w817]
            stop <- w815 stop-if-true
            n361 = call "Set_Compliance_Slope_R2.vi"("Compliance Slope"=w811, "DIO Ref Out"=w812, "VISA resource name"=w813, "Servo ID"=w814) -> ()  [unwired: 6 in, 2 out]
            n362 = Increment(x=w817) -> (x+1=w818:i32)
            n363 = Greater Or Equal?(x=w818, y=w816) -> (x >= y?=w815:bool)
          }
        }
      }
      n364 = call "Tick Count"() -> ("Tick Count(uSec)"=w788:u32)
    }
    frame #1 {
      # "Service Count"
      n365 = while {
        shift-right: [w831] -> _
        shift-left: w824 -> [w848]
        tunnel: "Max Write\nTx Attempts" -> [w843]
        tunnel: "Max Read\nTx Attempts" -> [w842]
        shift-right: [w838] -> w828
        shift-left: w826 -> [w841]
        shift-right: [w837] -> w827
        shift-left: w825 -> [w840]
        tunnel: w822 -> [w836]
        tunnel: w821 -> [w835]
        tunnel: w820 -> [w834]
        shift-right: [w832] -> _
        shift-left: u16 0 -> [w833]
        stop <- "close comms" stop-if-true
        # "Loop Timer"
        n366 = local read "SERVO ENABLE"() -> (w830:bool)
        n367 = call "Tick Count2"() -> ("Tick Count(uSec)"=w831:u32)
        n368 = Subtract(x=w831, y=w848) -> (x-y=w847:u32)
        n369 = call "Wait4"("Count(mSec)"="Servo Comm\nLoop Time (ms)") -> ()  [unwired: 1 out]
        n370 = Divide(x=w847, y=u32 1000) -> (x/y=→"dT - Comm Loop":dbl)
        n371 = case shown="True" w830 {
          tunnel: w843 -> [_ w857]
          tunnel: w842 -> [_ w888]
          tunnel: w841 -> [w851 w852]
          tunnel: w840 -> [w850 w881]
          tunnel: [w851 w854] -> w838
          tunnel: [w850 w853] -> w837
          tunnel: w836 -> [_ w860]
          tunnel: w835 -> [_ w859]
          tunnel: w834 -> [_ w858]
          tunnel: w833 -> [_ w856]
          tunnel: [u16 100 w855] -> w832
          frame False {
            # "Restart at same value\nUsed to Periodically update \nCompliance Slope"
          }
          frame True {
            n372 = flat-sequence {
              tunnel: [w894] -> w892
              tunnel: [w895] -> w891
              tunnel: [w893] -> w890
              tunnel: w888 -> [w896]
              tunnel: [w898] -> w879
              tunnel: [w897] -> w877
              tunnel: w852 -> [w898]
              tunnel: w881 -> [w897]
              tunnel: w860 -> [w893]
              tunnel: w892 -> [w916]
              tunnel: w891 -> [w917]
              tunnel: w890 -> [w915]
              tunnel: [w915] -> w889
              tunnel: [w914] -> w882
              tunnel: [w913] -> w880
              tunnel: w879 -> [w913]
              tunnel: [w912] -> w878
              tunnel: w877 -> [w912]
              tunnel: w889 -> [w938]
              tunnel: w857 -> [w937]
              tunnel: w882 -> [w932]
              tunnel: w880 -> [w934]
              tunnel: w878 -> [w933]
              tunnel: [w934] -> w875
              tunnel: [w933] -> w873
              tunnel: [w971] -> w876
              tunnel: w875 -> [w971]
              tunnel: [w970] -> w874
              tunnel: w873 -> [w970]
              tunnel: ["Servo Comm\nWait Time - (ms)"] -> w865
              tunnel: w888 -> [w978]
              tunnel: [w977] -> w887
              tunnel: [w976] -> w886
              tunnel: [w972] -> w884
              tunnel: w876 -> [w975]
              tunnel: w874 -> [w974]
              tunnel: [w975] -> w872
              tunnel: [w974] -> w869
              tunnel: [w973] -> w866
              tunnel: w865 -> [w973]
              tunnel: w859 -> [w972]
              tunnel: w887 -> [w998]
              tunnel: w886 -> [w997]
              tunnel: [w996] -> w885
              tunnel: w884 -> [w996]
              tunnel: [w995] -> w883
              tunnel: w872 -> [w994]
              tunnel: [w994] -> w871
              tunnel: [w993] -> w870
              tunnel: w869 -> [w993]
              tunnel: w866 -> [w992]
              tunnel: [w992] -> w864
              tunnel: w885 -> [w1020]
              tunnel: w883 -> [w1018]
              tunnel: w857 -> [w1019]
              tunnel: w871 -> [w1017]
              tunnel: w870 -> [w1016]
              tunnel: [w1017] -> w868
              tunnel: [w1016] -> w867
              tunnel: w864 -> [w1013]
              tunnel: [w1013] -> w863
              tunnel: w868 -> [w1053]
              tunnel: w867 -> [w1052]
              tunnel: w863 -> [w1051]
              tunnel: [w1053] -> w862
              tunnel: [w1052] -> w861
              tunnel: w862 -> [w1057]
              tunnel: w861 -> [w1056]
              tunnel: w860 -> [w1062]
              tunnel: w859 -> [w1061]
              tunnel: w858 -> [w1060]
              tunnel: w856 -> [w1055]
              tunnel: w857 -> [w1059]
              tunnel: [w1058] -> w855
              tunnel: [w1057] -> w854
              tunnel: [w1056] -> w853
              frame #0 {
                n373 = while {
                  tunnel: [w911] -> w894
                  tunnel: w893 -> [w910]
                  tunnel: [w903] -> w895
                  tunnel: w896 -> [w901]
                  tunnel: w898 -> [w900]
                  tunnel: w897 -> [w899]
                  i -> [w902]
                  stop <- w904 stop-if-true
                  # "Attemp to Read Until\nMax Read Tx Attemps Limit"
                  n374 = call "ReadServo_R3.vi"("DIO Ref In"=w899, "VISA resource name out"=w900, "Servo ID"=w910) -> ("Error"=w907:u8, "Valid Checksum"=w908:bool, "Current Position"=w911:u64)  [unwired: 6 in]
                  n375 = Increment(x=w902) -> (x+1=w905:i32)
                  n376 = Equal To 0?(x=w907) -> (x = 0?=w909:bool)
                  n377 = Greater Or Equal?(x=w905, y=w901) -> (x >= y?=w906:bool)
                  n378 = And(x=w908, y=w909) -> (x .and. y?=w903:bool)
                  n379 = Or(x=w903, y=w906) -> (x .or. y?=w904:bool)
                }
              }
              frame #1 {
                # "Read Position First"
                n380 = local read "Servo Goal Position\n - Left"() -> (w914:u16)
                n381 = case shown="True" w917 {
                  tunnel: w916 -> [_ w922]
                  tunnel: w914 -> [_ w920]
                  frame False {
                  }
                  frame True {
                    # "Convert Received Position to Angle Relative to Robot"
                    # "45 DEG MOUNT OFFSET"
                    # "1024/300"
                    n382 = local write "Current L (10bit)"(w922) -> ()
                    n383 = To Word Integer(number=w922) -> (16bit integer=w926:i16)
                    n384 = To Word Integer(number=w920) -> (16bit integer=w925:i16)
                    n385 = Subtract(x=w925, y=w926) -> (x-y=w924:i16)
                    n386 = Divide(x=w922, y=3.413333333333333) -> (x/y=w930:dbl)
                    n387 = Absolute Value(x=w924) -> (abs(x)=w923:i16)
                    n388 = Subtract(x=w930, y=sgl 60.0) -> (x-y=w928:dbl)
                    n389 = Greater?(x=w923, y=u16 5) -> (0:w919:bool)
                    n390 = Add(x=w928, y=sgl 45.0) -> (x+y=w918:dbl)
                    n391 = local write "Move Servo - L"(w919) -> ()
                    n392 = local write "Servo Moving - L"(w919) -> ()
                    n393 = local write "Current Angle\n - Left (internal)"(w918) -> ()
                    n394 = shared-variable "RT myRIO Target - Overlord\\Localization_Variables_r0.lvlib\\Left Servo Angle_Current"(w918) -> ()  [unwired: 1 in, 1 out]
                  }
                }
              }
              frame #2 {
                n395 = local read "Move Servo - L"() -> (w935:bool)
                n396 = case shown="True" w935 {
                  tunnel: w938 -> [_ w953]
                  tunnel: w932 -> [_ w940]
                  tunnel: [TRUE w951] -> w936
                  tunnel: w937 -> [_ w943]
                  tunnel: w934 -> [_ w942]
                  tunnel: w933 -> [_ w941]
                  frame False {
                    # "Only Send if Current Position is far enough"
                  }
                  frame True {
                    w949 = 1
                    # "High Byte"
                    # "Low Byte"
                    n397 = Type Cast(type="", x=w940) -> (*(type *) &x=w950:string)
                    n398 = local write "Servo Moving - L"(TRUE) -> ()
                    n399 = String Subset(string=w950, offset (0)=1, length (rest)=w949) -> (substring=w945:string)
                    n400 = String Subset(string=w950, offset (0)=0, length (rest)=w949) -> (substring=w944:string)
                    n401 = while {
                      tunnel: w953 -> [w967]
                      tunnel: [w959] -> w951
                      tunnel: w945 -> [w963]
                      tunnel: w944 -> [w962]
                      tunnel: w943 -> [w956]
                      tunnel: w942 -> [w955]
                      tunnel: w941 -> [w954]
                      i -> [w957]
                      stop <- w958 stop-if-true
                      # "Attemp to Write Until\nMax Write Tx Attemps Limit"
                      n402 = call "MoveServo_R3.vi"("DIO Ref Out"=w954, "VISA resource name out"=w955, "GP - Low Byte"=w963, "GP - High Byte"=w962, "Servo ID"=w967) -> ("Valid Checksum"=w964:bool, "Error"=w966:u64)  [unwired: 5 in]
                      n403 = Equal To 0?(x=w966) -> (x = 0?=w965:bool)
                      n404 = And(x=w964, y=w965) -> (x .and. y?=w959:bool)
                      n405 = Increment(x=w957) -> (x+1=w961:i32)
                      n406 = Greater Or Equal?(x=w961, y=w956) -> (x >= y?=w960:bool)
                      n407 = Or(x=w959, y=w960) -> (x .or. y?=w958:bool)
                    }
                  }
                }
                n408 = case shown="True" w936 {
                  frame False {
                  }
                  frame True {
                    # "Update Servo flag"
                    n409 = local write "Move Servo - L"(FALSE) -> ()
                  }
                }
              }
              frame #3 {
                n410 = call "Wait2"("Count(mSec)"="Servo Comm\nWait Time - (ms)") -> ()  [unwired: 1 out]
              }
              frame #4 {
                n411 = while {
                  tunnel: [w991] -> w977
                  tunnel: w972 -> [w990]
                  tunnel: [w983] -> w976
                  tunnel: w978 -> [w981]
                  tunnel: w975 -> [w980]
                  tunnel: w974 -> [w979]
                  i -> [w982]
                  stop <- w984 stop-if-true
                  # "Attemp to Read Until\nMax Read Tx Attemps Limit"
                  n412 = call "ReadServo_R3.vi"("DIO Ref In"=w979, "VISA resource name out"=w980, "Servo ID"=w990) -> ("Error"=w987:u8, "Valid Checksum"=w988:bool, "Current Position"=w991:u64)  [unwired: 6 in]
                  n413 = Increment(x=w982) -> (x+1=w985:i32)
                  n414 = Equal To 0?(x=w987) -> (x = 0?=w989:bool)
                  n415 = Greater Or Equal?(x=w985, y=w981) -> (x >= y?=w986:bool)
                  n416 = And(x=w988, y=w989) -> (x .and. y?=w983:bool)
                  n417 = Or(x=w983, y=w986) -> (x .or. y?=w984:bool)
                }
              }
              frame #5 {
                n418 = local read "Servo Goal Position\n - Right"() -> (w995:u16)
                n419 = case shown="True" w997 {
                  tunnel: w998 -> [_ w1002]
                  tunnel: w995 -> [_ w1001]
                  frame False {
                    # "Don't update current position"
                  }
                  frame True {
                    # "Convert Received Position to Angle Relative to Robot"
                    # "45 DEG MOUNT OFFSET"
                    # "1024/300"
                    n420 = local write "Current R (10bit)"(w1002) -> ()
                    n421 = Divide(x=w1002, y=3.413333333333333) -> (x/y=w1011:dbl)
                    n422 = Subtract(x=w1011, y=sgl 60.0) -> (x-y=w1009:dbl)
                    n423 = Subtract(x=w1009, y=sgl 45.0) -> (x-y=w999:dbl)
                    n424 = To Word Integer(number=w1001) -> (16bit integer=w1006:i16)
                    n425 = To Word Integer(number=w1002) -> (16bit integer=w1007:i16)
                    n426 = shared-variable "RT myRIO Target - Overlord\\Localization_Variables_r0.lvlib\\Right Servo Angle_Current"(w999) -> ()  [unwired: 1 in, 1 out]
                    n427 = local write "Current Angle\n - Right (internal)"(w999) -> ()
                    n428 = Subtract(x=w1006, y=w1007) -> (x-y=w1005:i16)
                    n429 = Absolute Value(x=w1005) -> (abs(x)=w1004:i16)
                    n430 = Greater?(x=w1004, y=u16 5) -> (0:w1000:bool)
                    n431 = local write "Move Servo - R"(w1000) -> ()
                    n432 = local write "Servo Moving - R"(w1000) -> ()
                  }
                }
              }
              frame #6 {
                n433 = local read "Move Servo - R"() -> (w1014:bool)
                n434 = case shown="True" w1014 {
                  tunnel: w1018 -> [_ w1023]
                  tunnel: w1020 -> [_ w1030]
                  tunnel: [TRUE w1031] -> w1015
                  tunnel: w1019 -> [_ w1026]
                  tunnel: w1017 -> [_ w1025]
                  tunnel: w1016 -> [_ w1024]
                  frame False {
                  }
                  frame True {
                    w1033 = 1
                    # "High Byte"
                    # "Low Byte"
                    n435 = Type Cast(type="", x=w1023) -> (*(type *) &x=w1032:string)
                    n436 = local write "Servo Moving - R"(TRUE) -> ()
                    n437 = String Subset(string=w1032, offset (0)=1, length (rest)=w1033) -> (substring=w1029:string)
                    n438 = String Subset(string=w1032, offset (0)=0, length (rest)=w1033) -> (substring=w1028:string)
                    n439 = while {
                      tunnel: [w1042] -> w1031
                      tunnel: w1030 -> [w1047]
                      tunnel: w1029 -> [w1046]
                      tunnel: w1028 -> [w1045]
                      tunnel: w1026 -> [w1040]
                      tunnel: w1025 -> [w1038]
                      tunnel: w1024 -> [w1037]
                      i -> [w1041]
                      stop <- w1039 stop-if-true
                      # "Attemp to Write Until\nMax Write Tx Attemps Limit"
                      n440 = call "MoveServo_R3.vi"("DIO Ref Out"=w1037, "VISA resource name out"=w1038, "GP - Low Byte"=w1046, "GP - High Byte"=w1045, "Servo ID"=w1047) -> ("Valid Checksum"=w1049:bool, "Error"=w1048:u64)  [unwired: 5 in]
                      n441 = Increment(x=w1041) -> (x+1=w1043:i32)
                      n442 = Greater Or Equal?(x=w1043, y=w1040) -> (x >= y?=w1044:bool)
                      n443 = Equal To 0?(x=w1048) -> (x = 0?=w1050:bool)
                      n444 = And(x=w1049, y=w1050) -> (x .and. y?=w1042:bool)
                      n445 = Or(x=w1042, y=w1044) -> (x .or. y?=w1039:bool)
                    }
                  }
                }
                n446 = case shown="True" w1015 {
                  frame False {
                  }
                  frame True {
                    # "Update Servo flag"
                    n447 = local write "Move Servo - R"(FALSE) -> ()
                  }
                }
              }
              frame #7 {
                n448 = call "Wait3"("Count(mSec)"=w1051) -> ()  [unwired: 1 out]
              }
              frame #8 {
                # "Increment Service Count"
                # "Update Compliance Slope\nEvery x loops"
                n449 = Equal?(x=w1055, y=u16 1000) -> (x = y?=w1064:bool)
                n450 = case shown="True" w1064 {
                  tunnel: w1060 -> [_ w1074]
                  tunnel: w1057 -> [_ w1073]
                  tunnel: w1056 -> [_ w1072]
                  tunnel: w1057 -> [_ w1071]
                  tunnel: w1056 -> [_ w1070]
                  tunnel: w1062 -> [_ w1069]
                  tunnel: w1061 -> [_ w1068]
                  tunnel: w1055 -> [w1065 _]
                  tunnel: [w1065 u16 0] -> w1063
                  tunnel: w1059 -> [_ w1066]
                  frame False {
                  }
                  frame True {
                    # "Reset Service\nCount"
                    n451 = flat-sequence {
                      tunnel: w1073 -> [w1079]
                      tunnel: w1072 -> [w1078]
                      tunnel: w1069 -> [w1080]
                      tunnel: [w1076] -> w1075
                      tunnel: w1074 -> [w1077]
                      tunnel: w1066 -> [w1076]
                      tunnel: w1068 -> [w1092]
                      tunnel: w1075 -> [w1091]
                      tunnel: w1074 -> [w1090]
                      tunnel: w1071 -> [w1089]
                      tunnel: w1070 -> [w1088]
                      frame #0 {
                        n452 = while {
                          tunnel: w1076 -> [w1087]
                          tunnel: w1079 -> [w1085]
                          tunnel: w1078 -> [w1084]
                          tunnel: w1080 -> [w1083]
                          tunnel: w1077 -> [w1082]
                          i -> [w1081]
                          stop <- w1086 stop-if-true
                          n453 = call "Set_Compliance_Slope_R2.vi"("Compliance Slope"=w1082, "DIO Ref Out"=w1084, "VISA resource name"=w1085, "Servo ID"=w1083) -> ()  [unwired: 6 in, 2 out]
                          n454 = Greater Or Equal?(x=w1081, y=w1087) -> (x >= y?=w1086:bool)
                        }
                      }
                      frame #1 {
                        n455 = while {
                          tunnel: w1091 -> [w1099]
                          tunnel: w1092 -> [w1097]
                          tunnel: w1089 -> [w1096]
                          tunnel: w1088 -> [w1095]
                          tunnel: w1090 -> [w1094]
                          i -> [w1093]
                          stop <- w1098 stop-if-true
                          n456 = call "Set_Compliance_Slope_R2.vi"("Compliance Slope"=w1094, "DIO Ref Out"=w1095, "VISA resource name"=w1096, "Servo ID"=w1097) -> ()  [unwired: 6 in, 2 out]
                          n457 = Greater Or Equal?(x=w1093, y=w1099) -> (x >= y?=w1098:bool)
                        }
                      }
                    }
                  }
                }
                n458 = Increment(x=w1063) -> (x+1=w1058:u16)
              }
            }
          }
        }
      }
    }
    frame #2 {
      n459 = VISA Close(VISA resource name=w1101) -> ()  [unwired: 1 in, 1 out]
      n460 = call <vilib>:"Close.vi"("DIO Ref In"=w1100) -> ()  [unwired: 10 in, 1 out]
    }
  }
  n461 = while {
    stop <- FALSE stop-if-true
    n462 = call "Wait9"("Count(mSec)"=u32 1000) -> ()  [unwired: 1 out]
  }
  n463 = while {
    shift-right: [w1162] -> _
    shift-left: "Initial Main State - Left" -> [w1187]
    shift-right: [w1154] -> _
    shift-left: "Search Direction - in - L" -> [w1181]
    shift-right: [w1153] -> _
    shift-left: FALSE -> [w1180]
    shift-right: [w1156] -> _
    shift-left: w13 -> [w1155]
    shift-right: [w1157] -> _
    shift-left: w13 -> [w1174]
    shift-right: [w1158] -> _
    shift-left: w13 -> [w1179]
    shift-right: [w1159] -> _
    shift-left: w13 -> [w1173]
    shift-right: [w1160] -> _
    shift-left: w13 -> [w1172]
    shift-right: [w1105] -> _
    shift-left: "Search Direction - in - Right" -> [w1129]
    shift-right: [w1150] -> _
    shift-left: FALSE -> [w1127]
    shift-right: [w1151] -> _
    shift-left: w12 -> [w1118]
    shift-right: [w1106] -> _
    shift-left: w12 -> [w1117]
    shift-right: [w1107] -> _
    shift-left: w12 -> [w1124]
    shift-right: [w1108] -> _
    shift-left: w12 -> [w1126]
    shift-right: [w1109] -> _
    shift-left: w12 -> [w1125]
    shift-right: [w1116] -> _
    shift-left: "Initial Main State- Right" -> [w1141]
    shift-right: [w1146] -> _
    shift-left: 0 -> [w1148]
    shift-right: [w1113] -> _
    shift-left: 0 -> [w1133]
    shift-right: [w1145] -> _
    shift-left: "Initial Tracking State - Left" -> [w1147]
    shift-right: [w1111] -> _
    shift-left: "Initial Tracking State - Right" -> [w1139]
    shift-right: [w1112] -> _
    shift-left: "Initial Recovery State  - Right" -> [w1140]
    shift-right: [w1143] -> _
    shift-left: "Initial Recovery State - L" -> [w1144]
    stop <- FALSE stop-if-true
    w1166 = T2."Tracking" ("Next Main State")
    # "Wait for New"
    # "ADD TRACKING TIMEOUT COUNT**********************"
    # "Service Track Angle Flag"
    # "Add Logic to Have Search Directions\nopposite if Both Searching"
    # "REMOVE LAST GOAL POSITION WITH cURRENT"
    # "Go to Current State"
    # "Add Logic to Have Search Directions\nopposite if Both Searching"
    # "Manuallly Reset\nRespond Var"
    # "Manuallly Reset\nRespond Var"
    # "Update Comm Process Variables"
    # "Both Tracking"
    # "Current delta - L"
    # "delta move sum - R"
    # "delta move sum - L"
    # "Current delta - R"
    # "Service Move Respond Variables"
    n464 = local read "Min Num Frames\nper Search"() -> (w1152:i32)
    n465 = local read "Minimum Delta \nServo Threshold"() -> (w1171:i16)
    n466 = local read "Maximum Move \nServo Threshold"() -> (w1170:i16)
    n467 = local read "Middle Beacon\nCoordinates"() -> (w1119:cluster{"X":sgl, "Y":sgl})
    n468 = local read "Position \nLock Status"() -> (w1178:bool)
    n469 = local read "Position \nLock Status"() -> (w1122:bool)
    n470 = local read "Search Step Size"() -> (w1169:u16)
    n471 = local read "Last Orientation"() -> (w1176:sgl)
    n472 = local read "Last Orientation"() -> (w1120:sgl)
    n473 = local read "Last Position"() -> (w1177:cluster{"X":sgl, "Y":sgl})
    n474 = local read "Last Position"() -> (w1121:cluster{"X":sgl, "Y":sgl})
    n475 = local read "Min Num Frames\nper Search"() -> (w1123:i32)
    n476 = call "Wait"("Count(mSec)"="Servo Algorithm\nCycle Time(ms)") -> ()  [unwired: 1 out]
    n477 = local read "Minimum Delta \nServo Threshold"() -> (w1131:i16)
    n478 = local read "Maximum Move \nServo Threshold"() -> (w1130:i16)
    n479 = local read "Search Step Size"() -> (w1128:u16)
    n480 = local read "New Data  Flag\nRight Servo"() -> (w1136:bool)
    n481 = local read "New Data  Flag\nLeft Servo"() -> (w1142:bool)
    n482 = local read "Image Lock - Right"() -> (w1138:bool)
    n483 = local read "Image Lock - Left"() -> (w1186:bool)
    n484 = local read "Tracking Angle - Right"() -> (w1135:sgl)
    n485 = local read "Tracking Angle - Left"() -> (w1184:sgl)
    n486 = local read "Current R (10bit)"() -> (w1134:u16)
    n487 = local read "Current L (10bit)"() -> (w1183:u16)
    n488 = case shown="True" w1136 {
      tunnel: [w1214 w1252] -> w1104
      tunnel: [w1208 w1251] -> w1115
      tunnel: w1141 -> [w1209 w1250]
      tunnel: w1138 -> [_ w1249]
      tunnel: "Track Angle Valid  - Right" -> [_ w1248]
      tunnel: w1135 -> [_ w1247]
      tunnel: w1134 -> [w1214 w1246]
      tunnel: "Mounting Offset - Right" -> [_ w1245]
      tunnel: w1129 -> [w1205 w1244]
      tunnel: w1127 -> [_ w1243]
      tunnel: w1124 -> [w1206 w1242]
      tunnel: w1122 -> [_ w1241]
      tunnel: w1121 -> [_ w1240]
      tunnel: w1120 -> [_ w1239]
      tunnel: w1119 -> [_ w1238]
      tunnel: w1117 -> [w1204 w1237]
      tunnel: w1126 -> [w1203 w1236]
      tunnel: w1125 -> [w1207 w1235]
      tunnel: w1131 -> [_ w1234]
      tunnel: w1130 -> [_ w1233]
      tunnel: w1128 -> [_ w1232]
      tunnel: [0 w1231] -> w1114
      tunnel: [w1209 w1230] -> w1116
      tunnel: [w1208 w1229] -> w1110
      tunnel: [w1207 w1228] -> w1109
      tunnel: [w1203 w1227] -> w1108
      tunnel: [w1206 w1226] -> w1107
      tunnel: [w1204 w1225] -> w1106
      tunnel: w1118 -> [_ w1224]
      tunnel: [w1205 w1223] -> w1105
      tunnel: w1123 -> [_ w1222]
      tunnel: w1133 -> [w1212 w1221]
      tunnel: w1139 -> [w1211 w1220]
      tunnel: [w1212 w1219] -> w1113
      tunnel: [w1211 w1218] -> w1111
      tunnel: w1140 -> [w1210 w1217]
      tunnel: [w1210 w1216] -> w1112
      frame False {
        w1208 = FALSE
        # "Recovery Mode COunt"
        # "Frames Processed - L"
        # "Recovery Search move Count - L"
        # "Recovery Search Attempt Count- L"
        # "WAITING FOR NEW IMAGE, RETAIN ALL VALUES"
      }
      frame True {
        w1254 = u16 1023
        w1257 = u16 0
        # "New Tracking State"
        # "Tracking Timeout Count"
        # "Next Main State"
        # "Next Recovery State"
        # "Reset Respond"
        # "Search Direction"
        # "Recovery Count"
        # "Recovery Search move Count"
        # "Recovery Search Attempt Count"
        # "Frames Processed"
        # "Apply Floor/Ceiling to Goal Position"
        # "Current move Delta"
        # "Service Track Angle Flag"
        # "Move Servo"
        # "Goal Position"
        # "Go to Current State"
        n489 = case shown="\"Recovery Mode\"" w1250 {
          tunnel: w1246 -> [w1276 w1353 w1531]
          tunnel: w1247 -> [_ w1355 _]
          tunnel: w1232 -> [w1275 _ w1526]
          tunnel: w1244 -> [w1274 w1335 w1520]
          tunnel: [w1273 w1351 w1530] -> w1258
          tunnel: [w1271 w1352 w1529] -> w1251
          tunnel: w1248 -> [w1269 w1346 w1507]
          tunnel: [w1268 w1348 w1516] -> w1230
          tunnel: w1249 -> [w1267 w1347 w1506]
          tunnel: w1245 -> [_ w1356 w1527]
          tunnel: w1234 -> [_ w1354 _]
          tunnel: [w1261 w1350 w1511] -> w1231
          tunnel: w1233 -> [_ w1349 _]
          tunnel: w1242 -> [w1266 _ w1521]
          tunnel: [enum16{"Generic Sweep", "Recovery Search"}."Recovery Search" enum16{"Generic Sweep", "Recovery Search"}."Recovery Search" w1528] -> w1216
          tunnel: w1237 -> [_ _ w1525]
          tunnel: w1217 -> [_ _ w1508]
          tunnel: w1243 -> [_ w1332 w1537]
          tunnel: w1224 -> [_ w1337 w1532]
          tunnel: w1239 -> [_ w1339 w1534]
          tunnel: w1240 -> [_ w1340 w1535]
          tunnel: w1241 -> [_ w1341 w1536]
          tunnel: w1238 -> [_ w1338 w1533]
          tunnel: [FALSE w1334 w1509] -> w1229
          tunnel: w1222 -> [w1265 _ w1519]
          tunnel: [w1261 w1329 w1518] -> w1225
          tunnel: [w1261 w1329 w1524] -> w1228
          tunnel: [w1261 w1329 w1523] -> w1227
          tunnel: [w1264 w1330 w1522] -> w1226
          tunnel: w1236 -> [_ _ w1514]
          tunnel: w1235 -> [_ _ w1513]
          tunnel: [w1262 w1335 w1512] -> w1223
          tunnel: w1221 -> [_ w1345 _]
          tunnel: [w1261 w1336 w1511] -> w1219
          tunnel: w1220 -> [_ w1342 _]
          tunnel: [enum16{"Track", "Reactive Predict", ""}."Track" ("Initial Tracking State - Right") w1333 enum16{"Track", "Reactive Predict", ""}."Track" ("Initial Tracking State - Right")] -> w1218
          frame "Start Up Search", Default {
            w1261 = u16 0
            # "Search Direction"
            # "Wait for 'x' Images to be Processed\nBefore Going to Next Step"
            # "Next Main State"
            # "New Goal Position"
            # "Move Servo"
            # "Choose Next State"
            # "Frames Processed Count"
            n490 = Greater Or Equal?(x=w1266, y=w1265) -> (x >= y?=w1272:bool)
            n491 = case shown="True" w1272 {
              tunnel: w1276 -> [w1291 w1303]
              tunnel: w1275 -> [_ w1301]
              tunnel: w1274 -> [w1290 w1300]
              tunnel: [w1291 w1297] -> w1273
              tunnel: [w1289 0] -> w1264
              tunnel: [FALSE TRUE] -> w1270
              tunnel: w1266 -> [w1292 _]
              tunnel: [w1290 w1294] -> w1262
              frame False {
                # "Increase Frames\nProcessed Count"
                n492 = Increment(x=w1292) -> (x+1=w1289:i32)
              }
              frame True {
                # "Reset Frames\nProcessed Count"
                # "SWEEP SEARCH - Startup"
                # "Multiple New Step\nby Step SIze"
                # "F = CCW\nT = CW"
                # "Last Direction"
                # "Min Step"
                # "add 10 in case\nactual position\nis lower than GP"
                # "Set New Step #"
                # "Choose Direction"
                # "Nearest step"
                # "Adjust Actual Posiiton\n to pre-determiend steps"
                # "Move Servo 1 \"Step\" to\nSearch"
                n493 = Add(x=3, y=w1303) -> (x+y=w1309:i32)
                n494 = Quotient & Remainder(x=w1309, y=w1301) -> (floor(x/y)=w1307:i32)  [unwired: 1 out]
                n495 = To Byte Integer(number=w1307) -> (8bit integer=w1298:i8)
                n496 = Less?(x=w1298, y=1) -> (x < y?=w1304:bool)
                n497 = case shown="False" w1304 {
                  tunnel: w1298 -> [w1320 w1328]
                  tunnel: [w1322 FALSE] -> w1294
                  tunnel: [w1321 w1328] -> w1306
                  tunnel: w1300 -> [w1319 _]
                  tunnel: w1301 -> [w1317 _]
                  frame False {
                    # "Max Step"
                    # "# of steps\nminus 1"
                    n498 = Divide(x=1024, y=w1317) -> (x/y=w1314:dbl)
                    n499 = To Unsigned Byte Integer(number=w1314) -> (unsigned 8bit integer=w1315:u8)
                    n500 = Greater Or Equal?(x=w1320, y=w1315) -> (x >= y?=w1316:bool)
                    n501 = case shown="True" w1316 {
                      tunnel: [w1323 TRUE] -> w1322
                      tunnel: [w1324 w1325] -> w1321
                      tunnel: w1320 -> [w1324 w1325]
                      tunnel: w1319 -> [w1323 _]
                      frame False {
                        # "No Need to\nChange Direction"
                      }
                      frame True {
                        # "T"
                        # "Move CW"
                      }
                    }
                  }
                  frame True {
                    # "F"
                    # "Move CCW"
                  }
                }
                n502 = case shown="False" w1294 {
                  tunnel: w1306 -> [w1311 w1312]
                  tunnel: [w1310 w1313] -> w1302
                  frame False {
                    # "CCW\n+1"
                    n503 = Increment(x=w1311) -> (x+1=w1310:i8)
                  }
                  frame True {
                    # "CW\n-1"
                    n504 = Decrement(x=w1312) -> (x-1=w1313:i8)
                  }
                }
                n505 = Multiply(x=w1302, y=w1301) -> (x*y=w1299:u16)
                n506 = To Unsigned Word Integer(number=w1299) -> (unsigned 16bit integer=w1297:u16)
              }
            }
            n507 = case shown="False" w1269 {
              tunnel: [w1280 FALSE] -> w1271
              tunnel: w1270 -> [w1280 _]
              tunnel: [w1281 w1286] -> w1268
              tunnel: w1267 -> [_ w1284]
              frame False {
                # "Check other Servo\nStay in Startup  State"
                n508 = local read "Track Angle Valid - Left"() -> (w1277:bool)
                n509 = local read "Image Lock - Left"() -> (w1278:bool)
                n510 = Or(x=w1277, y=w1278) -> (x .or. y?=w1279:bool)
                n511 = case shown="True" w1279 {
                  tunnel: [T2."Start Up Search" ("Next Main State") T2."Recovery Mode" ("Next Main State")] -> w1281
                  frame False {
                  }
                  frame True {
                  }
                }
              }
              frame True {
                # "Override Move Servo\nCommand bc an Angle Was Found\nduring this Step"
                # "Transition to Tracking State When\nImage Processing has Locked"
                n512 = case shown="False" w1284 {
                  tunnel: [T2."Start Up Search" ("Next Main State") T2."Tracking" ("Next Main State")] -> w1286
                  frame False {
                  }
                  frame True {
                  }
                }
              }
            }
          }
          frame "Tracking" {
            w1329 = 0
            # "Frames Processed Count"
            # "Image Lock - L"
            # "Track Angle Valid"
            # "Tracking Angle"
            # "Tracking Timeout Count"
            # "Max ove delta"
            # "Move delta threshold"
            # "mount offset"
            # "Current Position"
            # "Move Respond"
            # "Trackin Timeout count"
            # "Move Servo"
            # "delta"
            # "GP"
            # "Reset Move Respond"
            # "New Tracking State"
            # "Delta Move Sum"
            # "Choose Next State"
            n513 = case shown="\"Reactive Predict\"" w1342 {
              tunnel: w1356 -> [w1374 _]
              tunnel: w1355 -> [w1373 _]
              tunnel: w1354 -> [w1372 _]
              tunnel: w1353 -> [w1371 w1429]
              tunnel: [w1370 w1427] -> w1352
              tunnel: [w1369 w1435] -> w1351
              tunnel: [w1368 0] -> w1350
              tunnel: w1349 -> [w1367 _]
              tunnel: w1347 -> [w1366 w1419]
              tunnel: w1346 -> [w1365 w1422]
              tunnel: w1345 -> [w1364 w1424]
              tunnel: w1341 -> [_ w1434]
              tunnel: w1340 -> [_ w1433]
              tunnel: w1339 -> [_ w1432]
              tunnel: w1338 -> [_ w1431]
              tunnel: w1332 -> [_ w1430]
              tunnel: w1337 -> [_ w1428]
              tunnel: [TRUE w1425] -> w1334
              tunnel: [w1361 w1423] -> w1336
              tunnel: [w1359 w1421] -> w1333
              tunnel: [0 0] -> w1330
              frame "Track", Default {
                # "Reset"
                # "Tracking Timeout"
                # "Move Delta"
                # "Goal Position"
                # "Tracking Move"
                # "Move Servo"
                # "Only Consider Tracking Angle\n\nIF\n\nImage Locked        == T\nTrack Angle Flag   == T"
                n514 = And(x=w1366, y=w1365) -> (x .and. y?=w1358:bool)
                n515 = case shown="True" w1358 {
                  tunnel: w1374 -> [_ w1380]
                  tunnel: w1373 -> [_ w1398]
                  tunnel: w1372 -> [_ w1395]
                  tunnel: w1371 -> [w1377 w1385]
                  tunnel: [w1377 w1394] -> w1369
                  tunnel: [w1379 w1393] -> w1370
                  tunnel: [w1379 w1392] -> _
                  tunnel: [u16 0 w1391] -> w1368
                  tunnel: w1367 -> [_ w1387]
                  tunnel: w1364 -> [w1376 _]
                  tunnel: [w1375 0] -> w1361
                  frame False {
                    w1379 = FALSE
                    # "Increment timeout"
                    n516 = Increment(x=w1376) -> (x+1=w1375:i32)
                  }
                  frame True {
                    # "Convert Track Angle to UINT16"
                    # "1024/300"
                    # "Move to Tracking Angle \n\nif delta is greater than move servo threshold\nAND less than max move threshold"
                    n517 = Add(x=w1398, y=w1380) -> (x+y=w1401:sgl)
                    n518 = Add(x=w1401, y=sgl 60.0) -> (x+y=w1400:sgl)
                    n519 = Multiply(x=3.413333333333333, y=w1400) -> (x*y=w1381:dbl)
                    n520 = To Word Integer(number=w1385) -> (16bit integer=w1383:i16)
                    n521 = To Unsigned Word Integer(number=w1381) -> (unsigned 16bit integer=w1397:u16)
                    n522 = To Word Integer(number=w1381) -> (16bit integer=w1396:i16)
                    n523 = Subtract(x=w1396, y=w1383) -> (x-y=w1386:i16)
                    n524 = Absolute Value(x=w1386) -> (abs(x)=w1382:i16)
                    n525 = Greater Or Equal?(x=w1382, y=w1395) -> (x >= y?=w1389:bool)
                    n526 = Less Or Equal?(x=w1382, y=w1387) -> (x <= y?=w1388:bool)
                    n527 = And(x=w1389, y=w1388) -> (x .and. y?=w1390:bool)
                    n528 = case shown="True" w1390 {
                      tunnel: w1397 -> [_ w1409]
                      tunnel: [w1404 w1409] -> w1394
                      tunnel: [w1405 w1415] -> w1393
                      tunnel: [w1405 w1415] -> w1392
                      tunnel: w1385 -> [w1404 _]
                      tunnel: w1382 -> [_ w1414]
                      tunnel: [u16 0 w1414] -> w1391
                      tunnel: w1380 -> [_ w1408]
                      frame False {
                        w1405 = FALSE
                        # "Don't Move"
                      }
                      frame True {
                        w1415 = TRUE
                        # "45 DEG MOUNT OFFSET"
                        # "1024/300"
                        # "Current Delta"
                        # "Use new Track Angle"
                        n529 = Divide(x=w1409, y=3.413333333333333) -> (x/y=w1411:dbl)
                        n530 = Negate(x=w1408) -> (-x=w1407:sgl)
                        n531 = Subtract(x=w1411, y=sgl 60.0) -> (x-y=w1413:dbl)
                        n532 = Add(x=w1413, y=w1407) -> (x+y=w1406:dbl)
                        n533 = local write "Last Track Angle - R"(w1406) -> ()
                      }
                    }
                  }
                }
                n534 = local read "Timeout to \nEnable Reactive Predict"() -> (w1362:u16)
                n535 = Less?(x=w1361, y=w1362) -> (x < y?=w1360:bool)
                n536 = case shown="False" w1360 {
                  tunnel: [enum16{"Track", "Reactive Predict", ""}."Reactive Predict" ("Initial Tracking State - Right") enum16{"Track", "Reactive Predict", ""}."Track" ("Initial Tracking State - Right")] -> w1359
                  frame False {
                  }
                  frame True {
                  }
                }
              }
              frame "Reactive Predict" {
                # "Choose New\nTracking State"
                n537 = Or(x=w1419, y=w1422) -> (x .or. y?=w1418:bool)
                n538 = case shown="False" w1418 {
                  tunnel: [w1448 w1500] -> w1435
                  tunnel: w1434 -> [w1447 _]
                  tunnel: w1433 -> [w1446 _]
                  tunnel: w1432 -> [w1445 _]
                  tunnel: w1431 -> [w1444 _]
                  tunnel: w1430 -> [w1443 _]
                  tunnel: w1428 -> [w1442 _]
                  tunnel: [w1441 w1499] -> w1427
                  tunnel: [w1440 w1499] -> w1425
                  tunnel: w1424 -> [w1439 _]
                  tunnel: [w1438 0] -> w1423
                  tunnel: [enum16{"Track", "Reactive Predict", ""}."Reactive Predict" ("Initial Tracking State - Right") enum16{"Track", "Reactive Predict", ""}."Track" ("Initial Tracking State - Right")] -> w1421
                  tunnel: w1429 -> [w1436 w1500]
                  frame False {
                    # "Stay in Reactive State"
                    # "Increment Track Timeout"
                    # "Move Respond Flag"
                    n539 = Increment(x=w1439) -> (x+1=w1438:i32)
                    n540 = case shown="True" w1443 {
                      tunnel: w1447 -> [_ w1463]
                      tunnel: w1446 -> [_ w1462]
                      tunnel: w1445 -> [_ w1461]
                      tunnel: w1444 -> [_ w1460]
                      tunnel: w1442 -> [_ w1457]
                      tunnel: [w1449 w1453] -> w1448
                      tunnel: [w1450 w1452] -> w1441
                      tunnel: [w1450 w1452] -> w1440
                      tunnel: w1436 -> [w1449 w1451]
                      frame False {
                        w1450 = FALSE
                        # "Reset Move Respond = F"
                        # "Move Servo = F"
                      }
                      frame True {
                        w1452 = TRUE
                        # "Position Lock"
                        # "Current Servo\nPosition"
                        # "Reset Move\nRespond = T"
                        # "Move Servo = T"
                        # "Apply Direction \nto Offset (delta sum)"
                        # "Check Last Known Position of Robot"
                        n541 = case shown="True" w1463 {
                          tunnel: w1462 -> [_ w1491]
                          tunnel: w1461 -> [_ w1466]
                          tunnel: w1460 -> [_ w1467]
                          tunnel: [sgl 1.0 ("y") w1465] -> w1459
                          frame False {
                            # "No Position Data Available"
                            # "Default is to move\nSame Direction as other\nServo"
                          }
                          frame True {
                            w1472 = sgl 1.0 ("y")
                            # "Use previous position/orientation to Guess Which Direction to Move Servo"
                            # "Choose Search Direction"
                            # "\"Perpendicular \nThreshold\""
                            # "If Orientation is\n ~Perpendicular -> Start Search\n in Opposite Direction of Other"
                            # "****add 90 until orientation angle is fixed"
                            # "Last Orientation"
                            # "Convert to Rad"
                            # "Avoid Divide by 0"
                            # "-1/m"
                            # "Calculate Normal Line to \nLast Robot Position\nfrom Center Beacon"
                            # "last Position \nCoordinates"
                            n542 = Unbundle(w1491) -> ("X"=w1471:sgl, "Y"=w1470:sgl)
                            n543 = Unbundle(w1467) -> ("X"=w1469:sgl, "Y"=w1468:sgl)
                            n544 = Subtract(x=w1470, y=w1468) -> (x-y=w1487:sgl)
                            n545 = Subtract(x=w1471, y=w1469) -> (x-y=w1485:sgl)
                            n546 = Equal To 0?(x=w1485) -> (x = 0?=w1486:bool)
                            n547 = case shown="False" w1486 {
                              tunnel: w1487 -> [w1494 _]
                              tunnel: w1485 -> [w1493 _]
                              tunnel: [w1492 1000000000000000.0] -> w1484
                              frame False {
                                n548 = Divide(x=w1494, y=w1493) -> (x/y=w1492:sgl)
                              }
                              frame True {
                              }
                            }
                            n549 = Equal To 0?(x=w1484) -> (x = 0?=w1489:bool)
                            n550 = case shown="False" w1489 {
                              tunnel: [w1496 1e-08] -> w1488
                              tunnel: w1484 -> [w1496 _]
                              frame False {
                              }
                              frame True {
                                # "Can't have infinit slope"
                              }
                            }
                            n551 = Divide(x=-1.0, y=w1488) -> (x/y=w1483:dbl)
                            n552 = Inverse Tangent(1:w1483) -> (0:w1481:dbl)
                            n553 = expression code="(x/pi)*180.0" "radians to degrees"(w1481) -> (w1482:dbl)
                            n554 = To Single Precision Float(number=w1482) -> (single precision float=w1479:sgl)
                            n555 = Add(x=w1466, y=sgl 90.0) -> (x+y=w1478:sgl)
                            n556 = Subtract(x=w1479, y=w1478) -> (x-y=w1477:sgl)
                            n557 = Absolute Value(x=w1477) -> (abs(x)=w1476:sgl)
                            n558 = Less Or Equal?(x=w1476, y=sgl 10.0) -> (x <= y?=w1474:bool)
                            n559 = Negate(x=w1472) -> (-x=w1473:sgl)
                            n560 = Select(t=w1473, s=w1474, f=w1472) -> (s? t:f=w1465:sgl)
                          }
                        }
                        n561 = To Word Integer(number=w1459) -> (16bit integer=w1458:i16)
                        n562 = Multiply(x=w1458, y=w1457) -> (x*y=w1456:i32)
                        n563 = To Word Integer(number=w1451) -> (16bit integer=w1455:i16)
                        n564 = Add(x=w1456, y=w1455) -> (x+y=w1454:i32)
                        n565 = To Unsigned Word Integer(number=w1454) -> (unsigned 16bit integer=w1453:u16)
                      }
                    }
                  }
                  frame True {
                    w1499 = TRUE
                    # "Go Directly to Track State"
                  }
                }
              }
            }
            n566 = local read "Tracking Timeout\nThreshold"() -> (w1343:i32)
            n567 = Less?(x=w1336, y=w1343) -> (x < y?=w1344:bool)
            n568 = case shown="False" w1344 {
              tunnel: [T2."Recovery Mode" ("Next Main State") T2."Tracking" ("Next Main State")] -> w1348
              frame False {
              }
              frame True {
              }
            }
          }
          frame "Recovery Mode" {
            w1511 = u16 0
            # "Increment Recovery Mode Count"
            # "Recovvery Mode\nCount"
            # "Frames Processed"
            # "Choose Next Main State"
            # "Reset recovery count"
            # "Recovery move\nCount"
            # "Recovery Search\nAttempt count"
            # "Move Servo = T"
            # "delta move sum"
            # "Robot Position Valid"
            n569 = local read "Image Lock - Left"() -> (w1515:bool)
            n570 = Or(x=w1506, y=w1507) -> (x .or. y?=w1505:bool)
            n571 = case shown="\"Recovery Search\"" w1508 {
              tunnel: w1537 -> [_ _]
              tunnel: w1536 -> [_ _]
              tunnel: w1535 -> [_ _]
              tunnel: w1534 -> [_ _]
              tunnel: w1533 -> [_ _]
              tunnel: w1532 -> [_ _]
              tunnel: w1531 -> [w1565 w1651]
              tunnel: [w1557 w1649] -> w1530
              tunnel: [w1554 w1643] -> w1529
              tunnel: [FALSE FALSE] -> w1509
              tunnel: [w1559 w1640] -> w1528
              tunnel: w1525 -> [w1563 _]
              tunnel: w1527 -> [w1566 _]
              tunnel: w1526 -> [w1564 w1646]
              tunnel: [w1556 w1639] -> w1523
              tunnel: [w1555 w1639] -> w1524
              tunnel: w1515 -> [w1553 _]
              tunnel: [w1544 w1650] -> w1522
              tunnel: w1521 -> [w1542 w1634]
              tunnel: w1520 -> [w1547 w1647]
              tunnel: w1519 -> [w1543 w1645]
              tunnel: w1506 -> [_ _]
              tunnel: w1507 -> [_ w1642]
              tunnel: [FALSE w1641] -> w1517
              tunnel: w1514 -> [w1551 _]
              tunnel: w1513 -> [w1550 _]
              tunnel: [w1547 w1638] -> w1512
              frame "Recovery Search" {
                # "Wait for 2 Images to be Processed\nBefore Going to Next Step"
                # "Choose Next Reovery State"
                # "Recovery Search \nAttempt Count"
                # "Move Servo"
                # "Goal Position"
                # "Recovery Search\nmove Count"
                # "Attempt Recovery Search if Other Servo has Valid Angle"
                n572 = local read "Last Track Angle - L"() -> (w1546:sgl)
                n573 = Greater Or Equal?(x=w1542, y=w1543) -> (x >= y?=w1545:bool)
                n574 = case shown="True" w1545 {
                  tunnel: w1566 -> [_ w1586]
                  tunnel: [w1571 w1585] -> w1555
                  tunnel: w1565 -> [w1574 w1584]
                  tunnel: w1564 -> [_ w1583]
                  tunnel: [w1572 w1582] -> w1556
                  tunnel: [w1574 w1581] -> w1557
                  tunnel: [FALSE w1580] -> w1554
                  tunnel: w1551 -> [w1572 w1579]
                  tunnel: w1550 -> [w1571 w1578]
                  tunnel: w1553 -> [_ w1577]
                  tunnel: w1546 -> [_ w1576]
                  tunnel: [w1569 0 ("Frames Processed\nCount - in")] -> w1544
                  tunnel: w1542 -> [w1570 _]
                  frame False {
                    # "Increment Frames Processed"
                    # "WAIT"
                    n575 = Increment(x=w1570) -> (x+1=w1569:i32)
                  }
                  frame True {
                    n576 = case shown="True" w1577 {
                      tunnel: w1576 -> [_ w1599]
                      tunnel: w1579 -> [w1587 w1595]
                      tunnel: w1586 -> [_ w1600]
                      tunnel: [w1590 w1598] -> w1581
                      tunnel: [w1588 w1597] -> w1585
                      tunnel: w1578 -> [w1588 w1596]
                      tunnel: w1584 -> [w1590 w1594]
                      tunnel: w1583 -> [_ w1593]
                      tunnel: [FALSE TRUE] -> w1580
                      tunnel: [w1587 w1591] -> w1582
                      frame False {
                        # "Don't Move bc Other Servo Doesn't Have Image Lock"
                      }
                      frame True {
                        # "Move Servo = T"
                        n577 = Greater Than 0?(x=w1595) -> (x > 0?=w1601:bool)
                        n578 = case shown="False" w1601 {
                          tunnel: w1600 -> [w1608 _]
                          tunnel: w1599 -> [w1602 _]
                          tunnel: [w1607 w1618] -> w1598
                          tunnel: [w1605 w1624] -> w1597
                          tunnel: w1596 -> [w1606 w1624]
                          tunnel: w1595 -> [w1604 w1621]
                          tunnel: [w1603 w1623] -> w1591
                          tunnel: w1594 -> [_ w1619]
                          tunnel: w1593 -> [_ w1616]
                          frame False {
                            # "Increment move count to transition\nto Pan mode"
                            # "Increment Recovery Search Attempt Count"
                            # "1024/300"
                            # "Move Parallel to Other Servo"
                            n579 = Increment(x=w1606) -> (x+1=w1605:i32)
                            n580 = Add(x=w1602, y=w1608) -> (x+y=w1614:sgl)
                            n581 = Add(x=w1614, y=sgl 60.0) -> (x+y=w1613:sgl)
                            n582 = Multiply(x=3.413333333333333, y=w1613) -> (x*y=w1611:dbl)
                            n583 = Add(x=0.5, y=w1611) -> (x+y=w1609:dbl)
                            n584 = To Unsigned Word Integer(number=w1609) -> (unsigned 16bit integer=w1607:u16)
                            n585 = Increment(x=w1604) -> (x+1=w1603:i32)
                          }
                          frame True {
                            # "Apply Direction"
                            # "Step SIze"
                            # "Current Position"
                            # "Attempt to Pan in Steps Towards other Servo"
                            # "Could be same or function of \nregular search step size"
                            # "Max # of Pan\nMoves"
                            # "Pan Towards Other Servo"
                            n586 = Greater Or Equal?(x=w1621, y=u16 20) -> (x >= y?=w1622:bool)
                            n587 = case shown="False" w1622 {
                              tunnel: w1621 -> [w1632 _]
                              tunnel: [w1631 u16 0] -> w1623
                              frame False {
                                # "Increment Pan Count"
                                n588 = Increment(x=w1632) -> (x+1=w1631:i32)
                              }
                              frame True {
                                # "Reset move count"
                              }
                            }
                            n589 = local read "Recovery Search\nDirection - R"() -> (w1617:bool)
                            n590 = case shown="False" w1617 {
                              tunnel: w1619 -> [w1626 w1630]
                              tunnel: w1616 -> [w1627 w1629]
                              tunnel: [w1625 w1628] -> w1618
                              frame False {
                                # "CCW"
                                n591 = Add(x=w1626, y=w1627) -> (x+y=w1625:u16)
                              }
                              frame True {
                                # "CW"
                                n592 = Subtract(x=w1630, y=w1629) -> (x-y=w1628:u16)
                              }
                            }
                          }
                        }
                      }
                    }
                  }
                }
                n593 = local read "Max Recovery Count\n(Recovery Search)"() -> (w1548:u16)
                n594 = local read "Max Recovery\nSearch Attempts"() -> (w1549:u16)
                n595 = Less Or Equal?(x=w1555, y=w1549) -> (x <= y?=w1561:bool)
                n596 = Less Or Equal?(x=w1563, y=w1548) -> (x <= y?=w1562:bool)
                n597 = And(x=w1561, y=w1562) -> (x .and. y?=w1560:bool)
                n598 = case shown="True" w1560 {
                  tunnel: [enum16{"Generic Sweep", "Recovery Search"}."Generic Sweep" enum16{"Generic Sweep", "Recovery Search"}."Recovery Search"] -> w1559
                  frame False {
                  }
                  frame True {
                  }
                }
              }
              frame "Generic Sweep" {
                w1639 = u16 0
                # "Angle Valid?"
                # "Choose Next Recovery State"
                # "Wait for 2 Images to be Processed\nBefore Going to Next Step"
                # "New Goal Position"
                # "Move Servo"
                # "Frames Processed Count"
                n599 = Greater Or Equal?(x=w1634, y=w1645) -> (x >= y?=w1652:bool)
                n600 = case shown="True" w1652 {
                  tunnel: w1651 -> [w1668 w1680]
                  tunnel: w1646 -> [_ w1678]
                  tunnel: w1647 -> [w1667 w1677]
                  tunnel: [w1668 w1674] -> w1649
                  tunnel: [w1666 0] -> w1650
                  tunnel: [FALSE TRUE] -> w1644
                  tunnel: w1634 -> [w1669 _]
                  tunnel: [w1667 w1671] -> w1638
                  frame False {
                    # "Increment Frames Processed"
                    n601 = Increment(x=w1669) -> (x+1=w1666:i32)
                  }
                  frame True {
                    # "Reset Frames\nProcessed Count"
                    # "SWEEP SEARCH - Startup"
                    # "Multiple New Step\nby Step SIze"
                    # "F = CCW\nT = CW"
                    # "Last Direction"
                    # "Min Step"
                    # "add 10 in case\nactual position\nis lower than GP"
                    # "Set New Step #"
                    # "Choose Direction"
                    # "Nearest step"
                    # "Adjust Actual Posiiton\n to pre-determiend steps"
                    # "Move Servo 1 \"Step\" to\nSearch"
                    n602 = Add(x=5, y=w1680) -> (x+y=w1686:i32)
                    n603 = Quotient & Remainder(x=w1686, y=w1678) -> (floor(x/y)=w1684:i32)  [unwired: 1 out]
                    n604 = To Byte Integer(number=w1684) -> (8bit integer=w1675:i8)
                    n605 = Less?(x=w1675, y=1) -> (x < y?=w1681:bool)
                    n606 = case shown="False" w1681 {
                      tunnel: w1675 -> [w1697 w1705]
                      tunnel: [w1699 FALSE] -> w1671
                      tunnel: [w1698 w1705] -> w1683
                      tunnel: w1677 -> [w1696 _]
                      tunnel: w1678 -> [w1694 _]
                      frame False {
                        # "Max Step"
                        # "# of steps\nminus 1"
                        n607 = Divide(x=1024, y=w1694) -> (x/y=w1691:dbl)
                        n608 = To Unsigned Byte Integer(number=w1691) -> (unsigned 8bit integer=w1692:u8)
                        n609 = Greater Or Equal?(x=w1697, y=w1692) -> (x >= y?=w1693:bool)
                        n610 = case shown="True" w1693 {
                          tunnel: [w1700 TRUE] -> w1699
                          tunnel: [w1701 w1702] -> w1698
                          tunnel: w1697 -> [w1701 w1702]
                          tunnel: w1696 -> [w1700 _]
                          frame False {
                            # "No Need to\nChange Direction"
                          }
                          frame True {
                            # "T"
                            # "Move CW"
                          }
                        }
                      }
                      frame True {
                        # "F"
                        # "Move CCW"
                      }
                    }
                    n611 = case shown="True" w1671 {
                      tunnel: w1683 -> [w1688 w1689]
                      tunnel: [w1687 w1690] -> w1679
                      frame False {
                        # "CCW\n+1"
                        n612 = Increment(x=w1688) -> (x+1=w1687:i8)
                      }
                      frame True {
                        # "CW\n-1"
                        n613 = Decrement(x=w1689) -> (x-1=w1690:i8)
                      }
                    }
                    n614 = Multiply(x=w1679, y=w1678) -> (x*y=w1676:u16)
                    n615 = To Unsigned Word Integer(number=w1676) -> (unsigned 16bit integer=w1674:u16)
                  }
                }
                n616 = local read "Track Angle Valid - Left"() -> (w1637:bool)
                n617 = local read "Image Lock - Left"() -> (w1636:bool)
                n618 = Or(x=w1636, y=w1637) -> (x .or. y?=w1635:bool)
                n619 = case shown="False" w1642 {
                  tunnel: [w1655 w1665] -> w1643
                  tunnel: w1644 -> [w1656 _]
                  tunnel: [w1657 enum16{"Generic Sweep", "Recovery Search"}."Generic Sweep"] -> w1640
                  tunnel: [w1654 w1665] -> w1641
                  tunnel: w1635 -> [w1653 _]
                  frame False {
                    # "Is other servo tracking?"
                    n620 = case shown="True" w1653 {
                      tunnel: [enum16{"Generic Sweep", "Recovery Search"}."Generic Sweep" enum16{"Generic Sweep", "Recovery Search"}."Recovery Search"] -> w1657
                      tunnel: w1656 -> [w1660 _]
                      tunnel: [w1660 FALSE] -> w1655
                      tunnel: [FALSE TRUE] -> w1654
                      frame False {
                        # "Stay in Sweep"
                      }
                      frame True {
                        # "G o to Recovery Search  State"
                      }
                    }
                  }
                  frame True {
                    w1665 = FALSE
                    # "Override Move Servo\nCommand bc an Angle Was Found\nduring this Step"
                    # "Stay In Sweep\nLet Main State Machine transition\ninto Tracking"
                  }
                }
              }
            }
            n621 = Increment(x=w1525) -> (x+1=w1504:i32)
            n622 = case shown="True" w1517 {
              tunnel: w1504 -> [w1540 _]
              tunnel: [w1540 0] -> w1518
              frame False {
              }
              frame True {
              }
            }
            n623 = case shown="False" w1505 {
              tunnel: [T2."Recovery Mode" ("Next Main State") T2."Tracking" ("Next Main State")] -> w1516
              frame False {
              }
              frame True {
              }
            }
          }
        }
        "Current Move Delta - L 2" <- w1231
        n624 = Less?(x=w1258, y=w1257) -> (x < y?=w1256:bool)
        n625 = local write "New Data  Flag\nRight Servo"(FALSE) -> ()
        n626 = Select(t=w1257, s=w1256, f=w1258) -> (s? t:f=w1253:u16)
        n627 = Greater?(x=w1253, y=w1254) -> (0:w1255:bool)
        n628 = Select(t=w1254, s=w1255, f=w1253) -> (s? t:f=w1252:u16)
      }
    }
    "Next Main State - Right" <- w1116
    "Next Tracking State - Right" <- w1111
    "Next Recovery State - Right" <- w1112
    n629 = case shown="True" w1142 {
      tunnel: [w1717 w1755] -> w1189
      tunnel: [w1711 w1754] -> w1188
      tunnel: w1187 -> [w1712 w1753]
      tunnel: w1186 -> [_ w1752]
      tunnel: "Track Angle Valid - Left" -> [_ w1751]
      tunnel: w1184 -> [_ w1750]
      tunnel: w1183 -> [w1717 w1749]
      tunnel: "Mounting Offset - Left" -> [_ w1748]
      tunnel: w1181 -> [w1708 w1747]
      tunnel: w1180 -> [_ w1746]
      tunnel: w1179 -> [w1709 w1745]
      tunnel: w1178 -> [_ w1744]
      tunnel: w1177 -> [_ w1743]
      tunnel: w1176 -> [_ w1742]
      tunnel: "Middle Beacon\nCoordinates" -> [_ w1741]
      tunnel: w1174 -> [w1707 w1740]
      tunnel: w1173 -> [w1706 w1739]
      tunnel: w1172 -> [w1710 w1738]
      tunnel: w1171 -> [_ w1737]
      tunnel: w1170 -> [_ w1736]
      tunnel: w1169 -> [_ w1735]
      tunnel: [0 w1734] -> w1163
      tunnel: [w1712 w1733] -> w1162
      tunnel: [w1711 w1732] -> w1161
      tunnel: [w1710 w1731] -> w1160
      tunnel: [w1706 w1730] -> w1159
      tunnel: [w1709 w1729] -> w1158
      tunnel: [w1707 w1728] -> w1157
      tunnel: w1155 -> [_ w1727]
      tunnel: [w1708 w1726] -> w1154
      tunnel: w1152 -> [_ w1725]
      tunnel: w1148 -> [w1715 w1724]
      tunnel: w1147 -> [w1714 w1723]
      tunnel: [w1715 w1722] -> w1146
      tunnel: [w1714 w1721] -> w1145
      tunnel: w1144 -> [w1713 w1720]
      tunnel: [w1713 w1719] -> w1143
      frame False {
        w1711 = FALSE
        # "Recovery Mode COunt"
        # "Frames Processed - L"
        # "Recovery Search move Count - L"
        # "Recovery Search Attempt Count- L"
        # "WAITING FOR NEW IMAGE, RETAIN ALL VALUES"
      }
      frame True {
        w1757 = u16 1023
        w1760 = u16 0
        # "New Tracking State"
        # "Tracking Timeout Count"
        # "Next Main State"
        # "Next Recovery State"
        # "Reset Respond"
        # "Search Direction"
        # "Recovery Count"
        # "Recovery Search move Count"
        # "Recovery Search Attempt Count"
        # "Frames Processed"
        # "Apply Floor/Ceiling to Goal Position"
        # "Current move Delta"
        # "Service Track Angle Flag"
        # "Move Servo"
        # "Goal Position"
        # "Go to Current State"
        n630 = case shown="\"Recovery Mode\"" w1753 {
          tunnel: w1749 -> [w1779 w1856 w2034]
          tunnel: w1750 -> [_ w1858 _]
          tunnel: w1735 -> [w1778 _ w2029]
          tunnel: w1747 -> [w1777 w1838 w2023]
          tunnel: [w1776 w1854 w2033] -> w1761
          tunnel: [w1774 w1855 w2032] -> w1754
          tunnel: w1751 -> [w1772 w1849 w2010]
          tunnel: [w1771 w1851 w2019] -> w1733
          tunnel: w1752 -> [w1770 w1850 w2009]
          tunnel: w1748 -> [_ w1859 w2030]
          tunnel: w1737 -> [_ w1857 _]
          tunnel: [w1764 w1853 w2014] -> w1734
          tunnel: w1736 -> [_ w1852 _]
          tunnel: w1745 -> [w1769 _ w2024]
          tunnel: [enum16{"Generic Sweep", "Recovery Search"}."Recovery Search" enum16{"Generic Sweep", "Recovery Search"}."Recovery Search" w2031] -> w1719
          tunnel: w1740 -> [_ _ w2028]
          tunnel: w1720 -> [_ _ w2011]
          tunnel: w1746 -> [_ w1835 w2040]
          tunnel: w1727 -> [_ w1840 w2035]
          tunnel: w1742 -> [_ w1842 w2037]
          tunnel: w1743 -> [_ w1843 w2038]
          tunnel: w1744 -> [_ w1844 w2039]
          tunnel: w1741 -> [_ w1841 w2036]
          tunnel: [FALSE w1837 w2012] -> w1732
          tunnel: w1725 -> [w1768 _ w2022]
          tunnel: [w1764 w1832 w2021] -> w1728
          tunnel: [w1764 w1832 w2027] -> w1731
          tunnel: [w1764 w1832 w2026] -> w1730
          tunnel: [w1767 w1833 w2025] -> w1729
          tunnel: w1739 -> [_ _ w2017]
          tunnel: w1738 -> [_ _ w2016]
          tunnel: [w1765 w1838 w2015] -> w1726
          tunnel: w1724 -> [_ w1848 _]
          tunnel: [w1764 w1839 w2014] -> w1722
          tunnel: w1723 -> [_ w1845 _]
          tunnel: [enum16{"Track", "Reactive Predict", ""}."Track" ("Initial Tracking State - Right") w1836 enum16{"Track", "Reactive Predict", ""}."Track" ("Initial Tracking State - Right")] -> w1721
          frame "Start Up Search", Default {
            w1764 = u16 0
            # "Search Direction"
            # "Wait for 'x' Images to be Processed\nBefore Going to Next Step"
            # "Next Main State"
            # "New Goal Position"
            # "Move Servo"
            # "Choose Next State"
            # "Frames Processed Count"
            n631 = Greater Or Equal?(x=w1769, y=w1768) -> (x >= y?=w1775:bool)
            n632 = case shown="True" w1775 {
              tunnel: w1779 -> [w1794 w1806]
              tunnel: w1778 -> [_ w1804]
              tunnel: w1777 -> [w1793 w1803]
              tunnel: [w1794 w1800] -> w1776
              tunnel: [w1792 0] -> w1767
              tunnel: [FALSE TRUE] -> w1773
              tunnel: w1769 -> [w1795 _]
              tunnel: [w1793 w1797] -> w1765
              frame False {
                # "Increase Frames\nProcessed Count"
                n633 = Increment(x=w1795) -> (x+1=w1792:i32)
              }
              frame True {
                # "Reset Frames\nProcessed Count"
                # "SWEEP SEARCH - Startup"
                # "Multiple New Step\nby Step SIze"
                # "F = CCW\nT = CW"
                # "Last Direction"
                # "Min Step"
                # "add 10 in case\nactual position\nis lower than GP"
                # "Set New Step #"
                # "Choose Direction"
                # "Nearest step"
                # "Adjust Actual Posiiton\n to pre-determiend steps"
                # "Move Servo 1 \"Step\" to\nSearch"
                n634 = Add(x=3, y=w1806) -> (x+y=w1812:i32)
                n635 = Quotient & Remainder(x=w1812, y=w1804) -> (floor(x/y)=w1810:i32)  [unwired: 1 out]
                n636 = To Byte Integer(number=w1810) -> (8bit integer=w1801:i8)
                n637 = Less?(x=w1801, y=1) -> (x < y?=w1807:bool)
                n638 = case shown="False" w1807 {
                  tunnel: w1801 -> [w1823 w1831]
                  tunnel: [w1825 FALSE] -> w1797
                  tunnel: [w1824 w1831] -> w1809
                  tunnel: w1803 -> [w1822 _]
                  tunnel: w1804 -> [w1820 _]
                  frame False {
                    # "Max Step"
                    # "# of steps\nminus 1"
                    n639 = Divide(x=1024, y=w1820) -> (x/y=w1817:dbl)
                    n640 = To Unsigned Byte Integer(number=w1817) -> (unsigned 8bit integer=w1818:u8)
                    n641 = Greater Or Equal?(x=w1823, y=w1818) -> (x >= y?=w1819:bool)
                    n642 = case shown="True" w1819 {
                      tunnel: [w1826 TRUE] -> w1825
                      tunnel: [w1827 w1828] -> w1824
                      tunnel: w1823 -> [w1827 w1828]
                      tunnel: w1822 -> [w1826 _]
                      frame False {
                        # "No Need to\nChange Direction"
                      }
                      frame True {
                        # "T"
                        # "Move CW"
                      }
                    }
                  }
                  frame True {
                    # "F"
                    # "Move CCW"
                  }
                }
                n643 = case shown="False" w1797 {
                  tunnel: w1809 -> [w1814 w1815]
                  tunnel: [w1813 w1816] -> w1805
                  frame False {
                    # "CCW\n+1"
                    n644 = Increment(x=w1814) -> (x+1=w1813:i8)
                  }
                  frame True {
                    # "CW\n-1"
                    n645 = Decrement(x=w1815) -> (x-1=w1816:i8)
                  }
                }
                n646 = Multiply(x=w1805, y=w1804) -> (x*y=w1802:u16)
                n647 = To Unsigned Word Integer(number=w1802) -> (unsigned 16bit integer=w1800:u16)
              }
            }
            n648 = case shown="False" w1772 {
              tunnel: [w1783 FALSE] -> w1774
              tunnel: w1773 -> [w1783 _]
              tunnel: [w1784 w1789] -> w1771
              tunnel: w1770 -> [_ w1787]
              frame False {
                # "Check other Servo\nStay in Startup  State"
                n649 = local read "Track Angle Valid  - Right"() -> (w1780:bool)
                n650 = local read "Image Lock - Right"() -> (w1781:bool)
                n651 = Or(x=w1780, y=w1781) -> (x .or. y?=w1782:bool)
                n652 = case shown="True" w1782 {
                  tunnel: [T2."Start Up Search" ("Next Main State") T2."Recovery Mode" ("Next Main State")] -> w1784
                  frame False {
                  }
                  frame True {
                  }
                }
              }
              frame True {
                # "Override Move Servo\nCommand bc an Angle Was Found\nduring this Step"
                # "Transition to Tracking State When\nImage Processing has Locked"
                n653 = case shown="False" w1787 {
                  tunnel: [T2."Start Up Search" ("Next Main State") T2."Tracking" ("Next Main State")] -> w1789
                  frame False {
                  }
                  frame True {
                  }
                }
              }
            }
          }
          frame "Tracking" {
            w1832 = 0
            # "Frames Processed Count"
            # "Image Lock - L"
            # "Track Angle Valid"
            # "Tracking Angle"
            # "Tracking Timeout Count"
            # "Max ove delta"
            # "Move delta threshold"
            # "mount offset"
            # "Current Position"
            # "Move Respond"
            # "Trackin Timeout count"
            # "Move Servo"
            # "delta"
            # "GP"
            # "Reset Move Respond"
            # "New Tracking State"
            # "Delta Move Sum"
            # "Choose Next State"
            n654 = case shown="\"Track\", Default" w1845 {
              tunnel: w1859 -> [w1877 _]
              tunnel: w1858 -> [w1876 _]
              tunnel: w1857 -> [w1875 _]
              tunnel: w1856 -> [w1874 w1932]
              tunnel: [w1873 w1930] -> w1855
              tunnel: [w1872 w1938] -> w1854
              tunnel: [w1871 0] -> w1853
              tunnel: w1852 -> [w1870 _]
              tunnel: w1850 -> [w1869 w1922]
              tunnel: w1849 -> [w1868 w1925]
              tunnel: w1848 -> [w1867 w1927]
              tunnel: w1844 -> [_ w1937]
              tunnel: w1843 -> [_ w1936]
              tunnel: w1842 -> [_ w1935]
              tunnel: w1841 -> [_ w1934]
              tunnel: w1835 -> [_ w1933]
              tunnel: w1840 -> [_ w1931]
              tunnel: [TRUE w1928] -> w1837
              tunnel: [w1864 w1926] -> w1839
              tunnel: [w1862 w1924] -> w1836
              tunnel: [0 0] -> w1833
              frame "Track", Default {
                # "Reset"
                # "Tracking Timeout"
                # "Move Delta"
                # "Goal Position"
                # "Tracking Move"
                # "Move Servo"
                # "Only Consider Tracking Angle\n\nIF\n\nImage Locked        == T\nTrack Angle Flag   == T"
                n655 = And(x=w1869, y=w1868) -> (x .and. y?=w1861:bool)
                n656 = case shown="True" w1861 {
                  tunnel: w1877 -> [_ w1883]
                  tunnel: w1876 -> [_ w1901]
                  tunnel: w1875 -> [_ w1898]
                  tunnel: w1874 -> [w1880 w1888]
                  tunnel: [w1880 w1897] -> w1872
                  tunnel: [w1882 w1896] -> w1873
                  tunnel: [w1882 w1895] -> _
                  tunnel: [u16 0 w1894] -> w1871
                  tunnel: w1870 -> [_ w1890]
                  tunnel: w1867 -> [w1879 _]
                  tunnel: [w1878 0] -> w1864
                  frame False {
                    w1882 = FALSE
                    # "Increment timeout"
                    n657 = Increment(x=w1879) -> (x+1=w1878:i32)
                  }
                  frame True {
                    # "Convert Track Angle to UINT16"
                    # "1024/300"
                    # "Move to Tracking Angle \n\nif delta is greater than move servo threshold\nAND less than max move threshold"
                    n658 = Add(x=w1901, y=w1883) -> (x+y=w1904:sgl)
                    n659 = Add(x=w1904, y=sgl 60.0) -> (x+y=w1903:sgl)
                    n660 = Multiply(x=3.413333333333333, y=w1903) -> (x*y=w1884:dbl)
                    n661 = To Word Integer(number=w1888) -> (16bit integer=w1886:i16)
                    n662 = To Unsigned Word Integer(number=w1884) -> (unsigned 16bit integer=w1900:u16)
                    n663 = To Word Integer(number=w1884) -> (16bit integer=w1899:i16)
                    n664 = Subtract(x=w1899, y=w1886) -> (x-y=w1889:i16)
                    n665 = Absolute Value(x=w1889) -> (abs(x)=w1885:i16)
                    n666 = Greater Or Equal?(x=w1885, y=w1898) -> (x >= y?=w1892:bool)
                    n667 = Less Or Equal?(x=w1885, y=w1890) -> (x <= y?=w1891:bool)
                    n668 = And(x=w1892, y=w1891) -> (x .and. y?=w1893:bool)
                    n669 = case shown="True" w1893 {
                      tunnel: w1900 -> [_ w1912]
                      tunnel: [w1907 w1912] -> w1897
                      tunnel: [w1908 w1918] -> w1896
                      tunnel: [w1908 w1918] -> w1895
                      tunnel: w1888 -> [w1907 _]
                      tunnel: w1885 -> [_ w1917]
                      tunnel: [u16 0 w1917] -> w1894
                      tunnel: w1883 -> [_ w1911]
                      frame False {
                        w1908 = FALSE
                        # "Don't Move"
                      }
                      frame True {
                        w1918 = TRUE
                        # "45 DEG MOUNT OFFSET"
                        # "1024/300"
                        # "Current Delta"
                        # "Use new Track Angle"
                        n670 = Divide(x=w1912, y=3.413333333333333) -> (x/y=w1914:dbl)
                        n671 = Negate(x=w1911) -> (-x=w1910:sgl)
                        n672 = Subtract(x=w1914, y=sgl 60.0) -> (x-y=w1916:dbl)
                        n673 = Add(x=w1916, y=w1910) -> (x+y=w1909:dbl)
                        n674 = local write "Last Track Angle - L"(w1909) -> ()
                      }
                    }
                  }
                }
                n675 = local read "Timeout to \nEnable Reactive Predict"() -> (w1865:u16)
                n676 = Less?(x=w1864, y=w1865) -> (x < y?=w1863:bool)
                n677 = case shown="True" w1863 {
                  tunnel: [enum16{"Track", "Reactive Predict", ""}."Reactive Predict" ("Initial Tracking State - Right") enum16{"Track", "Reactive Predict", ""}."Track" ("Initial Tracking State - Right")] -> w1862
                  frame False {
                  }
                  frame True {
                  }
                }
              }
              frame "Reactive Predict" {
                # "Choose New\nTracking State"
                n678 = Or(x=w1922, y=w1925) -> (x .or. y?=w1921:bool)
                n679 = case shown="False" w1921 {
                  tunnel: [w1951 w2003] -> w1938
                  tunnel: w1937 -> [w1950 _]
                  tunnel: w1936 -> [w1949 _]
                  tunnel: w1935 -> [w1948 _]
                  tunnel: w1934 -> [w1947 _]
                  tunnel: w1933 -> [w1946 _]
                  tunnel: w1931 -> [w1945 _]
                  tunnel: [w1944 w2002] -> w1930
                  tunnel: [w1943 w2002] -> w1928
                  tunnel: w1927 -> [w1942 _]
                  tunnel: [w1941 0] -> w1926
                  tunnel: [enum16{"Track", "Reactive Predict", ""}."Reactive Predict" ("Initial Tracking State - Right") enum16{"Track", "Reactive Predict", ""}."Track" ("Initial Tracking State - Right")] -> w1924
                  tunnel: w1932 -> [w1939 w2003]
                  frame False {
                    # "Stay in Reactive State"
                    # "Increment Track Timeout"
                    # "Move Respond Flag"
                    n680 = Increment(x=w1942) -> (x+1=w1941:i32)
                    n681 = case shown="True" w1946 {
                      tunnel: w1950 -> [_ w1966]
                      tunnel: w1949 -> [_ w1965]
                      tunnel: w1948 -> [_ w1964]
                      tunnel: w1947 -> [_ w1963]
                      tunnel: w1945 -> [_ w1960]
                      tunnel: [w1952 w1956] -> w1951
                      tunnel: [w1953 w1955] -> w1944
                      tunnel: [w1953 w1955] -> w1943
                      tunnel: w1939 -> [w1952 w1954]
                      frame False {
                        w1953 = FALSE
                        # "Reset Move Respond = F"
                        # "Move Servo = F"
                      }
                      frame True {
                        w1955 = TRUE
                        # "Position Lock"
                        # "Current Servo\nPosition"
                        # "Reset Move\nRespond = T"
                        # "Move Servo = T"
                        # "Apply Direction \nto Offset (delta sum)"
                        # "Check Last Known Position of Robot"
                        n682 = case shown="True" w1966 {
                          tunnel: w1965 -> [_ w1994]
                          tunnel: w1964 -> [_ w1969]
                          tunnel: w1963 -> [_ w1970]
                          tunnel: [sgl 1.0 ("y") w1968] -> w1962
                          frame False {
                            # "No Position Data Available"
                            # "Default is to move\nSame Direction as other\nServo"
                          }
                          frame True {
                            w1975 = sgl 1.0 ("y")
                            # "Use previous position/orientation to Guess Which Direction to Move Servo"
                            # "Choose Search Direction"
                            # "\"Perpendicular \nThreshold\""
                            # "If Orientation is\n ~Perpendicular -> Start Search\n in Opposite Direction of Other"
                            # "****add 90 until orientation angle is fixed"
                            # "Last Orientation"
                            # "Convert to Rad"
                            # "Avoid Divide by 0"
                            # "-1/m"
                            # "Calculate Normal Line to \nLast Robot Position\nfrom Center Beacon"
                            # "last Position \nCoordinates"
                            n683 = Unbundle(w1994) -> ("X"=w1974:sgl, "Y"=w1973:sgl)
                            n684 = Unbundle(w1970) -> ("X"=w1972:sgl, "Y"=w1971:sgl)
                            n685 = Subtract(x=w1973, y=w1971) -> (x-y=w1990:sgl)
                            n686 = Subtract(x=w1974, y=w1972) -> (x-y=w1988:sgl)
                            n687 = Equal To 0?(x=w1988) -> (x = 0?=w1989:bool)
                            n688 = case shown="False" w1989 {
                              tunnel: w1990 -> [w1997 _]
                              tunnel: w1988 -> [w1996 _]
                              tunnel: [w1995 1000000000000000.0] -> w1987
                              frame False {
                                n689 = Divide(x=w1997, y=w1996) -> (x/y=w1995:sgl)
                              }
                              frame True {
                              }
                            }
                            n690 = Equal To 0?(x=w1987) -> (x = 0?=w1992:bool)
                            n691 = case shown="False" w1992 {
                              tunnel: [w1999 1e-08] -> w1991
                              tunnel: w1987 -> [w1999 _]
                              frame False {
                              }
                              frame True {
                                # "Can't have infinit slope"
                              }
                            }
                            n692 = Divide(x=-1.0, y=w1991) -> (x/y=w1986:dbl)
                            n693 = Inverse Tangent(1:w1986) -> (0:w1984:dbl)
                            n694 = expression code="(x/pi)*180.0" "radians to degrees"(w1984) -> (w1985:dbl)
                            n695 = To Single Precision Float(number=w1985) -> (single precision float=w1982:sgl)
                            n696 = Add(x=w1969, y=sgl 90.0) -> (x+y=w1981:sgl)
                            n697 = Subtract(x=w1982, y=w1981) -> (x-y=w1980:sgl)
                            n698 = Absolute Value(x=w1980) -> (abs(x)=w1979:sgl)
                            n699 = Less Or Equal?(x=w1979, y=sgl 10.0) -> (x <= y?=w1977:bool)
                            n700 = Negate(x=w1975) -> (-x=w1976:sgl)
                            n701 = Select(t=w1976, s=w1977, f=w1975) -> (s? t:f=w1968:sgl)
                          }
                        }
                        n702 = To Word Integer(number=w1962) -> (16bit integer=w1961:i16)
                        n703 = Multiply(x=w1961, y=w1960) -> (x*y=w1959:i32)
                        n704 = To Word Integer(number=w1954) -> (16bit integer=w1958:i16)
                        n705 = Add(x=w1959, y=w1958) -> (x+y=w1957:i32)
                        n706 = To Unsigned Word Integer(number=w1957) -> (unsigned 16bit integer=w1956:u16)
                      }
                    }
                  }
                  frame True {
                    w2002 = TRUE
                    # "Go Directly to Track State"
                  }
                }
              }
            }
            n707 = local read "Tracking Timeout\nThreshold"() -> (w1846:i32)
            n708 = Less?(x=w1839, y=w1846) -> (x < y?=w1847:bool)
            n709 = case shown="False" w1847 {
              tunnel: [T2."Recovery Mode" ("Next Main State") T2."Tracking" ("Next Main State")] -> w1851
              frame False {
              }
              frame True {
              }
            }
          }
          frame "Recovery Mode" {
            w2014 = u16 0
            # "***Compltetly resets as of R17, used to just reset to \"Max Recovery Count - 1\""
            # "Increment Recoveyr Mode Count"
            # "Frames Processed"
            # "Choose Next Main State"
            # "Reset recovery count"
            # "Recovery move\nCount"
            # "Recovery Search\nAttempt count"
            # "Move Servo = T"
            # "delta move sum"
            # "Robot Position Valid"
            n710 = local read "Image Lock - Right"() -> (w2018:bool)
            n711 = Or(x=w2009, y=w2010) -> (x .or. y?=w2008:bool)
            n712 = case shown="\"Recovery Search\"" w2011 {
              tunnel: w2040 -> [_ _]
              tunnel: w2039 -> [_ _]
              tunnel: w2038 -> [_ _]
              tunnel: w2037 -> [_ _]
              tunnel: w2036 -> [_ _]
              tunnel: w2035 -> [_ _]
              tunnel: w2034 -> [w2068 w2154]
              tunnel: [w2060 w2152] -> w2033
              tunnel: [w2057 w2146] -> w2032
              tunnel: [FALSE FALSE] -> w2012
              tunnel: [w2062 w2143] -> w2031
              tunnel: w2028 -> [w2066 _]
              tunnel: w2030 -> [w2069 _]
              tunnel: w2029 -> [w2067 w2149]
              tunnel: [w2059 w2142] -> w2026
              tunnel: [w2058 w2142] -> w2027
              tunnel: w2018 -> [w2056 _]
              tunnel: [w2047 w2153] -> w2025
              tunnel: w2024 -> [w2045 w2137]
              tunnel: w2023 -> [w2050 w2150]
              tunnel: w2022 -> [w2046 w2148]
              tunnel: w2009 -> [_ _]
              tunnel: w2010 -> [_ w2145]
              tunnel: [FALSE w2144] -> w2020
              tunnel: w2017 -> [w2054 _]
              tunnel: w2016 -> [w2053 _]
              tunnel: [w2050 w2141] -> w2015
              frame "Recovery Search" {
                # "Wait for 2 Images to be Processed\nBefore Going to Next Step"
                # "Choose Next Reovery State"
                # "Recovery Search \nAttempt Count"
                # "Move Servo"
                # "Goal Position"
                # "Recovery Search\nmove Count"
                # "Attempt Recovery Search if Other Servo has Valid Angle"
                n713 = local read "Last Track Angle - R"() -> (w2049:sgl)
                n714 = Greater Or Equal?(x=w2045, y=w2046) -> (x >= y?=w2048:bool)
                n715 = case shown="True" w2048 {
                  tunnel: w2069 -> [_ w2089]
                  tunnel: [w2074 w2088] -> w2058
                  tunnel: w2068 -> [w2077 w2087]
                  tunnel: w2067 -> [_ w2086]
                  tunnel: [w2075 w2085] -> w2059
                  tunnel: [w2077 w2084] -> w2060
                  tunnel: [FALSE w2083] -> w2057
                  tunnel: w2054 -> [w2075 w2082]
                  tunnel: w2053 -> [w2074 w2081]
                  tunnel: w2056 -> [_ w2080]
                  tunnel: w2049 -> [_ w2079]
                  tunnel: [w2072 0 ("Frames Processed\nCount - in")] -> w2047
                  tunnel: w2045 -> [w2073 _]
                  frame False {
                    # "Increment Frames Processed"
                    # "WAIT"
                    n716 = Increment(x=w2073) -> (x+1=w2072:i32)
                  }
                  frame True {
                    n717 = case shown="True" w2080 {
                      tunnel: w2079 -> [_ w2102]
                      tunnel: w2082 -> [w2090 w2098]
                      tunnel: w2089 -> [_ w2103]
                      tunnel: [w2093 w2101] -> w2084
                      tunnel: [w2091 w2100] -> w2088
                      tunnel: w2081 -> [w2091 w2099]
                      tunnel: w2087 -> [w2093 w2097]
                      tunnel: w2086 -> [_ w2096]
                      tunnel: [FALSE TRUE] -> w2083
                      tunnel: [w2090 w2094] -> w2085
                      frame False {
                        # "Don't Move bc Other Servo Doesn't Have Image Lock"
                      }
                      frame True {
                        # "Move Servo = T"
                        n718 = Greater Than 0?(x=w2098) -> (x > 0?=w2104:bool)
                        n719 = case shown="False" w2104 {
                          tunnel: w2103 -> [w2111 _]
                          tunnel: w2102 -> [w2105 _]
                          tunnel: [w2110 w2121] -> w2101
                          tunnel: [w2108 w2127] -> w2100
                          tunnel: w2099 -> [w2109 w2127]
                          tunnel: w2098 -> [w2107 w2124]
                          tunnel: [w2106 w2126] -> w2094
                          tunnel: w2097 -> [_ w2122]
                          tunnel: w2096 -> [_ w2119]
                          frame False {
                            # "Increment move count to transition\nto Pan mode"
                            # "Increment Recovery Search Attempt Count"
                            # "1024/300"
                            # "Move Parallel to Other Servo"
                            n720 = Increment(x=w2109) -> (x+1=w2108:i32)
                            n721 = Add(x=w2105, y=w2111) -> (x+y=w2117:sgl)
                            n722 = Add(x=w2117, y=sgl 60.0) -> (x+y=w2116:sgl)
                            n723 = Multiply(x=3.413333333333333, y=w2116) -> (x*y=w2114:dbl)
                            n724 = Add(x=0.5, y=w2114) -> (x+y=w2112:dbl)
                            n725 = To Unsigned Word Integer(number=w2112) -> (unsigned 16bit integer=w2110:u16)
                            n726 = Increment(x=w2107) -> (x+1=w2106:i32)
                          }
                          frame True {
                            # "Apply Direction"
                            # "Step SIze"
                            # "Current Position"
                            # "Attempt to Pan in Steps Towards other Servo"
                            # "Could be same or function of \nregular search step size"
                            # "Max # of Pan\nMoves"
                            # "Pan Towards Other Servo"
                            n727 = Greater Or Equal?(x=w2124, y=u16 20) -> (x >= y?=w2125:bool)
                            n728 = case shown="False" w2125 {
                              tunnel: w2124 -> [w2135 _]
                              tunnel: [w2134 u16 0] -> w2126
                              frame False {
                                # "Increment Pan Count"
                                n729 = Increment(x=w2135) -> (x+1=w2134:i32)
                              }
                              frame True {
                                # "Reset move count"
                              }
                            }
                            n730 = local read "Recovery Search\nDirection - L"() -> (w2120:bool)
                            n731 = case shown="False" w2120 {
                              tunnel: w2122 -> [w2129 w2133]
                              tunnel: w2119 -> [w2130 w2132]
                              tunnel: [w2128 w2131] -> w2121
                              frame False {
                                # "CCW"
                                n732 = Add(x=w2129, y=w2130) -> (x+y=w2128:u16)
                              }
                              frame True {
                                # "CW"
                                n733 = Subtract(x=w2133, y=w2132) -> (x-y=w2131:u16)
                              }
                            }
                          }
                        }
                      }
                    }
                  }
                }
                n734 = local read "Max Recovery Count\n(Recovery Search)"() -> (w2051:u16)
                n735 = local read "Max Recovery\nSearch Attempts"() -> (w2052:u16)
                n736 = Less Or Equal?(x=w2058, y=w2052) -> (x <= y?=w2064:bool)
                n737 = Less Or Equal?(x=w2066, y=w2051) -> (x <= y?=w2065:bool)
                n738 = And(x=w2064, y=w2065) -> (x .and. y?=w2063:bool)
                n739 = case shown="True" w2063 {
                  tunnel: [enum16{"Generic Sweep", "Recovery Search"}."Generic Sweep" enum16{"Generic Sweep", "Recovery Search"}."Recovery Search"] -> w2062
                  frame False {
                  }
                  frame True {
                  }
                }
              }
              frame "Generic Sweep" {
                w2142 = u16 0
                # "Angle Valid?"
                # "Choose Next Recovery State"
                # "Wait for 2 Images to be Processed\nBefore Going to Next Step"
                # "New Goal Position"
                # "Move Servo"
                # "Frames Processed Count"
                n740 = Greater Or Equal?(x=w2137, y=w2148) -> (x >= y?=w2155:bool)
                n741 = case shown="True" w2155 {
                  tunnel: w2154 -> [w2171 w2183]
                  tunnel: w2149 -> [_ w2181]
                  tunnel: w2150 -> [w2170 w2180]
                  tunnel: [w2171 w2177] -> w2152
                  tunnel: [w2169 0] -> w2153
                  tunnel: [FALSE TRUE] -> w2147
                  tunnel: w2137 -> [w2172 _]
                  tunnel: [w2170 w2174] -> w2141
                  frame False {
                    # "Increment Frames Processed"
                    n742 = Increment(x=w2172) -> (x+1=w2169:i32)
                  }
                  frame True {
                    # "Reset Frames\nProcessed Count"
                    # "SWEEP SEARCH - Startup"
                    # "Multiple New Step\nby Step SIze"
                    # "F = CCW\nT = CW"
                    # "Last Direction"
                    # "Min Step"
                    # "add 10 in case\nactual position\nis lower than GP"
                    # "Set New Step #"
                    # "Choose Direction"
                    # "Nearest step"
                    # "Adjust Actual Posiiton\n to pre-determiend steps"
                    # "Move Servo 1 \"Step\" to\nSearch"
                    n743 = Add(x=5, y=w2183) -> (x+y=w2189:i32)
                    n744 = Quotient & Remainder(x=w2189, y=w2181) -> (floor(x/y)=w2187:i32)  [unwired: 1 out]
                    n745 = To Byte Integer(number=w2187) -> (8bit integer=w2178:i8)
                    n746 = Less?(x=w2178, y=1) -> (x < y?=w2184:bool)
                    n747 = case shown="False" w2184 {
                      tunnel: w2178 -> [w2200 w2208]
                      tunnel: [w2202 FALSE] -> w2174
                      tunnel: [w2201 w2208] -> w2186
                      tunnel: w2180 -> [w2199 _]
                      tunnel: w2181 -> [w2197 _]
                      frame False {
                        # "Max Step"
                        # "# of steps\nminus 1"
                        n748 = Divide(x=1024, y=w2197) -> (x/y=w2194:dbl)
                        n749 = To Unsigned Byte Integer(number=w2194) -> (unsigned 8bit integer=w2195:u8)
                        n750 = Greater Or Equal?(x=w2200, y=w2195) -> (x >= y?=w2196:bool)
                        n751 = case shown="True" w2196 {
                          tunnel: [w2203 TRUE] -> w2202
                          tunnel: [w2204 w2205] -> w2201
                          tunnel: w2200 -> [w2204 w2205]
                          tunnel: w2199 -> [w2203 _]
                          frame False {
                            # "No Need to\nChange Direction"
                          }
                          frame True {
                            # "T"
                            # "Move CW"
                          }
                        }
                      }
                      frame True {
                        # "F"
                        # "Move CCW"
                      }
                    }
                    n752 = case shown="True" w2174 {
                      tunnel: w2186 -> [w2191 w2192]
                      tunnel: [w2190 w2193] -> w2182
                      frame False {
                        # "CCW\n+1"
                        n753 = Increment(x=w2191) -> (x+1=w2190:i8)
                      }
                      frame True {
                        # "CW\n-1"
                        n754 = Decrement(x=w2192) -> (x-1=w2193:i8)
                      }
                    }
                    n755 = Multiply(x=w2182, y=w2181) -> (x*y=w2179:u16)
                    n756 = To Unsigned Word Integer(number=w2179) -> (unsigned 16bit integer=w2177:u16)
                  }
                }
                n757 = local read "Track Angle Valid  - Right"() -> (w2140:bool)
                n758 = local read "Image Lock - Right"() -> (w2139:bool)
                n759 = Or(x=w2139, y=w2140) -> (x .or. y?=w2138:bool)
                n760 = case shown="False" w2145 {
                  tunnel: [w2158 w2168] -> w2146
                  tunnel: w2147 -> [w2159 _]
                  tunnel: [w2160 enum16{"Generic Sweep", "Recovery Search"}."Generic Sweep"] -> w2143
                  tunnel: [w2157 w2168] -> w2144
                  tunnel: w2138 -> [w2156 _]
                  frame False {
                    # "Is other servo tracking?"
                    n761 = case shown="True" w2156 {
                      tunnel: [enum16{"Generic Sweep", "Recovery Search"}."Generic Sweep" enum16{"Generic Sweep", "Recovery Search"}."Recovery Search"] -> w2160
                      tunnel: w2159 -> [w2163 _]
                      tunnel: [w2163 FALSE] -> w2158
                      tunnel: [FALSE TRUE] -> w2157
                      frame False {
                        # "Stay in Sweep"
                      }
                      frame True {
                        # "G o to Recovery Search  State"
                      }
                    }
                  }
                  frame True {
                    w2168 = FALSE
                    # "Override Move Servo\nCommand bc an Angle Was Found\nduring this Step"
                    # "Stay In Sweep\nLet Main State Machine transition\ninto Tracking"
                  }
                }
              }
            }
            n762 = Increment(x=w2028) -> (x+1=w2007:i32)
            n763 = case shown="True" w2020 {
              tunnel: w2007 -> [w2043 _]
              tunnel: [w2043 0] -> w2021
              frame False {
              }
              frame True {
              }
            }
            n764 = case shown="False" w2008 {
              tunnel: [T2."Recovery Mode" ("Next Main State") T2."Tracking" ("Next Main State")] -> w2019
              frame False {
              }
              frame True {
              }
            }
          }
        }
        "Current Move Delta - L" <- w1734
        n765 = Less?(x=w1761, y=w1760) -> (x < y?=w1759:bool)
        n766 = local write "New Data  Flag\nLeft Servo"(FALSE) -> ()
        n767 = Select(t=w1760, s=w1759, f=w1761) -> (s? t:f=w1756:u16)
        n768 = Greater?(x=w1756, y=w1757) -> (0:w1758:bool)
        n769 = Select(t=w1757, s=w1758, f=w1756) -> (s? t:f=w1755:u16)
      }
    }
    "Next Main State - Left" <- w1162
    "Next Tracking State - Left" <- w1145
    "Next Recovery State - Left" <- w1143
    n770 = flat-sequence {
      tunnel: w1188 -> [w2215]
      tunnel: w1115 -> [w2214]
      tunnel: w1189 -> [w2217]
      tunnel: w1104 -> [w2216]
      tunnel: [w2215] -> w1202
      tunnel: [w2214] -> w1201
      tunnel: w1202 -> [w2223]
      tunnel: [w2222] -> w1197
      tunnel: [w2221] -> w1198
      tunnel: w1201 -> [w2220]
      frame #0 {
        # "Only Update GP if Moving Servo"
        n771 = case shown="True" w2215 {
          tunnel: w2217 -> [_ w2219]
          frame False {
          }
          frame True {
            # "Update Goal Position"
            n772 = local write "Servo Goal Position\n - Left"(w2219) -> ()
          }
        }
        n773 = case shown="True" w2214 {
          tunnel: w2216 -> [_ w2218]
          frame False {
          }
          frame True {
            # "New Direction"
            # "Update Goal Position"
            # "Update Direction"
            n774 = local write "Servo Goal Position\n - Right"(w2218) -> ()
          }
        }
      }
      frame #1 {
        # "Allow Comm Process to Take Down the Flag\nOnly Raise if not already in motion"
        n775 = local read "Servo Moving - R"() -> (w2228:bool)
        n776 = local read "Servo Moving - L"() -> (w2225:bool)
        n777 = local read "Move Servo - L"() -> (w2224:bool)
        n778 = local read "Move Servo - R"() -> (w2231:bool)
        n779 = Not(x=w2228) -> (.not. x?=w2230:bool)
        n780 = Not(x=w2225) -> (.not. x?=w2227:bool)
        n781 = And(x=w2220, y=w2230) -> (x .and. y?=w2229:bool)
        n782 = And(x=w2223, y=w2227) -> (x .and. y?=w2226:bool)
        n783 = case shown="True" w2229 {
          selector: w2229 -> [_ w2233]
          tunnel: [w2232 w2233] -> w2221
          tunnel: w2231 -> [w2232 _]
          frame False {
          }
          frame True {
          }
        }
        n784 = case shown="False" w2226 {
          selector: w2226 -> [_ w2235]
          tunnel: [w2234 w2235] -> w2222
          tunnel: w2224 -> [w2234 _]
          frame False {
          }
          frame True {
          }
        }
        n785 = local write "Move Servo - R"(w2221) -> ()
        n786 = local write "Move Servo - L"(w2222) -> ()
      }
    }
    n787 = local read "Current Main State - Right"() -> (w1167:T2)
    n788 = local read "Current Main State - Left"() -> (w1168:T2)
    n789 = Equal?(x=w1168, y=w1166) -> (x = y?=w1165:bool)
    n790 = Equal?(x=w1167, y=w1166) -> (x = y?=w1164:bool)
    n791 = And(x=w1165, y=w1197) -> (x .and. y?=w1193:bool)
    n792 = And(x=w1198, y=w1164) -> (x .and. y?=w1194:bool)
    n793 = And(x=w1165, y=w1164) -> (x .and. y?=w1192:bool)
    n794 = Exclusive Or(1:w1194, 2:w1193) -> (0:w1191:bool)
    n795 = case shown="True" w1191 {
      tunnel: [w2246 w2267] -> w1199
      tunnel: [w2247 w2266] -> w1195
      tunnel: w1114 -> [_ w2270]
      tunnel: w1155 -> [w2244 w2271]
      tunnel: w1118 -> [w2242 w2269]
      tunnel: [w2245 w2257] -> w1196
      tunnel: [w2243 w2256] -> w1200
      tunnel: w1163 -> [_ w2268]
      tunnel: w1192 -> [w2241 _]
      tunnel: w1193 -> [_ w2267]
      tunnel: w1194 -> [_ w2266]
      frame False {
        n796 = case shown="False" w2241 {
          tunnel: [w2251 w2253] -> w2247
          tunnel: [w2250 w2253] -> w2246
          tunnel: [w2249 w2252] -> w2245
          tunnel: w2244 -> [w2249 _]
          tunnel: [w2248 w2252] -> w2243
          tunnel: w2242 -> [w2248 _]
          frame False {
            # "No Movement\nRetain All Values"
            n797 = local read "Move Respond - L"() -> (w2251:bool)
            n798 = local read "Move Respond - R"() -> (w2250:bool)
          }
          frame True {
            w2252 = i16 0
            w2253 = FALSE
            # "Reset Delta Move sum\nfor both"
            # "F"
            # "Both Moved,\nMake Flags False"
          }
        }
      }
      frame True {
        w2263 = 200 ("y")
        w2254 = -200 ("y")
        # "Add/Clear Sum for \nServo That didn't move"
        # "Update Moving Servo's  Delta Position"
        # "if one Servo Moves, other should \nmove too eventually,\nUsed in Search Process"
        # "Only 1 Servo is Moving Due to Tracking --> Update delta move sum"
        n799 = case shown="True" w2266 {
          tunnel: w2271 -> [_ w2279]
          tunnel: w2270 -> [_ w2278]
          tunnel: [i16 0 w2277] -> w2264
          frame False {
          }
          frame True {
            n800 = Add(x=w2279, y=w2278) -> (x+y=w2277:i32)
          }
        }
        n801 = case shown="True" w2267 {
          tunnel: w2269 -> [_ w2275]
          tunnel: w2268 -> [_ w2274]
          tunnel: [i16 0 w2273] -> w2261
          frame False {
          }
          frame True {
            n802 = Add(x=w2275, y=w2274) -> (x+y=w2273:i32)
          }
        }
        n803 = Greater?(x=w2264, y=w2263) -> (0:w2265:bool)
        n804 = Greater?(x=w2261, y=w2263) -> (0:w2262:bool)
        n805 = Select(t=w2263, s=w2262, f=w2261) -> (s? t:f=w2258:i32)
        n806 = Select(t=w2263, s=w2265, f=w2264) -> (s? t:f=w2259:i32)
        n807 = Greater?(x=w2259, y=w2254) -> (0:w2255:bool)
        n808 = Greater?(x=w2258, y=w2254) -> (0:w2260:bool)
        n809 = Select(t=w2258, s=w2260, f=w2254) -> (s? t:f=w2256:i32)
        n810 = Select(t=w2259, s=w2255, f=w2254) -> (s? t:f=w2257:i32)
      }
    }
    n811 = case shown="True" w1110 {
      selector: w1110 -> [_ w2213]
      tunnel: [w2210 w2212] -> w1150
      tunnel: [w2209 i16 0] -> w1151
      tunnel: w1199 -> [w2210 _]
      tunnel: w1200 -> [w2209 _]
      frame False {
      }
      frame True {
        n812 = Not(x=w2213) -> (.not. x?=w2212:bool)
      }
    }
    "Move Respond - R" <- w1150
    "deltaMoveServo\n- R" <- w1151
    n813 = case shown="False" w1161 {
      selector: w1161 -> [_ w2240]
      tunnel: [w2237 w2239] -> w1153
      tunnel: [w2236 i16 0] -> w1156
      tunnel: w1195 -> [w2237 _]
      tunnel: w1196 -> [w2236 _]
      frame False {
      }
      frame True {
        n814 = Not(x=w2240) -> (.not. x?=w2239:bool)
      }
    }
    "Move Respond - L" <- w1153
    "deltaMoveServo\n- L" <- w1156
    "Current Main State - Left" <- w1187
    "Frames Processed\nCount - in -L" <- w1179
    "Recovery Mode Count - in Left" <- w1174
    "Recovery Search\nmove Count - in - L" <- w1173
    "Recovery Search\nAttempt Count - in - L" <- w1172
    "Current Main State - Right" <- w1141
    "Frames Processed\nCount - in Right" <- w1124
    "Recovery Search\nmove Count - Right" <- w1126
    "Recovery Search\nAttempt Count - Right" <- w1125
    "Recovery Mode Count in Right" <- w1117
    "Tracking Timeout\nCount - L" <- w1148
    "Tracking Timeout\nCount - R" <- w1133
    "Current Tracking State - Left" <- w1147
    "Current Tracking State - Right 2" <- w1139
    "Current Recovery State - Right" <- w1140
    "Current Recovery State -L" <- w1144
  }
